vi "WVDIAL_2_OphirPM_v2.2_temp_tune.vi"() -> ()   [LabVIEW 2012]
uses:
  <vilib>/DAQmx/write.llb/DAQmx Write (Digital 1D Bool NChan 1Samp 1Line).vi
  <vilib>/DAQmx/miscellaneous.llb/DAQmx Fill In Error Info.vi
  under_development/AMCS_Data.vi
  <vilib>/Analysis/baseanly.llb/Mean (DBL).vi
  H2O_DIAL/LabVIEW-2012/Scalar_Data.vi
  H2O_DIAL/LabVIEW-2012/Bristol WM V2_31b/CLDevIFace.dll
  <vilib>/Analysis/NI_AALBase.lvlib
panel:
  out "AMCS_Profile":i32=423938
  out "FileHour":i32=21
  out "L_Count":i32=55
  out "sigma_off_total":dbl[](array[numeric])=[4.643764478525789e-25, 4.614054089008885e-25, 4.584505239124867e-25, 4.555117711360031e-25, 4.525891281920628e-25, 4.496825720864026e-25, 4.4679207921346825e-25, 4.43917625363397e-25, 4.410591857279519e-25, 4.382167349086702e-25, 4.353902469221332e-25, 4.325796952070131e-25, 4.297850526319035e-25, 4.270062915003385e-25, 4.2424338355941755e-25, 4.21496300005555e-25, 4.187650114911694e-25, 4.160494881312817e-25, 4.133496995114222e-25, 4.10665614692786e-25, 4.079972022208119e-25, 4.0534443013005885e-25, 4.0270726595130557e-25, 4.0008567671863953e-25, 3.9747962897506563e-25, 3.948890887799126e-25, 3.923140217138123e-25, 3.8975439288624596e-25, 3.872101669423651e-25, 3.8468130806556615e-25, 3.8216777998733165e-25, 3.796695459918264e-25, 3.771865689214647e-25, 3.7471881118146976e-25, 3.7226623474847904e-25, 3.698288011738762e-25, 3.674064715881081e-25, 3.6499920670996217e-25, 3.626069668468178e-25, 3.602297119029483e-25, 3.5786740138468807e-25, 3.555199944025038e-25, 3.531874496780442e-25, 3.508697255483564e-25, 3.4856677996831964e-25, 3.462785705191059e-25, 3.440050544069148e-25, 3.41746188471553e-25, 3.3950192918949573e-25, 3.3727223267433067e-25, 3.350570546849384e-25, 3.3285635062685348e-25, 3.306700755546275e-25, 3.2849818417818464e-25, 3.2634063086181134e-25, 3.2419736963135166e-25, 3.2206835417447437e-25, 3.1995353784347226e-25, 3.178528736595472e-25, 3.1576631431460264e-25, 3.136938121710331e-25, 3.1163531926889047e-25, 3.0959078732359584e-25, 3.0756016773038813e-25, 3.0554341156586187e-25, 3.0354046958827905e-25, 3.0155129224057757e-25, 2.995758296523749e-25, 2.976140316396684e-25, 2.956658477076711e-25, 2.937312270508894e-25, 2.9181011855453255e-25, 2.8990247079637847e-25, 2.8800823204609833e-25, 2.8612735026590936e-25, 2.8425977311370583e-25, 2.824054479409753e-25, 2.8056432179446445e-25, 2.7873634141536925e-25, 2.7692145324124604e-25, 2.751196034045025e-25, 2.733307377340114e-25, 2.7155480175403066e-25, 2.697917406837425e-25, 2.6804149943858566e-25, 2.6630402262774586e-25, 2.6457925455661677e-25, 2.6286713922280107e-25, 2.6116762031845402e-25, 2.594806412296848e-25, 2.5780614503242897e-25, 2.5614407449651105e-25, 2.5449437208048386e-25, 2.5285697993381813e-25, 2.5123183989456577e-25, 2.4961889348824045e-25, 2.4801808192712767e-25, 2.464293461079702e-25, 2.4485262661369243e-25, 2.432878637089962e-25, 2.4173499733996907e-25, 2.401939671334805e-25, 2.3866471239444233e-25, 2.3714717210600145e-25, 2.3564128492636686e-25, 2.3414698918824553e-25, 2.3266422289643866e-25, 2.3119292372725023e-25, 2.2973302902539466e-25, 2.2828447580263785e-25, 2.268472007381932e-25, 2.254211401719836e-25, 2.240062301084126e-25, 2.226024062100116e-25, 2.212096037982056e-25, 2.198277578493862e-25, 2.1845680299420055e-25, 2.170966735142683e-25, 2.1574730334212e-25, 2.1440862605623073e-25, 2.1308057488112046e-25, 2.117630826839664e-25, 2.1045608197172205e-25, 2.0915950489043225e-25, 2.078732832232995e-25, 2.0659734838290317e-25, 2.0533163141598343e-25, 2.0407606299680385e-25, 2.0283057342632226e-25, 2.0159509262467982e-25, 2.0036955013794794e-25, 1.9915387512419972e-25, 1.9794799636048e-25, 1.967518422328947e-25, 1.9556534073675992e-25, 1.9438841947549892e-25, 1.9322100564956178e-25, 1.920630260637019e-25, 1.9091440711521815e-25, 1.8977507479510996e-25, 1.8864495468332108e-25, 1.8752397194377075e-25, 1.8641205132176874e-25, 1.85309117138839e-25, 1.842150932893969e-25, 1.8312990323947193e-25, 1.8205347001558067e-25, 1.809857162063116e-25, 1.7992656395150586e-25, 1.7887593494647524e-25, 1.778337504265391e-25, 1.7679993116519135e-25, 1.7577439747484068e-25, 1.7475706919047535e-25, 1.7374786567250477e-25, 1.7274670579202631e-25, 1.717535079320341e-25, 1.707681899765072e-25, 1.697906693041456e-25, 1.6882086278066873e-25, 1.678586867468332e-25, 1.669040570230428e-25, 1.6595688888336423e-25, 1.650170970602582e-25, 1.6408459573091302e-25, 1.6315929850696558e-25, 1.6224111842310663e-25, 1.6132996793032208e-25, 1.6042575888772121e-25, 1.5952840254274042e-25, 1.5863780952670232e-25, 1.5775388984249963e-25, 1.5687655284818781e-25, 1.5600570725121137e-25, 1.5514126108612298e-25, 1.5428312171529566e-25, 1.534311957966347e-25, 1.5258538929082173e-25, 1.5174560742476717e-25, 1.5091175469739927e-25, 1.5008373485458013e-25, 1.4926145086791297e-25, 1.4844480493302943e-25, 1.4763369844272314e-25, 1.468280319798211e-25, 1.4602770529521724e-25, 1.452326172944243e-25, 1.4444266601595768e-25, 1.4365774862349533e-25, 1.4287776138376983e-25, 1.4210259966100612e-25, 1.4133215788036764e-25, 1.4056632953286864e-25, 1.3980500715375963e-25, 1.3904808229973073e-25, 1.38295445546765e-25, 1.3754698646759526e-25, 1.3680259363191862e-25, 1.36062154573811e-25, 1.3532555580103542e-25, 1.3459268276849692e-25, 1.3386341988195482e-25, 1.3313765048231232e-25, 1.3241525685254664e-25, 1.3169612019618072e-25, 1.3098012064815228e-25, 1.3026713726028247e-25, 1.2955704802645196e-25, 1.2884972986337452e-25, 1.281450586258092e-25, 1.2744290912136427e-25, 1.2674315511209394e-25, 1.2604566934571265e-25, 1.2535032355813504e-25, 1.246569884883568e-25, 1.2396553393298492e-25, 1.2327582875898557e-25, 1.2258774092414679e-25, 1.219011375458982e-25, 1.2121588491226e-25, 1.2053184854101307e-25, 1.1984889325828062e-25, 1.1916688319567769e-25, 1.1848568191243869e-25, 1.178051524299784e-25, 1.1712515731126608e-25, 1.1644555874741191e-25, 1.1576621864375854e-25, 1.1508699868736606e-25, 1.1440776047568059e-25, 1.137283656132748e-25, 1.1304867581494259e-25, 1.1236855301332552e-25, 1.1168785951747307e-25, 1.1100645810052044e-25, 1.1032421216270046e-25, 1.0964098589464416e-25, 1.0895664437392028e-25, 1.0827105377761497e-25, 1.0758408152001282e-25, 1.068955964128544e-25, 1.062054688828481e-25, 1.055135711160854e-25, 1.0481977726805562e-25, 1.0412396366003204e-25, 1.0342600898105731e-25, 1.027257944842442e-25, 1.0202320419826945e-25, 1.0131812517790627e-25, 1.0061044766845727e-25, 9.990006537566844e-26, 9.918687569493606e-26, 9.8470779905946e-26, 9.775168344172793e-26, 9.702949608562794e-26, 9.630413227010019e-26, 9.557551122277968e-26, 9.484355729177786e-26, 9.410820011448697e-26, 9.336937490265801e-26, 9.262702260371961e-26, 9.188109020809214e-26, 9.11315308869798e-26, 9.037830427761936e-26, 8.962137666462638e-26, 8.88607211673616e-26, 8.809631794749932e-26, 8.732815442451108e-26, 8.655622537484813e-26, 8.578053318660534e-26, 8.500108793558888e-26, 8.421790757035365e-26, 8.343101802299517e-26, 8.26404533202396e-26, 8.184625569595185e-26]
  out "sigma_on_total":dbl[](array[numeric])=[1.7075862122244e-23, 1.7004426742837037e-23, 1.693239609744741e-23, 1.6859783954253323e-23, 1.678660410820497e-23, 1.6712870375550727e-23, 1.6638596588086796e-23, 1.656379658679081e-23, 1.6488484214502813e-23, 1.6412673312498138e-23, 1.6336377713340953e-23, 1.625961123487383e-23, 1.6182387675681657e-23, 1.6104720808587064e-23, 1.602662437665621e-23, 1.5948112086218224e-23, 1.586919760240094e-23, 1.5789894545108264e-23, 1.5710216482381445e-23, 1.5630176926607628e-23, 1.5549789329817173e-23, 1.546906707842516e-23, 1.5388023489784623e-23, 1.530667180683284e-23, 1.5225025193879302e-23, 1.5143096734187747e-23, 1.5060899422993675e-23, 1.4978446166673147e-23, 1.4895749777683752e-23, 1.4812822969984015e-23, 1.4729678357888077e-23, 1.464632845041312e-23, 1.4562785649718562e-23, 1.447906224670939e-23, 1.4395170419387456e-23, 1.431112222903883e-23, 1.4226929617854445e-23, 1.4142604406027486e-23, 1.405815829025985e-23, 1.397360284014021e-23, 1.388894949657693e-23, 1.380420957002031e-23, 1.371939423785285e-23, 1.363451454285266e-23, 1.3549581391141818e-23, 1.3464605551189887e-23, 1.3379597651367873e-23, 1.3294568179486758e-23, 1.3209527481194656e-23, 1.312448575787998e-23, 1.3039453067745007e-23, 1.2954439322388221e-23, 1.2869454287169013e-23, 1.2784507581039522e-23, 1.2699608673775678e-23, 1.2614766888406229e-23, 1.252999139774802e-23, 1.2445291225817366e-23, 1.2360675247526299e-23, 1.2276152187304654e-23, 1.2191730619865334e-23, 1.2107418970164145e-23, 1.202322551315382e-23, 1.193915837419463e-23, 1.1855225528683853e-23, 1.177143480262109e-23, 1.1687793873793825e-23, 1.1604310270505038e-23, 1.1520991373461181e-23, 1.1437844415482158e-23, 1.1354876482938843e-23, 1.1272094515594521e-23, 1.1189505307343022e-23, 1.1107115508072479e-23, 1.1024931622616465e-23, 1.094296001379224e-23, 1.0861206901467108e-23, 1.0779678365135314e-23, 1.0698380343367289e-23, 1.06173186361969e-23, 1.0536498905450043e-23, 1.0455926676160623e-23, 1.0375607337759655e-23, 1.0295546145299345e-23, 1.0215748220460876e-23, 1.0136218553593378e-23, 1.0056962003784583e-23, 9.97798330145124e-24, 9.899287048722052e-24, 9.820877721811146e-24, 9.74275967122139e-24, 9.664937124155247e-24, 9.587414185725328e-24, 9.51019484042637e-24, 9.433282953390896e-24, 9.356682271669029e-24, 9.280396426675263e-24, 9.204428935016307e-24, 9.128783200260969e-24, 9.053462513813825e-24, 8.978470057602318e-24, 8.903808904957389e-24, 8.829482022184774e-24, 8.755492270140328e-24, 8.68184240623818e-24, 8.608535085372624e-24, 8.535572861930238e-24, 8.462958191150288e-24, 8.390693430702545e-24, 8.318780842469266e-24, 8.247222593903732e-24, 8.176020759597675e-24, 8.105177323247602e-24, 8.0346941779939e-24, 7.964573129989107e-24, 7.89481589772579e-24, 7.825424115173927e-24, 7.756399332508075e-24, 7.6877430180163e-24, 7.619456559217698e-24, 7.551541264744586e-24, 7.483998365445229e-24, 7.416829016422044e-24, 7.350034297741753e-24, 7.283615216447286e-24, 7.217572707624918e-24, 7.151907636193094e-24, 7.086620797948962e-24, 7.02171292149949e-24, 6.957184668579832e-24, 6.893036636834266e-24, 6.829269359936771e-24, 6.76588330962968e-24, 6.702878896700126e-24, 6.640256472626323e-24, 6.5780163306938516e-24, 6.516158706777594e-24, 6.4546837815950906e-24, 6.3935916809599384e-24, 6.332882477825005e-24, 6.272556192843959e-24, 6.212612795889849e-24, 6.153052207074656e-24, 6.0938742983743955e-24, 6.035078894147427e-24, 5.976665772122362e-24, 5.918634665719597e-24, 5.860985263481029e-24, 5.803717211502671e-24, 5.7468301138902555e-24, 5.6903235336624575e-24, 5.634196994214138e-24, 5.578449979752345e-24, 5.5230819371427534e-24, 5.468092275895874e-24, 5.413480369833808e-24, 5.359245557887875e-24, 5.305387144754368e-24, 5.251904401815032e-24, 5.198796568697882e-24, 5.146062853222409e-24, 5.0937024329285036e-24, 5.041714455530881e-24, 4.9900980398858834e-24, 4.938852277059481e-24, 4.887976230623468e-24, 4.83746893794503e-24, 4.787329410462798e-24, 4.737556635055691e-24, 4.688149574056101e-24, 4.639107166465834e-24, 4.5904283286634496e-24, 4.542111954867825e-24, 4.494156918056621e-24, 4.4465620704066765e-24, 4.399326243957229e-24, 4.352448251589667e-24, 4.305926887428094e-24, 4.259760927133192e-24, 4.213949129056238e-24, 4.168490234607401e-24, 4.12338296883391e-24, 4.07862604077928e-24, 4.034218144353722e-24, 3.990157958768539e-24, 3.946444149064885e-24, 3.9030753664335e-24, 3.860050249023712e-24, 3.817367422335441e-24, 3.7750254995106654e-24, 3.733023082193349e-24, 3.691358760512388e-24, 3.650031114008777e-24, 3.6090387117905654e-24, 3.5683801127861655e-24, 3.528053866803104e-24, 3.488058514122023e-24, 3.4483925866184155e-24, 3.409054607705317e-24, 3.370043092808114e-24, 3.331356549823639e-24, 3.2929934793979014e-24, 3.2549523754474237e-24, 3.217231725253417e-24, 3.179830009805838e-24, 3.1427457044565034e-24, 3.1059772789917302e-24, 3.0695231977134503e-24, 3.033381920449335e-24, 2.99755190191396e-24, 2.962031592850093e-24, 2.9268194397709086e-24, 2.8919138854636326e-24, 2.8573133691808308e-24, 2.8230163268299376e-24, 2.7890211914429353e-24, 2.7553263932755457e-24, 2.7219303599098855e-24, 2.688831516768636e-24, 2.656028287199601e-24, 2.6235190926969376e-24, 2.5913023529850115e-24, 2.5593764866235505e-24, 2.527739910619601e-24, 2.496391041275666e-24, 2.465328293863177e-24, 2.434550083004947e-24, 2.4040548229168003e-24, 2.373840927399175e-24, 2.3439068103705293e-24, 2.314250885433015e-24, 2.284871566748021e-24, 2.2557672684858724e-24, 2.2269364056176892e-24, 2.1983773934884902e-24, 2.170088648470371e-24, 2.1420685877073818e-24, 2.1143156295265137e-24, 2.0868281932439607e-24, 2.059604699720196e-24, 2.0326435711084415e-24, 2.0059432311343632e-24, 1.9795021052597507e-24, 1.9533186205922764e-24, 1.927391206342342e-24, 1.90171829343342e-24, 1.8762983150473395e-24, 1.851129706617593e-24, 1.8262109056432633e-24, 1.8015403521583982e-24, 1.7771164885857278e-24, 1.752937759959652e-24, 1.7290026138301698e-24, 1.705309500565543e-24, 1.6818568732524412e-24, 1.6586431878588544e-24, 1.6356669031809573e-24, 1.6129264812045587e-24, 1.5904203868386669e-24, 1.5681470881088427e-24, 1.5461050562990223e-24, 1.5242927659307277e-24, 1.5027086948226053e-24, 1.481351324147798e-24, 1.4602191385259846e-24, 1.439310626001592e-24, 1.4186242781334644e-24, 1.3981585901500172e-24, 1.3779120607809285e-24, 1.3578831924817317e-24, 1.3380704914055822e-24, 1.3184724673794015e-24, 1.2990876341133162e-24, 1.2799145090715568e-24, 1.2609516136104614e-24]
  out "background start":u32=269
  in  "Tab Control 2":enum32{"WV ND Narrow", "WV ND Wide"}(tab)
  out "Water Vapor Number Density":dbl[][](graph)=[[2.7919549800729766, 2.4721214980617963, 2.1963483034310913, 1.9775481743916468, 2.0259507247493356, 2.096592957954238, 2.09200685333887, 2.201465478284958, 2.172049757701778, 2.066356384667988, 2.1552068146500667, 2.142096979762263, 2.16074094077469, 2.1508543106624907, 2.063657397073414, 2.111120921818043, 1.9736927303840606, 1.9924659617468845, 1.8437447128387863, 1.716666972928834, 1.7329795721179366, 1.6185075270306553, 1.9531692944484582, 1.7270894741211513, 1.3541922429617665, 1.6972365264191616, 1.3780472464601408, 0.6352127824328955, 0.7449848462353037, 0.25739950222857966, 0.02150582751711, 1.2625193726213453, 1.7103366183498547, 1.1760098085538666, 0.952397569112398, 0.9602628838341002, 1.1470709594539148, 2.0260087466607244, 1.717397631037124, 0.45954812101467546, 0.82082018935899, 0.4578051259106563, 0.17693171656260112, 0.2294926614257034, 0.40695379752745414, 0.7260767006490062, 1.6299360111045522, 1.394016861417572, 1.260638353981884, 0.9565154264924587, 0.778518699153623, 1.1018278296017567, 1.9052590216943897, 2.1494434456810643, 3.1852092631635816, 3.50602861686196, 3.114069255143937, 1.9505136425814023, 0.6799674842963526, 1.4884495991309699, -0.13824046213613744, 2.835156534294972, 3.3505695354404685, 2.938366562214755, 6.438557108895117, 0.5183551787975594, 0.3153485302712685, 1.975534410314832, 2.3601361815003115, 5.779543708322931, 5.6862481890886425, -0.320178545767054, -3.752352207701061, -7.1478162896744895, -12.791206630214896, -7.216285577276, -3.118979952580519, 2.676212905498716, -0.09079217678994128, 0.8475995496768057, 7.5565978270016485, 4.031331088945062, 18.746473553929125, 9.019579967521627, 10.111126789878568, 10.911425895546724, 10.881486374798657, -4.867225785195253, 1.3613463436287887, -6.705643508234555, -9.400669767805649, -11.45672530581558, -15.476104692326604, 2.5019067005614284, 22.15558346925288, 12.372906343206774, 9.180179495997407, 10.035886348315783, -2.300504604887407, -6.109257874581613, 1.2443637131026353, 10.72505129453685, 14.876862757116449, -15.670760900032207, -31.77161023736102, -8.91609594784887, -9.583958414687443, -10.704114282385731, 5.617021746201043, 8.71662490415398, 7.943503644326281, 16.20179237317941, -14.236690656943491, 2.957594051298285, 28.71651223843686, -15.16894026062252, -14.342090655059778, -10.145491925129408, -13.950103926886067, -8.362096082265273, -23.276275045469802, -34.21186123581827, -14.624177385211423, 5.1900077381089815, -22.451944969117548, 9.280913616926904, -0.7349242905240464, -1.9056931662673575, -0.3552584964139418, 13.011816088431226, 2.388764514874305, -4.970348772024848, -5.374892740249347, -18.104796179616045, -3.7757407411406834, 0.2572912127569682, -9.101456890736229, -9.940691485699297, -16.220067449273007, -31.360968584433184, -13.22567737321429, 2.9847822496071443, 0.3000737204657703, 14.226487589262792, 6.624487648840693, -27.284491819792123, 24.242667346984188, 19.937023327511973, -6.324539592488602, -2.8041964118578786, 6.740823105858939, 23.587397969477554, -4.2833757162263355, -33.3154285684293, -35.55104995851804, 4.931666571921572, -8.427144388302073, -2.161849941643455, 31.006477690881464, 28.994847381319968, 9.739058874229096, 31.647398824516547, -9.49704103338363, -3.459829626087916, -10.195382957260902, -18.2305351963672, -39.16562759387119, -38.369889060589664, -33.57595009336855, -48.192728659126416, -34.0670225863149, -64.44616828322731, 22.052013009398934, 48.8882374543455, 47.82272047473126, 21.630359864857, 19.619480202360133, 16.248342826014856, 14.55626534124269, 16.14141319559857, 41.72682657704204, 2.358153419284582, -18.450444811942706, -16.453191933989043, -32.77707187251656, 8.079786828047531, -1.1358565341839377, 18.848376232966167, 8.60604014960662, 4.314367560106007, -13.03383243904803, 2.650659064146061, -4.009372086896625, -29.11960106159767, 0.12218354900213305, -39.711017849362754, -42.75783315079344, -30.018182143488808, -9.971368815385215, 31.54378511520024, 37.63564210589476, -76.9833397272995, -131.8510304950383, 39.46780422831733, 23.7601287553926, -35.38738552003143, 32.03435449229545, -19.69485879050221, -3.0917333259606874, -124.46237667041301, -9.002678693930125, 107.01528897422901, 92.48090288243313, -103.79898797554694, -17.675491202491813, 7.874533254057714, 10.524609447658822, 49.75758334212029, 99.07815475479066, 283.5278586000699, 32.971642390852686, -57.450561658578394, 2.4742562020355403, -64.91676229497271, -81.39557989000245, -68.41783168327089, -79.73478237233522, -60.1655084932687, -183.42488156186718, -250.65131530114368, -152.8606608195418, -45.235659006464026, -71.77006522559867, 69.05001410951006, -31.66224852865109, 51.09664282478717, 46.1035128986533, 36.62674413702954, 77.11160259361291, 78.91913357872623, 74.85307061263583, 57.82460870704682, 102.49351870849972, 108.47745264638517, 108.28296843951362, 80.18423693091486, 6.206295215311893, -25.774421868942422, 38.17790600761687, -37.18542234252088, 40.562292077560116, -10.06029995849638, -45.99779659499376, -76.52379698325059, -24.04739599121833, 7.138888554504087, 94.67361862363965, -20.953075063505143, 27.52883005249273, -43.94482761055022, -31.42891116550487, -59.110333442134035, 69.6709781086392, 69.74972907027177, -244.93614676570755, 66.01327113431867, -263.90594662785674, -176.74730262491283, 53.83886185827534, 177.42061263532574, 108.16924852096365, 193.11882731535258, 102.94954292738339, 85.55425867346395, 0.0, 0.0, 0.0, 0.0, 0.0, 0.0]]
  out "Water Vapor Number Density 2":dbl[][](graph)=[[1.9246774090646468, 2.1364801526718655, 2.3563460415698363, 2.437880160037196, 2.4699096457122773, 2.4513779438068592, 2.4212790327062246, 2.4149121010244667, 2.442684765460251, 2.4627579558093378, 2.425720637457262, 2.499208106949827, 2.5487327850901806, 2.416323533000658, 2.503718155028522, 2.6058329726220686, 2.4815743106251458, 2.764613689254371, 2.8761740069495296, 2.9483743931379394, 2.9544743325162677, 3.1794158502671084, 3.1939705775233973, 2.533885225518133, 5.023499890046839, 5.739889326755892, 7.992222757013449, 11.222739860114261, 13.410626739277465, 21.58391327063631, 26.618972753698802, 23.957314589009496, 13.627342397542513, -33.466783552051155, -31.322362431050404, -3.828090312037132, -22.82546710883033, -10.993941851667527, -9.72872074268521, -20.277080950586896, -10.923757163092711, -9.07636230339632, -8.15449746589819, -10.005103572388432, -7.68751749774677, -8.476357917870377, -8.409711355395942, -8.352416737405557, -10.812293275936563, -10.41513555533087, -11.31136062577575, -13.45042937386785, -33.3057348158326, -14.63420336195662, -9.376062674764945, -11.009338696090161, -9.223392851297126, -11.554322192812531, -19.386991636136848, -10.670640131714526, -6.126941067398296, -7.518439774394675, 16.26303016203163, -4.0325693834978615, -2.912247487056353, 2.439455899744925, 1.3136310339215345, 7.53017468726898, 19.354503059461745, 10.874858416208898, 5.884842201842596, 11.658075090740155, 10.63840673688868, 11.819813138077537, 7.821749325303154, 6.142757151705678, 5.990511287239049, 6.091428632318514, 4.133829631016586, 1.910373740863632, 2.812138534703024, 0.13240697681270577, -1.6539863211154304, 1.8124465284545117, -0.10209803300606486, 0.3873834385336532, 3.2825127417538034, -0.38206784826885704, 0.29108793649235654, 1.9734986497673108, 2.709688975560919, 3.937758253159303, 6.073548367509126, 5.57827633674878, 3.7256924825272715, 3.523348344651393, 2.1380698550049098, 0.9819285118748023, 0.7534956053683336, 1.958752445947795, 1.167700425578407, 2.821741044082525, 1.7904903289201626, -0.06699506335081942, 2.0828772273760388, 1.5528809734202558, -1.4814454333788867, -0.7987225616089674, -2.386278740227717, -4.10627162811292, 0.7960841223175821, -0.967223151556819, -2.7068052187970837, -0.8793538769734781, -1.6058994738614338, -1.153786976051838, -0.3772533844763944, -0.8321700075992845, 0.44162594879454903, 1.6775161023774172, 0.6144603786142944, 1.4748523477090723, 2.4261191491083633, -2.1637504157741003, -3.389739107572159, -1.336259563239183, 1.9457781147812288, 7.382876566090144, 7.012454908750662, 3.1710680875691533, -1.4266581436017785, -1.990855306154264, 1.8513905052490254, 6.224985812056048, 6.783669358850058, 2.503269835114906, 2.526890697902952, -0.15272259761902673, 1.166363050044734, 6.816656964463991, 5.817625584065743, 4.99042666662815, 5.578758228379871, 5.316718150893578, 2.2279403560959765, 3.6626378977623295, -2.7379426603799293, -4.168325740386166, -6.125245341748409, -5.986492361721819, -5.554924977572535, -4.33933044932571, -4.5079301433076795, -8.557458906008524, -5.194267813260687, -2.290162360446739, 3.189747404419548, 8.255852252066553, 9.969917789546885, 7.289797314084266, 4.129672688789654, 1.5019653264394026, 4.035196023759196, 3.620172660102847, 19.014751858086527, 6.4140881220414885, 1.6078436888032817, -4.9127663382774704, -13.431807716867139, -4.920859019873842, 0.11545557487235945, -2.418236722549294, -12.138276953308633, -13.944911735185746, -38.40034011695379, -12.768978114170004, -10.98559210913547, -8.071653207468731, 13.296674504094893, -6.570530262352096, 2.05649815926914, 0.27410650933140895, -7.566197720766897, 3.244758690591443, 11.479395171418595, -7.161105508606986, 12.337200345292445, 7.436389297750922, -2.8867984076459487, 26.508322141770208, -8.578118700603605, -4.812022100008427, 3.533689345937024, -8.142214281133004, 2.5937233186038475, 9.186142836001329, -15.684712280988862, -4.636866364119136, -7.5203674360960395, -21.093456852627572, 26.245939225341598, 32.12889135174122, 30.211214706937447, 49.64772783624668, 27.87193220400699, 8.478543192420785, 7.300517871932979, -11.241261216539064, -6.755589509893532, 0.1754162141842197, -40.87967308128872, -30.777993550416333, -25.110900077730392, -40.53025335927562, -16.147889968195557, -5.849042580416056, -42.062440862797764, -40.9461177020024, -48.30500611043761, -32.69072054873273, 4.3684891317049805, 40.5333176218133, 44.48163269384392, 16.266173328134716, -1.4034575775621692, -13.732735958483435, 35.50263552659409, 88.77461883984728, 65.81909954799848, 46.01099724751913, 29.966703800722787, -32.222515144215095, -39.001218416158856, -45.89663062841511, 10.24466871719786, 50.268932259400195, -121.68095976928211, -105.29974840543122, -56.18445992064484, -67.42947981632405, -15.455237158470073, 268.98749589285126, 208.26441201100153, 162.76795471812062, 1.9734940437567248, -218.48392140256198, 105.85362620395831, -64.0037301624681, -2.898047398837785, 21.380458202422382, 52.06570549270102, -248.8417906380732, -392.7522320975338, -215.35790079570805, 86.30117929847647, 159.14973379695226, 49.766972938901, 141.48970735229034, 1.7362457533596822, -0.14859597277129066, -98.66855973524312, 66.47378697642905, 236.04063498719637, 18.599802555423434, -99.43534896876382, 102.65886550601961, 73.36634300545326, -52.794667338550894, 36.1390490700412, 17.94640810403047, 34.13997149679165, -102.74220223926922, -65.7599054547175, 57.26872729966095, 0.0, 0.0, 0.0, 0.0, 0.0, 0.0]] caption="Water Vapor Number Density"
  out "RingBuffer offline near":dbl[][](array[numeric])
  out "RingBuffer aerosol near":dbl[][](array[numeric])
  in  "LOWER DISPLAY TAB":T1(tab)
  out "NRB":dbl[][](graph)=[[-3.800229408179693, -3.06314471671871, -2.586395001932205, -2.231941202363951, -1.9477207314219656, -1.7167397393646742, -1.5262035572526398, -1.364937464827194, -1.229462730809553, -1.118344000034183, -1.0283656358510886, -0.9561701019361557, -0.9025135206001915, -0.8627761462819167, -0.8360063278396849, -0.8198158981197357, -0.8061970293623525, -0.7877547408903874, -0.761226082248506, -0.7318531575391255, -0.7043247843183529, -0.6856829368303268, -0.6774945269892939, -0.6780969120898757, -0.6855795172986112, -0.697357082303388, -0.7090931326438995, -0.719243815964618, -0.7301383219859523, -0.7340834310039841, -0.7411956864780824, -0.7410369821935734, -0.7389788255998272, -0.7411397471378939, -0.7349219768039156, -0.7383642102319196, -0.7346077084773024, -0.7383309135731002, -0.7404822097283869, -0.7400029405093289, -0.7403653644838679, -0.7398416855657998, -0.7495371647323372, -0.7507436529256251, -0.7628558778510316, -0.7744574009887791, -0.772092035038182, -0.7826605939835732, -0.7906350425190564, -0.7911167128231053, -0.8047257605935517, -0.8208185277520433, -0.8319646227700381, -0.8377364399653591, -0.8425989844040539, -0.8513709082209938, -0.8614177662910704, -0.8912920570377314, -0.9248282024330806, -0.9432974574531058, -0.9415412810401951, -0.9310482734359397, -0.9338475158110462, -0.9134126868959206, -0.9283159986479004, -0.9145357579604514, -0.8898714875211668, -0.8875119944449646, -0.8828395041020582, -0.8987158344231726, -0.9189036361912808, -0.9646903803671855, -1.012629192189445, -1.04810081341131, -1.0803705713954739, -1.0793488392821509, -1.0810325197637765, -1.0860051215689395, -1.0919950348359535, -1.0970130303750192, -1.10050408499005, -1.1270957243331732, -1.153978655576542, -1.1759114974466267, -1.1814224007579102, -1.1478719628952656, -1.0881989873342564, -1.0434132693286031, -1.0423709416923355, -1.003167618084612, -1.0073219251996215, -1.0202371044894711, -1.0152974092249483, -1.1107576533946732, -1.1218686377231266, -1.2137096270649306, -1.2667171397873895, -1.1892934301718043, -1.195811506977401, -1.0821539130490045, -1.060475648708257, -1.0960067322895548, -1.1045852070482358, -1.205075147723515, -1.1710054544711102, -1.2279788860580556, -1.2235093993119002, -1.1920092242575382, -1.1837115303455092, -1.172287896788179, -1.246471942306521, -1.163648031500021, -1.084657739777487, -1.0421989912294563, -1.031853699648537, -1.1138724762093004, -1.1962195579732187, -1.2789690855557603, -1.2013419086769594, -1.1984463292291385, -1.2347319589311334, -1.0914307352170172, -1.119133066161212, -1.0951251916722085, -1.0796012629942673, -1.1660709765933723, -1.121190131602695, -1.1021885815228185, -1.1162886426649374, -1.1518589012525402, -1.235429403749575, -1.3843132921113361, -1.4984585580111909, -1.1477154649207388, -1.1408513656392523, -1.0889991084647108, -1.0498968077168733, -1.2217489272096793, -1.147493708380524, -1.1048199722886152, -1.0906745215855211, -1.1616096714779933, -1.231523831555943, -1.2084113515707662, -1.0485969917388265, -1.0028476315868609, -0.908153785166785, -0.9593826358961169, -1.1485410157950036, -1.1805752730290044, -1.4613637167632942, -1.5831274616304676, -1.8524697361245794, -1.902893297328939, -1.787245904046182, -1.9469806297270116, -2.4348078969799545, -1.5452467790031763, -1.5555715396865895, -1.6046204481754156, -1.4808715626314377, -1.3616849023984043, -1.2044986712945338, -1.0728427396250597, -1.1368391398220103, -1.102541352977231, -1.188264259019151, -1.2087675203831756, -1.0898031784234676, -1.0938247007935697, -0.9835556291746889, -0.9904433581700574, -1.0522941045778185, -1.0560752229787496, -1.2348032828788582, -1.334713764526752, -1.1978469831217804, -1.3608491709347206, -1.0667022430489146, -0.9399106674612636, -0.9876858594604188, -0.9662967753493834, -1.0825798056847127, -1.3239312272664043, -1.2163301583978723, -1.3333345454057624, -1.4132217678519643, -1.4325731565341893, -1.326699507831265, -1.1895532512336644, -1.357146633255645, -1.1092647584015825, -1.405175209074444, -2.071325145827588, -1.7178623977929357, -2.519985049968918, -1.8650910351271313, -1.1573432346808377, -0.9007453282372851, -0.8538828666401298, -0.8669195966399774, -1.0140790767546946, -1.4217368261424512, -1.0249565405120962, -0.9192498069458324, -0.842713087225846, -0.9210522507407414, -1.1768630172734111, -1.2843024988594796, -1.9010322059685716, -1.2202092243334877, -1.766166903525135, -2.203531076343693, -3.514732758163316, -1.1658588717362406, -2.8174425613600427, -1.7252934585275521, -1.4158596591803272, -1.0661722234590856, -1.3922611378291887, -1.8065419289783404, -2.012215811399121, -2.9418314791168347, -2.1050247884394424, -1.574790059832753, -2.077194149612097, -2.1648977087631036, -1.5196154156533368, -1.177386185168425, -1.0008246644603354, -1.1775246202068392, -1.1202978755017272, -1.044063384440292, -0.9858486216752352, -0.9637605673447708, -1.2184346489813616, -1.1987451492339647, -1.5260011819424544, -1.2610700135891226, -0.9215963998960293, -1.113154617357813, -1.1475896753447852, -1.1756020903233884, -1.7256144841358523, -1.5689993243779985, -1.4104165618981157, -1.3146217250936891, -1.5819863632077438, -1.0933708340070682, -1.2071394021218131, -1.2102078003428727, -1.184296563243633, -1.2357777799638099, -1.1743147216259175, -1.380206899498629, -1.447625287732161, -1.2721141475668638, -2.6438056872192366, -1.0704576216856974, -1.828565053490517, -1.3540195684640588, -1.211855498018374, -0.965407575543998, -1.5884933767947966, -1.0531141070130239, -0.9156713028909425, -0.8100547333672709, -1.3031843902511135, -1.3165366769540703, -1.4320177541670616, -1.6886772033069095, -1.5758186382249717, -1.1421971851539605, -1.1508373970493577, -1.690035290867579, -inf, -inf, -inf, -inf, -inf]] caption="Water Vapor Number Density"
  out "NRB 2":dbl[][](graph)=[[-3.0395188028357603, -2.3233310980260935, -1.908420723106076, -1.6302908440291224, -1.4282319836990602, -1.2744401657701292, -1.1539937154087423, -1.05853929608012, -0.9834427908474358, -0.9283287518597617, -0.8863581265636199, -0.8577551770624776, -0.8428705414502229, -0.8373210856679418, -0.8447938776035089, -0.8587365448043809, -0.873883515771329, -0.8813689723007432, -0.8774795693013318, -0.8677747815053004, -0.8600600847719546, -0.8595431314342655, -0.8681841305661355, -0.885390456771323, -0.9199774671108429, -0.9523346307996355, -0.9887639986348082, -1.0160536970759566, -1.0377506342413638, -1.0575136619828756, -1.0724721099288403, -1.1081309920793745, -1.114135072852424, -1.1355512982105995, -1.1392677172713934, -1.1467863183669873, -1.1658943701620241, -1.188161442926748, -1.2069892676099805, -1.2074612515550163, -1.2430546003808078, -1.2300970883816922, -1.298830352045476, -1.358703266826767, -1.3248852909188416, -1.3860187725636977, -1.3972398422909322, -1.4554774841562164, -1.5178491030527048, -1.564110781795938, -1.6220897936161092, -1.5208969542258364, -1.454348655100703, -1.4405921579344618, -1.4615070162429147, -1.4951291443274128, -1.7319565361894438, -1.969627795218796, -2.0771765277122363, -2.328544428787139, -1.8601381790747755, -1.8951962653608625, -1.7793115109813733, -2.255357804818516, -2.902967799437367, -2.421844110716655, -1.886647282120273, -2.0371230826274975, -2.1296353890888784, -2.203475639570752, -2.5685712448217277, -2.0033420248153524, -2.6169900639957655, -1.927542690509862, -1.405873961597174, -1.3259638684638195, -1.3539550277695553, -1.4242408794322738, -1.468918201419294, -1.4538280602853981, -1.3954212501136907, -1.305232269627442, -1.3344630238732782, -1.4740737469258944, -1.348804310360201, -1.5001521126592026, -1.389640446498644, -1.2250901251967545, -1.2913755968283593, -1.1235122884102886, -1.1483390918357013, -1.146495387943153, -1.1508242258903185, -1.229521881558638, -1.3304819849086533, -1.4452755544135947, -1.2762251214476263, -1.188234794912964, -1.0272788934356993, -1.0561195464317779, -1.1755054918408905, -1.1901794946288025, -1.331092466379116, -1.3164567545394104, -1.3490261692585808, -1.3440099621319015, -1.2577528142307361, -1.2561268962359338, -1.1410008073837692, -1.0676552929420373, -1.0705065775440905, -0.9949654137895192, -0.9602649895110492, -0.9858900749888218, -1.0894067873465203, -1.00682512703767, -1.0243095421701527, -0.9262744207006681, -1.0124226618520726, -0.9852318793179309, -1.0545828719090762, -1.3309862870720164, -1.0873613373156128, -1.41157121686751, -1.2176731494363078, -1.543541430165227, -1.6266424343497268, -1.4411568122747527, -1.4038460927505363, -0.9525486962136351, -0.9710054049772678, -0.830230618685657, -0.9424523281840133, -0.8645246633140569, -0.8732983037287279, -1.0361607688951742, -0.8809275494921459, -1.0428741462471849, -0.8257052431138743, -0.7570678364375087, -0.8810124231548133, -0.9287378561861365, -0.9616461089243693, -1.0505251112482314, -0.9753015586967972, -0.8760595689715901, -0.9203697595905868, -1.116959300554274, -1.0757393471096224, -1.2481722985000652, -1.6419601507423385, -1.210873281443344, -1.1566809666728644, -1.1235066614230336, -0.9662288978872197, -0.8655480583717805, -1.0243341460745388, -1.0695996474203173, -0.9473647012757251, -1.2272006224470273, -1.5656156624047448, -0.8838816613406753, -0.8131352902229119, -0.5883525803118183, -0.44705190910656667, -0.4873783352928001, -0.697030801218704, -0.8529471636503854, -0.7888217180943793, -0.9796596082035468, -0.6965771991231455, -0.6863397287202919, -0.704343194569718, -0.6983521519003736, -0.75482060215265, -0.8265077372261195, -0.9366095532244315, -1.3096368128120366, -1.55523088529547, -1.051374191523295, -1.0134466624297098, -0.7165252825776682, -0.6877544777857888, -0.7294851994483913, -0.7071201854733108, -0.792240532611032, -0.8216762298728549, -0.8316234970712869, -1.183308004710733, -1.2014672707579863, -1.3930671714776368, -2.558789782326539, -1.0221680070974872, -0.7480559331584905, -0.5974185950939364, -0.4775717144571013, -0.6171381393317891, -0.8313691001778754, -0.9955764722936213, -1.0527813017046717, -0.6033543602819839, -0.5290594479150054, -0.43524397052742386, -0.37679335183244894, -0.5162544646967443, -0.47135181420500616, -0.7167633775590044, -0.7407021630217935, -0.8597964624753381, -1.1734621711320692, -0.7688427227470973, -1.669945647531002, -1.3431548384512018, -2.066624363320553, -1.654336929725225, -0.8971846990069086, -1.013146177970888, -1.5734198083696587, -1.8822121408274337, -2.0694797328117005, -1.1185490231931678, -0.6818046448015959, -0.9037450905151062, -1.9477758044580327, -1.9586300403215469, -1.0289019449660306, -0.5713708094925551, -0.439195873307232, -0.4029292512642405, -0.4611900196568202, -0.9660070139599247, -0.69589168199642, -1.2102712213870142, -1.3891355286097515, -1.214467865809061, -2.1242955574673843, -0.7547284262543583, -0.7392845638966377, -0.780333238537859, -0.6398868140073373, -1.273219658057857, -1.7242941865417751, -1.1638448909447319, -0.6533727995881398, -1.2415473713943328, -1.246609551185947, -1.1510733702051754, -0.5871513490306304, -0.6930188537604239, -0.44586737411491756, -0.4336888079832172, -0.5143941610715134, -0.5453776795196447, -0.6326882983211548, -0.8931884033565821, -0.7723614430752257, -0.9372443197274739, -1.178304247434384, -0.7218840491245596, -0.8616817347228367, -0.7209931344792607, -1.034721576384339, -0.7559150388452325, -0.8138309771345489, -1.0614132301942103, -0.6058575709955408, -0.4737327477542772, -0.8142841054573958, -1.3092373775920507, -1.0968241652288904, -0.8305038352815278, -1.2854410336523954, -0.5782161423596848, -1.3387354637076283, -1.116390408215631, -inf, -inf, -inf, -inf, -inf]] caption="Water Vapor Number Density"
  out "raw counts":dbl[][](graph)=[[64.89999999999998, 127.89999999999998, 149.89999999999998, 225.89999999999998, 299.9, 364.9, 367.9, 511.9, 588.9, 656.9, 762.9, 717.9, 757.9, 722.9, 691.9, 601.9, 558.9, 415.9, 441.9, 443.9, 372.9, 443.9, 423.9, 406.9, 339.9, 291.9, 282.9, 260.9, 225.89999999999998, 210.89999999999998, 169.89999999999998, 117.89999999999998, 138.89999999999998, 158.89999999999998, 165.89999999999998, 140.89999999999998, 132.89999999999998, 119.89999999999998, 84.89999999999998, 105.89999999999998, 103.89999999999998, 96.89999999999998, 96.89999999999998, 90.89999999999998, 119.89999999999998, 68.89999999999998, 98.89999999999998, 58.89999999999998, 41.89999999999998, 59.89999999999998, 34.89999999999998, 55.89999999999998, 28.899999999999977, 64.89999999999998, 18.899999999999977, 62.89999999999998, 44.89999999999998, 52.89999999999998, 58.89999999999998, 29.899999999999977, 63.89999999999998, 2.8999999999999773, 3.8999999999999773, 48.89999999999998, 43.89999999999998, 13.899999999999977, 20.899999999999977, 5.899999999999977, 34.89999999999998, 19.899999999999977, -9.100000000000023, 9.899999999999977, 30.899999999999977, 17.899999999999977, -2.1000000000000227, 29.899999999999977, 4.899999999999977, 34.89999999999998, 11.899999999999977, -1.1000000000000227, -7.100000000000023, -5.100000000000023, -11.100000000000023, 2.8999999999999773, 6.899999999999977, -3.1000000000000227, 19.899999999999977, 13.899999999999977, 13.899999999999977, 12.899999999999977, 12.899999999999977, 24.899999999999977, 38.89999999999998, -26.100000000000023, 0.8999999999999773, 19.899999999999977, 38.89999999999998, 11.899999999999977, 8.899999999999977, 36.89999999999998, 11.899999999999977, -12.100000000000023, -15.100000000000023, -3.1000000000000227, -8.100000000000023, -7.100000000000023, 14.899999999999977, 1.8999999999999773, -9.100000000000023, -21.100000000000023, -6.100000000000023, 12.899999999999977, 5.899999999999977, -9.100000000000023, 34.89999999999998, 16.899999999999977, -7.100000000000023, 30.899999999999977, 8.899999999999977, 24.899999999999977, 33.89999999999998, 15.899999999999977, 3.8999999999999773, 36.89999999999998, -18.100000000000023, 4.899999999999977, -12.100000000000023, 14.899999999999977, 11.899999999999977, -10.100000000000023, -27.100000000000023, 6.899999999999977, 3.8999999999999773, 3.8999999999999773, 11.899999999999977, 2.8999999999999773, 32.89999999999998, -12.100000000000023, 6.899999999999977, 14.899999999999977, -11.100000000000023, 24.899999999999977, 4.899999999999977, -38.10000000000002, 34.89999999999998, -21.100000000000023, -1.1000000000000227, -13.100000000000023, -12.100000000000023, 5.899999999999977, 26.899999999999977, -8.100000000000023, -0.10000000000002274, -16.100000000000023, -22.100000000000023, 12.899999999999977, 11.899999999999977, 28.899999999999977, -13.100000000000023, -9.100000000000023, -3.1000000000000227, -32.10000000000002, 32.89999999999998, 16.899999999999977, 0.8999999999999773, 9.899999999999977, 7.899999999999977, 28.899999999999977, 9.899999999999977, -6.100000000000023, 15.899999999999977, -10.100000000000023, 18.899999999999977, 23.899999999999977, -15.100000000000023, 23.899999999999977, -23.100000000000023, 12.899999999999977, 18.899999999999977, -3.1000000000000227, -11.100000000000023, -30.100000000000023, -25.100000000000023, 5.899999999999977, -0.10000000000002274, -23.100000000000023, 20.899999999999977, 4.899999999999977, 19.899999999999977, 13.899999999999977, 1.8999999999999773, 14.899999999999977, -3.1000000000000227, 57.89999999999998, 13.899999999999977, -1.1000000000000227, -12.100000000000023, -8.100000000000023, 10.899999999999977, -14.100000000000023, -24.100000000000023, -16.100000000000023, -3.1000000000000227, 6.899999999999977, -14.100000000000023, -18.100000000000023, -6.100000000000023, 5.899999999999977, 3.8999999999999773, 0.8999999999999773, 6.899999999999977, -1.1000000000000227, -6.100000000000023, -8.100000000000023, -0.10000000000002274, 9.899999999999977, -20.100000000000023, 9.899999999999977, 4.899999999999977, 29.899999999999977, -15.100000000000023, 2.8999999999999773, -26.100000000000023, -2.1000000000000227, 6.899999999999977, -16.100000000000023, -17.100000000000023, -15.100000000000023, -36.10000000000002, -24.100000000000023, -17.100000000000023, 18.899999999999977, -3.1000000000000227, -22.100000000000023, -12.100000000000023, 5.899999999999977, -20.100000000000023, 31.899999999999977, 3.8999999999999773, -0.10000000000002274, 30.899999999999977, 12.899999999999977, -20.100000000000023, -5.100000000000023, 17.899999999999977, -1.1000000000000227, -10.100000000000023, -30.100000000000023, 4.899999999999977, -3.1000000000000227, 9.899999999999977, 12.899999999999977, -14.100000000000023, -38.10000000000002, 7.899999999999977, -0.10000000000002274, -5.100000000000023, -24.100000000000023, 3.8999999999999773, -5.100000000000023, -11.100000000000023, 5.899999999999977, -1.1000000000000227, -8.100000000000023, -13.100000000000023, -8.100000000000023, -13.100000000000023, 3.8999999999999773, 3.8999999999999773, 29.899999999999977, 1.8999999999999773, -4.100000000000023, -22.100000000000023, 20.899999999999977, 4.899999999999977, -12.100000000000023, 1.8999999999999773, -18.100000000000023, -3.1000000000000227, 0.0]] caption="Water Vapor Number Density"
  out "raw counts near":dbl[][](graph)=[[330.29999999999995, 680.3, 879.3, 1114.3, 1303.3, 1233.3, 1310.3, 1335.3, 1304.3, 1170.3, 1044.3, 1129.3, 817.3, 849.3, 628.3, 550.3, 507.29999999999995, 330.29999999999995, 297.29999999999995, 291.29999999999995, 341.29999999999995, 223.29999999999995, 280.29999999999995, 290.29999999999995, 226.29999999999995, 162.29999999999995, 191.29999999999995, 182.29999999999995, 94.29999999999995, 62.299999999999955, 90.29999999999995, 69.29999999999995, 56.299999999999955, 80.29999999999995, 10.299999999999955, 26.299999999999955, 57.299999999999955, 34.299999999999955, 28.299999999999955, 52.299999999999955, 44.299999999999955, 44.299999999999955, -4.7000000000000455, 58.299999999999955, 36.299999999999955, 7.2999999999999545, 34.299999999999955, 61.299999999999955, 26.299999999999955, 40.299999999999955, 45.299999999999955, -34.700000000000045, 19.299999999999955, -20.700000000000045, -47.700000000000045, 27.299999999999955, 26.299999999999955, 74.29999999999995, 31.299999999999955, 3.2999999999999545, -7.7000000000000455, -0.7000000000000455, -50.700000000000045, -10.700000000000045, -19.700000000000045, 44.299999999999955, 75.29999999999995, -59.700000000000045, -53.700000000000045, -57.700000000000045, 3.2999999999999545, 10.299999999999955, 24.299999999999955, 32.299999999999955, 47.299999999999955, -51.700000000000045, 13.299999999999955, 6.2999999999999545, -65.70000000000005, 13.299999999999955, -13.700000000000045, -1.7000000000000455, -33.700000000000045, -33.700000000000045, -56.700000000000045, -42.700000000000045, 4.2999999999999545, -38.700000000000045, -23.700000000000045, 47.299999999999955, -38.700000000000045, -34.700000000000045, 15.299999999999955, -71.70000000000005, 44.299999999999955, -31.700000000000045, -35.700000000000045, 35.299999999999955, -3.7000000000000455, -31.700000000000045, 36.299999999999955, -41.700000000000045, 27.299999999999955, -20.700000000000045, 16.299999999999955, -75.70000000000005, 12.299999999999955, -83.70000000000005, -4.7000000000000455, 15.299999999999955, 46.299999999999955, -7.7000000000000455, -98.70000000000005, -50.700000000000045, -9.700000000000045, -42.700000000000045, -73.70000000000005, -42.700000000000045, 3.2999999999999545, -27.700000000000045, -28.700000000000045, -13.700000000000045, -37.700000000000045, -4.7000000000000455, -12.700000000000045, -20.700000000000045, -23.700000000000045, -20.700000000000045, 12.299999999999955, -37.700000000000045, 40.299999999999955, -37.700000000000045, -10.700000000000045, -37.700000000000045, 1.2999999999999545, -8.700000000000045, -46.700000000000045, -55.700000000000045, -87.70000000000005, 5.2999999999999545, 28.299999999999955, -63.700000000000045, -41.700000000000045, 18.299999999999955, -25.700000000000045, -27.700000000000045, 69.29999999999995, -48.700000000000045, -29.700000000000045, -2.7000000000000455, -8.700000000000045, -17.700000000000045, -7.7000000000000455, -50.700000000000045, 19.299999999999955, 15.299999999999955, 2.2999999999999545, -74.70000000000005, 4.2999999999999545, 3.2999999999999545, -138.70000000000005, 17.299999999999955, 31.299999999999955, -53.700000000000045, 16.299999999999955, 5.2999999999999545, -17.700000000000045, -9.700000000000045, -99.70000000000005, -140.70000000000005, 56.299999999999955, -68.70000000000005, 31.299999999999955, -27.700000000000045, 7.2999999999999545, 2.2999999999999545, -8.700000000000045, -22.700000000000045, 67.29999999999995, 21.299999999999955, -5.7000000000000455, -4.7000000000000455, -52.700000000000045, 19.299999999999955, -41.700000000000045, -126.70000000000005, 59.299999999999955, -66.70000000000005, -15.700000000000045, -6.7000000000000455, -55.700000000000045, 12.299999999999955, 56.299999999999955, -23.700000000000045, -34.700000000000045, -23.700000000000045, -48.700000000000045, -7.7000000000000455, -34.700000000000045, 21.299999999999955, 22.299999999999955, 18.299999999999955, 13.299999999999955, 15.299999999999955, -49.700000000000045, -47.700000000000045, 25.299999999999955, -97.70000000000005, -27.700000000000045, -20.700000000000045, -18.700000000000045, -35.700000000000045, -32.700000000000045, -4.7000000000000455, -41.700000000000045, -23.700000000000045, -34.700000000000045, -25.700000000000045, -10.700000000000045, 53.299999999999955, -60.700000000000045, 67.29999999999995, -15.700000000000045, 33.299999999999955, -33.700000000000045, 42.299999999999955, -44.700000000000045, -80.70000000000005, 62.299999999999955, 30.299999999999955, 38.299999999999955, -3.7000000000000455, -55.700000000000045, -2.7000000000000455, -9.700000000000045, 20.299999999999955, -3.7000000000000455, 1.2999999999999545, -50.700000000000045, -29.700000000000045, -18.700000000000045, 2.2999999999999545, -27.700000000000045, -15.700000000000045, -1.7000000000000455, 7.2999999999999545, -17.700000000000045, -61.700000000000045, -57.700000000000045, -15.700000000000045, -9.700000000000045, 6.2999999999999545, -39.700000000000045, 21.299999999999955, -33.700000000000045, -38.700000000000045, -17.700000000000045, 10.299999999999955, -25.700000000000045, 1.2999999999999545, -19.700000000000045, -39.700000000000045, 3.2999999999999545, -43.700000000000045, -30.700000000000045, 34.299999999999955, -45.700000000000045, -37.700000000000045, -30.700000000000045, -45.700000000000045, -3.7000000000000455, -32.700000000000045, -11.700000000000045, 27.299999999999955, 14.299999999999955, -3.7000000000000455, -9.700000000000045, -38.700000000000045, 104.29999999999995, 0.0]] caption="Water Vapor Number Density"
  out "Aerosol Smoothed 2":dbl[](array[numeric])=[796.9473684210525, 1034.6151315789473, 1193.9440789473683, 1273.4309210526317, 1297.5822368421054, 1284.1282894736844, 1245.342105263158, 1188.3552631578946, 1116.7927631578946, 1027.694078947368, 936.1578947368419, 840.7894736842103, 741.9440789473682, 648.4210526315788, 555.5986842105262, 473.1842105263157, 404.99342105263145, 355.203947368421, 321.7467105263157, 296.99342105263156, 274.25657894736844, 250.233552631579, 224.4802631578948, 198.19407894736847, 168.71052631578948, 144.8092105263158, 123.49671052631581, 107.85197368421055, 95.65131578947373, 85.41118421052636, 77.28618421052634, 66.81907894736844, 61.97039473684211, 55.57236842105263, 51.99671052631578, 48.30592105263157, 43.763157894736835, 39.41776315789473, 35.835526315789465, 34.02960526315788, 29.842105263157883, 29.299342105263143, 23.861842105263147, 19.855263157894726, 20.519736842105253, 17.059210526315777, 15.924342105263147, 13.351973684210515, 11.098684210526304, 9.582236842105251, 8.059210526315779, 9.786184210526304, 10.980263157894726, 10.917763157894726, 10.029605263157883, 8.95394736842104, 5.009868421052619, 2.799342105263146, 2.1118421052631455, -1.144736842105275, -3.256578947368433, -2.9078947368421173, -3.6776315789473806, -1.1907894736842228, 0.2598684210526195, 0.76315789473683, 2.539473684210514, 1.743421052631567, -1.3684210526315912, -1.1217105263158014, -0.4703947368421173, -1.6809210526315912, 0.39802631578946146, -1.8947368421052753, -6.131578947368434, -7.177631578947381, -6.555921052631591, -5.434210526315802, -4.779605263157907, -4.825657894736855, -5.384868421052644, -6.467105263157907, -5.9013157894736965, -4.177631578947381, -5.444078947368433, -3.7532894736842226, -4.730263157894749, -6.753289473684223, -5.667763157894749, -8.157894736842117, -7.5361842105263275, -7.404605263157906, -7.17434210526317, -5.858552631578959, -4.546052631578959, -3.4177631578947487, -4.940789473684223, -5.92763157894738, -8.414473684210538, -7.717105263157906, -5.746710526315802, -5.447368421052643, -3.86184210526317, -3.9177631578947487, -3.565789473684223, -3.539473684210538, -4.23684210526317, -4.17434210526317, -5.342105263157907, -6.210526315789486, -6.059210526315802, -7.082236842105275, -7.5361842105263275, -6.980263157894749, -5.404605263157907, -6.42434210526317, -6.065789473684223, -7.4736842105263275, -6.0263157894736965, -6.309210526315802, -5.289473684210538, -2.753289473684223, -4.746710526315802, -2.213815789473696, -3.404605263157907, -1.5822368421052755, -1.286184210526328, -1.9407894736842226, -2.0822368421052753, -5.796052631578959, -5.470394736842118, -7.450657894736854, -5.667763157894749, -6.680921052631591, -6.450657894736853, -4.368421052631591, -6.154605263157906, -4.177631578947381, -6.789473684210538, -7.8388157894736965, -5.809210526315801, -5.131578947368433, -4.690789473684223, -3.7697368421052753, -4.421052631578959, -5.480263157894749, -4.881578947368433, -3.0625000000000115, -3.322368421052644, -2.2039473684210646, -0.8782894736842225, -2.338815789473696, -2.6151315789473806, -2.7861842105263275, -3.950657894736854, -4.917763157894749, -3.3684210526315908, -2.996710526315801, -3.9210526315789593, -2.0328947368421173, -0.9210526315789591, -4.371710526315801, -5.082236842105275, -8.42434210526317, -11.523026315789487, -10.375000000000012, -6.325657894736853, -4.365131578947381, -5.0000000000000115, -3.1842105263158014, -6.039473684210538, -6.11184210526317, -5.796052631578959, -5.809210526315801, -5.042763157894749, -4.226973684210538, -3.243421052631591, -1.3585526315789598, -0.7631578947368542, -2.4078947368421173, -2.598684210526328, -5.092105263157907, -5.381578947368434, -4.835526315789486, -5.0361842105263275, -4.095394736842118, -3.786184210526328, -3.661184210526328, -1.6118421052631697, -1.529605263157907, -0.9736842105263278, 0.06578947368419855, -2.2401315789473806, -4.167763157894749, -5.835526315789486, -7.611842105263169, -5.463815789473696, -3.3026315789473806, -2.2401315789473806, -1.9440789473684328, -5.417763157894749, -6.365131578947381, -7.822368421052643, -8.86184210526317, -6.365131578947381, -6.990131578947381, -3.934210526315801, -3.687500000000012, -2.776315789473696, -1.3355263157894857, -3.3585526315789593, 0.41776315789472496, -0.8782894736842225, 0.16447368421051445, -0.42105263157895934, -2.3848684210526434, -1.8092105263158014, -0.493421052631591, -0.24013157894738058, -0.15460526315790668, -1.368421052631591, -3.7072368421052753, -2.2039473684210646, -0.19736842105264363, -0.1907894736842226, -1.6085526315789596, -4.572368421052644, -6.144736842105275, -6.621710526315802, -5.740131578947381, -1.7796052631579067, -3.286184210526328, -0.9967105263158014, 0.6546052631578827, -0.9703947368421174, 0.11842105263156688, -2.750000000000012, -2.825657894736854, -2.54934210526317, -3.4934210526315908, 0.805921052631567, -0.2828947368421173, 1.0197368421052513, 3.2763157894736725, 0.8388157894736723, 0.8223684210526196, -1.0164473684210646, -3.694078947368433, -2.8717105263158014, -5.032894736842117, -5.134868421052643, -4.230263157894749, -3.9078947368421173, -3.1710526315789593, -1.7269736842105383, -2.263157894736854, -1.5361842105263281, -0.875000000000012, -2.4835526315789593, -1.786184210526328, -2.450657894736854, 1.1809210526315668, 2.2269736842105146, 1.9342105263157776, 1.085526315789462, -3.075657894736854, -4.138157894736854, -1.8750000000000118, 0.5953947368420931, 0.9638157894736719, 1.7664473684210398, 0.6151315789473562, -3.11184210526317, -0.5361842105263277, 0.8881578947368303]
  out "Off-Line Smoothed 2":dbl[](array[numeric])=[737.7630026809647, 963.7931635388732, 1122.1765415549585, 1206.0666219839127, 1233.7422252010706, 1227.392359249328, 1198.6537533512046, 1152.8528150134032, 1092.8816353887385, 1022.7844504021434, 942.6061662198382, 853.9419571045571, 761.2046916890079, 667.010321715818, 577.6537533512069, 495.95804289544276, 422.8172922252015, 363.77506702412916, 318.57533512064384, 285.15509383378054, 259.58806970509414, 234.44865951742648, 208.47949061662206, 182.07734584450398, 156.0485254691688, 134.2509383378015, 114.62560321715806, 100.25563002680954, 89.05187667560311, 78.57198391420901, 71.08941018766747, 63.27372654155489, 57.71474530831094, 53.05522788203752, 49.82332439678284, 46.24691689008044, 42.89705093833783, 40.80187667560324, 37.58672922252014, 35.40040214477215, 31.597453083109947, 28.043163538874015, 24.653083109919596, 21.245576407506718, 20.764343163538893, 18.834718498659534, 17.677211796246667, 16.574664879356586, 14.522386058981247, 12.571983914209124, 10.867560321715823, 8.510991957104556, 8.053887399463804, 6.494235924932972, 5.057908847184984, 4.621581769436995, 2.708042895442358, 1.6550938337801595, 0.03579088471849734, -0.9166219839142106, -2.4447721179624677, -1.249061662198393, -1.5084450402144787, -0.722252010723862, 0.13364611260053472, -0.6639410187667575, 0.9111260053619289, 0.47412868632707633, -0.7550938337801623, -0.35630026809651616, -1.0419571045576421, -1.6237265415549613, -1.5560321715817709, -2.6961126005361944, -3.9179624664879373, -3.9333780160857925, -2.7812332439678302, -3.4012064343163564, -4.151206434316356, -3.0024128686327107, -3.879758713136732, -3.9849865951742656, -3.4293565683646143, -4.761796246648796, -4.9856568364611284, -4.0506702412868645, -3.5915549597855243, -3.862332439678286, -3.495710455764076, -4.289946380697053, -3.8884718498659536, -3.5084450402144793, -3.995710455764077, -3.060723860589814, -3.9461126005361944, -3.9628686327077762, -4.309383378016088, -5.083512064343166, -6.360321715817697, -6.3489276139410205, -5.890482573726543, -5.979624664879359, -5.480965147453086, -5.1458445040214515, -4.837533512064346, -5.107640750670244, -4.895844504021451, -5.740348525469171, -6.5252010723860625, -6.5660857908847206, -5.351608579088474, -4.977613941018769, -3.578820375335123, -2.704155495978554, -3.224932975871315, -3.1639410187667574, -4.878418230563005, -5.509785522788206, -5.155898123324399, -5.613002680965151, -4.486327077747992, -4.157238605898126, -4.284584450402147, -3.048659517426275, -3.528552278820377, -3.1525469168900817, -2.9541554959785534, -3.915281501340484, -3.9789544235924943, -3.363002680965149, -2.6197050938337814, -2.987667560321718, -2.9621983914209133, -3.9809651474530856, -4.5017426273458465, -3.759785522788205, -3.273860589812334, -3.7081769436997334, -4.5788203753351215, -5.0707774798927625, -5.055361930294907, -4.609651474530833, -5.275201072386061, -5.353619302949064, -5.5781501340482595, -5.442091152815016, -5.0258713136729245, -4.176005361930296, -5.086863270777483, -5.552010723860593, -4.704825737265418, -5.3080428954423615, -4.27922252010724, -4.06407506702413, -3.9615281501340496, -4.633109919571048, -4.137131367292227, -4.293967828418233, -5.401206434316356, -3.4487935656836486, -2.9568364611260076, -3.0707774798927634, -3.107640750670244, -4.858310991957108, -6.390482573726544, -6.595576407506705, -5.007774798927616, -4.3160857908847206, -4.155898123324399, -3.3824396782841837, -4.1592493297587145, -3.236997319034854, -3.35093833780161, -2.6418230563002694, -2.6880697050938354, -4.415281501340485, -4.03525469168901, -3.8630026809651494, -3.066756032171584, -1.9762734584450417, -1.3764075067024144, -2.580831099195712, -2.148525469168902, -2.125067024128688, -3.66662198391421, -2.63378016085791, -3.867024128686328, -3.8241286863270787, -2.381099195710457, -2.7671581769437013, -2.1364611260053636, -1.7121983914209131, -2.5815013404825753, -1.9534852546916905, -2.427345844504023, -3.374396782841824, -2.1404825737265427, -2.614343163538875, -2.7510723860589827, -1.9957104557640766, -2.8348525469168915, -3.086193029490618, -2.464879356568366, -3.331501340482575, -2.5037533512064356, -2.4367292225201083, -2.3697050938337814, -1.2356568364611276, -1.8442359249329772, -1.516487935656838, -1.8301608579088486, -2.340884718498661, -1.7832439678284198, -1.3663538873994652, -1.413270777479894, -1.3495978552278833, -0.724932975871315, -1.2135388739946393, -1.8697050938337823, -1.2865951742627366, -2.3408847184986614, -2.589544235924935, -0.5902144772117978, -0.5406166219839159, 0.47077747989275986, 0.8789544235924918, -1.1022788203753364, -2.1103217158176957, -2.945442359249331, -2.9615281501340496, -1.9494638069705108, -1.523860589812334, -1.1538873994638084, -1.8254691689008056, -1.863002680965149, -2.604289544235926, -3.2845844504021464, -1.951474530831101, -1.5687667560321734, -0.23297587131367445, 0.7053619302949047, -1.0821715817694384, -0.021849865951743874, -0.2725201072386072, -0.5164879356568378, 0.38163538873994496, -0.9380697050938351, -1.338203753351208, -1.2195710455764088, -0.6994638069705108, -0.7021447721179639, 0.010321715817692895, 0.8407506702412854, 0.08136729222519956, -0.8355227882037548, -1.1029490616621997, -1.447453083109921, -0.4936997319034867, -0.023860589812333965, -0.23900804289544386, -1.2403485254691704, -0.6793565683646127, -0.3482573726541569, -0.3516085790884733, -0.29128686327077896, -1.0453083109919585, -0.4635388739946396, -0.04329758713136875, 0.6349865951742613, -0.34557640750670393, -1.0138069705093848, -1.3924932975871327, -1.3382037533512081, 0.3481233243967814, 0.8126005361930281]
  out "Off-Line Bin Readings 2":dbl[](array[numeric])=[1969.0, 2319.0, 2518.0, 2753.0, 2942.0, 2872.0, 2949.0, 2974.0, 2943.0, 2809.0, 2683.0, 2768.0, 2456.0, 2488.0, 2267.0, 2189.0, 2146.0, 1969.0, 1936.0, 1930.0, 1980.0, 1862.0, 1919.0, 1929.0, 1865.0, 1801.0, 1830.0, 1821.0, 1733.0, 1701.0, 1729.0, 1708.0, 1695.0, 1719.0, 1649.0, 1665.0, 1696.0, 1673.0, 1667.0, 1691.0, 1683.0, 1683.0, 1634.0, 1697.0, 1675.0, 1646.0, 1673.0, 1700.0, 1665.0, 1679.0, 1684.0, 1604.0, 1658.0, 1618.0, 1591.0, 1666.0, 1665.0, 1713.0, 1670.0, 1642.0, 1631.0, 1638.0, 1588.0, 1628.0, 1619.0, 1683.0, 1714.0, 1579.0, 1585.0, 1581.0, 1642.0, 1649.0, 1663.0, 1671.0, 1686.0, 1587.0, 1652.0, 1645.0, 1573.0, 1652.0, 1625.0, 1637.0, 1605.0, 1605.0, 1582.0, 1596.0, 1643.0, 1600.0, 1615.0, 1686.0, 1600.0, 1604.0, 1654.0, 1567.0, 1683.0, 1607.0, 1603.0, 1674.0, 1635.0, 1607.0, 1675.0, 1597.0, 1666.0, 1618.0, 1655.0, 1563.0, 1651.0, 1555.0, 1634.0, 1654.0, 1685.0, 1631.0, 1540.0, 1588.0, 1629.0, 1596.0, 1565.0, 1596.0, 1642.0, 1611.0, 1610.0, 1625.0, 1601.0, 1634.0, 1626.0, 1618.0, 1615.0, 1618.0, 1651.0, 1601.0, 1679.0, 1601.0, 1628.0, 1601.0, 1640.0, 1630.0, 1592.0, 1583.0, 1551.0, 1644.0, 1667.0, 1575.0, 1597.0, 1657.0, 1613.0, 1611.0, 1708.0, 1590.0, 1609.0, 1636.0, 1630.0, 1621.0, 1631.0, 1588.0, 1658.0, 1654.0, 1641.0, 1564.0, 1643.0, 1642.0, 1500.0, 1656.0, 1670.0, 1585.0, 1655.0, 1644.0, 1621.0, 1629.0, 1539.0, 1498.0, 1695.0, 1570.0, 1670.0, 1611.0, 1646.0, 1641.0, 1630.0, 1616.0, 1706.0, 1660.0, 1633.0, 1634.0, 1586.0, 1658.0, 1597.0, 1512.0, 1698.0, 1572.0, 1623.0, 1632.0, 1583.0, 1651.0, 1695.0, 1615.0, 1604.0, 1615.0, 1590.0, 1631.0, 1604.0, 1660.0, 1661.0, 1657.0, 1652.0, 1654.0, 1589.0, 1591.0, 1664.0, 1541.0, 1611.0, 1618.0, 1620.0, 1603.0, 1606.0, 1634.0, 1597.0, 1615.0, 1604.0, 1613.0, 1628.0, 1692.0, 1578.0, 1706.0, 1623.0, 1672.0, 1605.0, 1681.0, 1594.0, 1558.0, 1701.0, 1669.0, 1677.0, 1635.0, 1583.0, 1636.0, 1629.0, 1659.0, 1635.0, 1640.0, 1588.0, 1609.0, 1620.0, 1641.0, 1611.0, 1623.0, 1637.0, 1646.0, 1621.0, 1577.0, 1581.0, 1623.0, 1629.0, 1645.0, 1599.0, 1660.0, 1605.0, 1600.0, 1621.0, 1649.0, 1613.0, 1640.0, 1619.0, 1599.0, 1642.0, 1595.0, 1608.0, 1673.0, 1593.0, 1601.0, 1608.0, 1593.0, 1635.0, 1606.0, 1627.0, 1666.0, 1653.0, 1635.0, 1629.0, 1600.0, 1743.0]
  out "On-Line Smoothed 2":dbl[](array[numeric])=[512.1839142091153, 638.7643431635389, 707.9513404825736, 719.0880697050939, 692.9486595174262, 649.234852546917, 596.6537533512067, 541.2053619302951, 483.76702412868633, 427.3333780160858, 371.05656836461117, 317.15442359249323, 266.9768096514745, 220.0719839142091, 179.66045576407504, 146.09477211796246, 116.9969168900804, 94.93659517426273, 78.5961126005362, 65.53310991957105, 56.1416890080429, 47.11152815013405, 39.43793565683646, 31.704691689008037, 25.579356568364595, 20.878284182305617, 15.040482573726528, 12.100134048257367, 8.232171581769435, 5.809919571045576, 3.6731903485254693, 1.8441018766756028, 0.9513404825737262, -0.5560321715817697, -0.460187667560322, -1.979624664879357, -1.4816353887399467, -2.0453083109919574, -3.3422252010723863, -2.797319034852547, -4.177345844504021, -5.062734584450402, -5.131099195710455, -6.079490616621983, -4.982975871313672, -4.740348525469168, -5.6646112600536185, -5.253753351206434, -6.596246648793565, -7.3053619302949055, -6.565415549597856, -8.006434316353888, -8.55, -9.194101876675603, -9.613672922252011, -8.532573726541553, -7.395844504021447, -6.61970509383378, -7.419973190348525, -8.205495978552278, -8.836193029490616, -9.137131367292225, -9.00710455764075, -8.499731903485253, -8.121715817694371, -8.673994638069704, -7.850268096514746, -7.395174262734585, -8.284584450402145, -6.3697050938337805, -6.635790884718498, -8.204825737265415, -7.834852546916889, -9.23699731903485, -9.070777479892762, -8.547319034852546, -9.115013404825737, -7.740348525469169, -8.001072386058981, -7.570107238605898, -6.9782841823056305, -7.48833780160858, -6.574128686327079, -6.291286863270779, -6.149195710455764, -6.564745308310991, -7.451474530831098, -8.474932975871312, -8.533243967828417, -8.133780160857908, -7.099597855227882, -6.221581769436996, -4.796648793565682, -4.351608579088472, -4.795308310991957, -4.9146112600536185, -6.070107238605898, -6.384450402144772, -6.614343163538874, -5.5875335120643435, -6.395844504021448, -6.490348525469169, -4.972922252010724, -6.332171581769437, -5.304691689008043, -4.898525469168901, -5.830160857908848, -5.006434316353888, -5.434718498659517, -5.889142091152815, -4.484316353887399, -4.444101876675603, -3.8924932975871314, -3.588203753351207, -4.637131367292225, -4.913270777479893, -5.253753351206434, -5.454825737265415, -5.957506702412868, -5.655227882037533, -4.604289544235924, -4.30201072386059, -4.879758713136729, -4.374396782841822, -4.753753351206434, -3.9963806970509372, -2.997721179624665, -3.3636729222520114, -3.5680965147453088, -4.255764075067025, -3.8174262734584454, -3.569436997319035, -2.7865951742627346, -2.705495978552279, -2.995040214477212, -3.4306970509383383, -3.7886058981233246, -3.8904825737265423, -3.4816353887399463, -3.5111260053619304, -3.7798927613941022, -4.252412868632707, -3.907908847184986, -3.751742627345844, -3.411260053619302, -2.700134048257373, -3.3743967828418233, -2.754423592493298, -2.383109919571046, -2.442761394101877, -2.872386058981234, -3.4816353887399467, -3.885790884718499, -3.940750670241287, -3.972922252010724, -3.8033512064343165, -4.316085790884719, -4.010455764075067, -3.7510723860589814, -3.081501340482574, -2.7557640750670243, -2.458176943699732, -2.225603217158177, -2.5486595174262736, -3.052680965147453, -3.1867292225201074, -3.7571045576407505, -3.523860589812332, -2.1793565683646112, -2.289946380697051, -1.0278820375335123, -1.6270777479892764, -2.0975871313672925, -1.9193029490616624, -3.125067024128687, -2.9983914209115285, -2.9528150134048263, -3.5774798927613944, -3.497050938337802, -3.1679624664879356, -3.965549597855228, -2.9983914209115285, -2.7323056300268096, -2.6009383378016087, -1.9675603217158177, -2.745040214477212, -2.6351206434316357, -3.557372654155496, -4.130428954423593, -3.587533512064343, -2.986997319034853, -2.9018766756032175, -1.6793565683646114, -1.5895442359249334, -1.6190348525469174, -0.8971849865951745, -2.3194369973190354, -3.0942359249329763, -3.7483914209115285, -3.721581769436998, -3.3583109919571044, -3.1632707774798927, -3.5017426273458443, -3.442761394101876, -2.477613941018767, -1.98029490616622, -0.7906166219839145, -0.34289544235924957, -0.6310991957104561, -0.2939678284182308, -0.6056300268096517, -1.5540214477211798, -1.6612600536193034, -2.0721179624664883, -1.7162198391420913, -1.0399463806970513, -1.311394101876676, -1.2517426273458447, -1.8609919571045581, -1.403217158176944, -1.6203753351206438, -2.2517426273458447, -2.649865951742628, -3.581501340482574, -3.3449061662198396, -2.395844504021448, -1.727613941018767, -0.5734584450402146, -0.6773458445040217, -1.9199731903485255, -1.529892761394102, -2.19544235924933, -1.4146112600536194, -0.5680965147453085, -1.277211796246649, -1.4320375335120645, -1.8247989276139414, -1.5533512064343167, -1.3227882037533516, -0.5975871313672925, -0.413270777479893, -0.3395442359249332, -0.7993297587131369, -1.8971849865951746, -1.8368632707774804, -1.5225201072386063, -0.9293565683646117, 0.0009383378016083188, -0.004423592493297837, 0.021715817694369755, 0.36420911528150113, 0.7965147453083107, 1.3092493297587129, 1.9057640750670237, 2.500268096514745, 2.047855227882037, 0.39034852546916876, -0.2557640750670242, -1.363672922252011, -1.6411528150134052, -0.12372654155495993, -1.0567024128686329, 0.19329758713136713, 0.29249329758713116, 0.7542895442359248, 1.8621983914209115, 1.1463806970509383, 0.006970509383377843, -0.21152815013404852, -1.247721179624665, -0.9045576407506705, 0.297184986595174, -0.2021447721179627, 0.7435656836461124, 0.9339142091152812]
  out "On-Line Bin Readings 2":dbl[](array[numeric])=[1931.0, 2137.0, 2311.0, 2341.0, 2387.0, 2422.0, 2291.0, 2251.0, 2344.0, 2214.0, 2108.0, 2141.0, 1988.0, 1865.0, 1768.0, 1801.0, 1774.0, 1692.0, 1696.0, 1688.0, 1700.0, 1641.0, 1704.0, 1653.0, 1613.0, 1617.0, 1684.0, 1673.0, 1747.0, 1639.0, 1589.0, 1559.0, 1662.0, 1572.0, 1558.0, 1613.0, 1653.0, 1588.0, 1591.0, 1584.0, 1598.0, 1581.0, 1602.0, 1575.0, 1571.0, 1567.0, 1609.0, 1644.0, 1575.0, 1623.0, 1620.0, 1623.0, 1646.0, 1653.0, 1675.0, 1612.0, 1563.0, 1612.0, 1616.0, 1621.0, 1594.0, 1635.0, 1647.0, 1631.0, 1660.0, 1558.0, 1621.0, 1579.0, 1622.0, 1526.0, 1638.0, 1650.0, 1593.0, 1599.0, 1620.0, 1659.0, 1636.0, 1576.0, 1575.0, 1688.0, 1599.0, 1599.0, 1594.0, 1540.0, 1608.0, 1537.0, 1595.0, 1561.0, 1565.0, 1617.0, 1590.0, 1671.0, 1644.0, 1604.0, 1573.0, 1557.0, 1623.0, 1647.0, 1513.0, 1604.0, 1606.0, 1627.0, 1624.0, 1512.0, 1652.0, 1646.0, 1640.0, 1639.0, 1624.0, 1585.0, 1601.0, 1555.0, 1601.0, 1613.0, 1601.0, 1644.0, 1672.0, 1552.0, 1628.0, 1604.0, 1620.0, 1620.0, 1592.0, 1618.0, 1615.0, 1652.0, 1617.0, 1607.0, 1619.0, 1543.0, 1700.0, 1544.0, 1561.0, 1591.0, 1592.0, 1655.0, 1590.0, 1610.0, 1618.0, 1611.0, 1621.0, 1555.0, 1583.0, 1564.0, 1515.0, 1688.0, 1607.0, 1622.0, 1573.0, 1594.0, 1597.0, 1683.0, 1623.0, 1607.0, 1544.0, 1641.0, 1622.0, 1634.0, 1677.0, 1599.0, 1635.0, 1600.0, 1585.0, 1604.0, 1635.0, 1677.0, 1633.0, 1683.0, 1620.0, 1629.0, 1563.0, 1540.0, 1611.0, 1612.0, 1604.0, 1595.0, 1661.0, 1564.0, 1608.0, 1616.0, 1571.0, 1557.0, 1593.0, 1592.0, 1618.0, 1565.0, 1580.0, 1570.0, 1614.0, 1646.0, 1561.0, 1634.0, 1586.0, 1588.0, 1639.0, 1576.0, 1629.0, 1600.0, 1589.0, 1519.0, 1586.0, 1617.0, 1607.0, 1607.0, 1553.0, 1545.0, 1571.0, 1642.0, 1605.0, 1607.0, 1573.0, 1583.0, 1591.0, 1612.0, 1599.0, 1594.0, 1541.0, 1670.0, 1611.0, 1590.0, 1592.0, 1586.0, 1606.0, 1614.0, 1604.0, 1540.0, 1586.0, 1632.0, 1539.0, 1617.0, 1659.0, 1640.0, 1624.0, 1712.0, 1599.0, 1611.0, 1677.0, 1573.0, 1631.0, 1593.0, 1615.0, 1647.0, 1632.0, 1627.0, 1595.0, 1575.0, 1520.0, 1633.0, 1583.0, 1590.0, 1689.0, 1630.0, 1637.0, 1660.0, 1578.0, 1618.0, 1605.0, 1612.0, 1653.0, 1662.0, 1519.0, 1539.0, 1537.0, 1588.0, 1647.0, 1653.0, 1674.0, 1654.0, 1685.0, 1604.0, 1615.0, 1628.0, 1617.0, 1618.0, 1631.0, 1615.0, 1526.0, 1576.0, 1669.0]
  in  "stop":bool
  in  "Reset Average":bool=TRUE
  in  "Save Data?":bool=TRUE
  in  "Collect Data?":bool=TRUE
  in  "Tab Control":T2(tab)=enum."g/m^3"
  out "Water Vapor Number Density  2":cluster{"Y":dbl[], "Y":dbl[]}[](graph)
  out "Absolute Humidity":cluster{"Y":dbl[], "Y":dbl[]}[](graph)
  out "NRB plot":cluster{"Y":dbl[], "Y":dbl[]}[](graph)
  in  "background length":i32=10
  out "Correction":cluster{"Y":dbl[], "Y":dbl[]}[](graph)
  in  "dead time":dbl=3.7e-08
  out "Optical Depth":cluster{"Y":dbl[], "Y":dbl[]}[](graph) caption="XY Graph"
  out "RingBuffer offline far":dbl[][](array[numeric])
  out "RingBuffer aerosol far":dbl[][](array[numeric])
  in  "Weather":T3(tab)=enum."Pulse Energy (Micro Joule)"
  out "Temperature (C)":dbl(graph)=28.233974358974365
  out "Pressure (mb)":dbl(graph)=842.3763736263736
  out "Relative Humdity (%)":dbl(graph)=31.846764346764346
  out "Pulse Energy (Micro Joule)":cluster{dbl}(graph)={3.7142857142857144}
  in  "PRF (kHz)":dbl=7.0
  out "?":cluster{"mean":dbl, "mean":dbl}(graph)={"mean"=55220.00000000001, "mean"=327740.0}
  out "Index":i32=56
  out "Aerosol Smoothed":dbl[](array[numeric])=[140.37105263157895, 191.4861842105263, 254.97631578947363, 324.2296052631578, 399.0355263157894, 471.4072368421052, 536.8184210526315, 595.5519736842105, 642.5947368421052, 672.1177631578948, 683.2855263157895, 678.0125, 653.8052631578947, 617.920394736842, 572.6934210526315, 522.6572368421052, 477.88421052631577, 444.8611842105263, 424.47960526315785, 409.94342105263155, 396.20328947368415, 376.89078947368415, 351.45986842105253, 322.4039473684209, 292.1177631578946, 262.9105263157894, 237.34144736842103, 215.62763157894736, 196.0618421052631, 181.57171052631577, 167.3019736842105, 157.0782894736842, 148.4138157894737, 139.1276315789474, 133.1901315789474, 124.90723684210528, 119.27894736842109, 112.12434210526318, 105.92697368421055, 100.81184210526318, 95.87763157894739, 91.47960526315794, 85.35131578947372, 81.29210526315792, 75.58486842105266, 70.43026315789476, 67.83486842105265, 63.476315789473695, 59.805263157894736, 57.37434210526315, 53.44671052631579, 49.54210526315789, 46.4828947368421, 44.18684210526315, 42.121052631578934, 39.81842105263157, 37.555263157894736, 33.86118421052632, 30.292105263157893, 28.07171052631579, 27.26907894736842, 27.042105263157893, 26.02236842105263, 26.430263157894732, 24.759210526315783, 24.788815789473684, 25.459868421052633, 24.851315789473684, 24.39736842105263, 22.854605263157893, 21.206578947368417, 18.558552631578948, 16.167105263157897, 14.49934210526316, 13.1046052631579, 12.7921052631579, 12.413815789473688, 11.959868421052636, 11.499342105263162, 11.084868421052636, 10.72631578947369, 9.844736842105268, 9.032236842105268, 8.384210526315796, 8.084868421052636, 8.532236842105268, 9.565131578947373, 10.36447368421053, 10.157236842105267, 10.871052631578952, 10.532236842105268, 10.002631578947373, 9.900657894736847, 7.778947368421055, 7.423684210526318, 5.884210526315792, 5.101315789473687, 5.973026315789477, 5.7657894736842135, 7.341447368421056, 7.565131578947372, 6.834868421052634, 6.571710526315791, 5.114473684210528, 5.426973684210528, 4.670394736842107, 4.63092105263158, 4.887500000000001, 4.890789473684212, 4.930263157894738, 4.081578947368422, 4.851315789473686, 5.716447368421056, 6.193421052631582, 6.232894736842107, 5.0717105263157904, 4.124342105263159, 3.3513157894736856, 3.9401315789473697, 3.9006578947368435, 3.5289473684210533, 4.828289473684211, 4.456578947368422, 4.6342105263157904, 4.726315789473686, 3.8118421052631595, 4.1605263157894745, 4.278947368421054, 4.078289473684212, 3.7000000000000015, 3.0059210526315803, 2.101315789473685, 1.5914473684210542, 3.515789473684213, 3.5190789473684236, 3.9072368421052657, 4.213157894736844, 2.7953947368421064, 3.2690789473684223, 3.555263157894738, 3.621052631578949, 3.0322368421052643, 2.545394736842107, 2.647368421052633, 3.772368421052634, 4.134210526315792, 5.071710526315791, 4.446710526315791, 2.8381578947368435, 2.6013157894736856, 1.3447368421052643, 1.0026315789473697, 0.5322368421052643, -0.46776315789473555, -0.6026315789473671, -0.4118421052631566, -0.13223684210526185, 1.0125000000000013, 0.9763157894736856, 0.8611842105263171, 1.1309210526315803, 1.4697368421052643, 2.084868421052633, 2.7888157894736856, 2.37763157894737, 2.5421052631578958, 2.061842105263159, 1.9434210526315803, 2.5256578947368435, 2.473026315789475, 3.1506578947368435, 3.06513157894737, 2.62763157894737, 2.5750000000000015, 1.6868421052631595, 1.3250000000000015, 1.7953947368421068, 1.2197368421052643, 2.3743421052631595, 3.1440789473684223, 2.785526315789475, 2.8940789473684223, 2.1901315789473697, 1.2427631578947382, 1.575000000000001, 1.1901315789473697, 0.979605263157896, 0.9269736842105275, 1.1703947368421066, 1.5881578947368433, 1.0684210526315803, 1.8710526315789489, 0.9368421052631591, 0.2000000000000013, 0.4467105263157908, -0.06973684210526182, 0.31184210526315925, 1.5750000000000015, 2.81513157894737, 3.104605263157896, 2.982894736842107, 2.104605263157896, 0.8151315789473698, 2.0125000000000015, 2.542105263157896, 3.0026315789473697, 2.4828947368421064, 1.3644736842105276, 1.0552631578947382, 0.25263157894736976, 1.2000000000000013, 0.33815789473684343, -0.12236842105263024, 0.0059210526315803, -1.3098684210526301, 0.028947368421054054, 0.3546052631578962, 0.7164473684210542, 1.5881578947368433, 0.7427631578947382, -0.28355263157894606, -0.1749999999999987, -0.020394736842103994, -0.1388157894736829, 0.466447368421054, -0.1453947368421039, 0.11776315789473824, 0.5157894736842119, 1.1243421052631593, 1.673684210526317, 1.1046052631578962, 1.2493421052631595, 1.4763157894736856, 1.6736842105263172, 1.7460526315789489, 0.9631578947368432, 0.9993421052631591, 0.46644736842105394, 0.8513157894736856, 1.8447368421052643, 1.1769736842105276, 1.078289473684212, 1.0026315789473697, -0.28026315789473544, -0.3986842105263144, -0.5697368421052618, -0.7046052631578934, 0.3776315789473697, 1.153947368421054, 0.8809210526315803, 0.8677631578947382, 0.9138157894736856, 0.8052631578947382, 0.9203947368421068, 0.5684210526315805, 0.4828947368421066, -0.7177631578947355, -0.03026315789473555, 1.124342105263159, -0.19473684210526188, -0.576315789473683, -0.7934210526315777, -1.388815789473683, 0.3282894736842118, 1.117763157894738, 1.522368421052633, 1.9269736842105276, 0.6144736842105276, 0.5914473684210539, 0.45000000000000134, -0.2473684210526302, 0.3184210526315803, 0.8578947368421066, 0.8348684210526329, 0.23947368421052762]
  out "Off-Line  Bin Readings":dbl[](array[numeric])=[341.0, 404.0, 426.0, 502.0, 576.0, 641.0, 644.0, 788.0, 865.0, 933.0, 1039.0, 994.0, 1034.0, 999.0, 968.0, 878.0, 835.0, 692.0, 718.0, 720.0, 649.0, 720.0, 700.0, 683.0, 616.0, 568.0, 559.0, 537.0, 502.0, 487.0, 446.0, 394.0, 415.0, 435.0, 442.0, 417.0, 409.0, 396.0, 361.0, 382.0, 380.0, 373.0, 373.0, 367.0, 396.0, 345.0, 375.0, 335.0, 318.0, 336.0, 311.0, 332.0, 305.0, 341.0, 295.0, 339.0, 321.0, 329.0, 335.0, 306.0, 340.0, 279.0, 280.0, 325.0, 320.0, 290.0, 297.0, 282.0, 311.0, 296.0, 267.0, 286.0, 307.0, 294.0, 274.0, 306.0, 281.0, 311.0, 288.0, 275.0, 269.0, 271.0, 265.0, 279.0, 283.0, 273.0, 296.0, 290.0, 290.0, 289.0, 289.0, 301.0, 315.0, 250.0, 277.0, 296.0, 315.0, 288.0, 285.0, 313.0, 288.0, 264.0, 261.0, 273.0, 268.0, 269.0, 291.0, 278.0, 267.0, 255.0, 270.0, 289.0, 282.0, 267.0, 311.0, 293.0, 269.0, 307.0, 285.0, 301.0, 310.0, 292.0, 280.0, 313.0, 258.0, 281.0, 264.0, 291.0, 288.0, 266.0, 249.0, 283.0, 280.0, 280.0, 288.0, 279.0, 309.0, 264.0, 283.0, 291.0, 265.0, 301.0, 281.0, 238.0, 311.0, 255.0, 275.0, 263.0, 264.0, 282.0, 303.0, 268.0, 276.0, 260.0, 254.0, 289.0, 288.0, 305.0, 263.0, 267.0, 273.0, 244.0, 309.0, 293.0, 277.0, 286.0, 284.0, 305.0, 286.0, 270.0, 292.0, 266.0, 295.0, 300.0, 261.0, 300.0, 253.0, 289.0, 295.0, 273.0, 265.0, 246.0, 251.0, 282.0, 276.0, 253.0, 297.0, 281.0, 296.0, 290.0, 278.0, 291.0, 273.0, 334.0, 290.0, 275.0, 264.0, 268.0, 287.0, 262.0, 252.0, 260.0, 273.0, 283.0, 262.0, 258.0, 270.0, 282.0, 280.0, 277.0, 283.0, 275.0, 270.0, 268.0, 276.0, 286.0, 256.0, 286.0, 281.0, 306.0, 261.0, 279.0, 250.0, 274.0, 283.0, 260.0, 259.0, 261.0, 240.0, 252.0, 259.0, 295.0, 273.0, 254.0, 264.0, 282.0, 256.0, 308.0, 280.0, 276.0, 307.0, 289.0, 256.0, 271.0, 294.0, 275.0, 266.0, 246.0, 281.0, 273.0, 286.0, 289.0, 262.0, 238.0, 284.0, 276.0, 271.0, 252.0, 280.0, 271.0, 265.0, 282.0, 275.0, 268.0, 263.0, 268.0, 263.0, 280.0, 280.0, 306.0, 278.0, 272.0, 254.0, 297.0, 281.0, 264.0, 278.0, 258.0, 273.0]
  out "Off-Line Smoothed":dbl[](array[numeric])=[127.77426273458451, 172.54235924932982, 227.732707774799, 289.64959785522797, 354.35335120643435, 419.08525469168904, 481.18176943699734, 536.7601876675602, 584.6268096514743, 622.284986595174, 642.3573726541553, 646.1261394101875, 633.4719839142089, 605.5014745308309, 570.7166219839141, 527.8305630026808, 482.8037533512064, 443.6603217158178, 411.3821715817695, 388.9833780160859, 371.84061662198405, 352.78632707774807, 328.95455764075075, 301.4290884718499, 273.13619302949064, 245.35000000000008, 220.8955764075068, 200.36407506702426, 182.35938337801622, 168.23538873994647, 155.8654155495979, 146.39222520107242, 138.71461126005363, 131.58860589812335, 126.45857908847185, 120.63887399463806, 115.62278820375334, 110.16166219839138, 104.41836461126002, 99.68780160857908, 94.41367292225199, 89.60603217158175, 84.59463806970507, 79.55509383378015, 74.53565683646111, 69.32922252010722, 65.1563002680965, 60.84731903485254, 56.555093833780134, 52.8037533512064, 48.49410187667557, 44.28029490616619, 40.62680965147452, 37.98806970509382, 35.37949061662198, 33.49745308310992, 31.606032171581766, 29.33525469168901, 27.985388739946384, 26.544369973190353, 25.264879356568372, 24.046380697050946, 22.511528150134055, 20.89959785522789, 19.872117962466497, 19.20254691689009, 18.80978552278821, 18.112734584450408, 17.195844504021455, 16.5745308310992, 16.060455764075073, 15.16836461126006, 14.343967828418238, 13.205898123324408, 12.327882037533525, 12.067828418230576, 11.781635388739957, 11.52225201072387, 10.843967828418236, 10.449195710455768, 10.24879356568365, 9.49477211796247, 8.901608579088471, 8.667024128686327, 8.21729222520107, 8.605361930294906, 8.965951742627349, 8.80241286863271, 8.51152815013405, 8.114075067024126, 7.471313672922248, 7.09664879356568, 7.347989276139406, 6.719302949061658, 6.643565683646109, 5.983378016085788, 5.019571045576405, 4.935120643431633, 5.292359249329756, 5.625469168900802, 5.4967828418230535, 5.356032171581767, 5.181769436997316, 5.091957104557637, 5.212600536193026, 5.139544235924929, 4.67640750670241, 3.9237265415549585, 4.170375335120641, 3.6402144772117944, 3.4532171581769413, 3.834584450402142, 3.620107238605896, 4.108042895442356, 4.064477211796244, 3.78900804289544, 4.092627345844502, 3.7869973190348514, 3.605361930294904, 3.6449061662198377, 2.8841823056300253, 2.8386058981233226, 3.059785522788203, 2.892895442359248, 3.045710455764074, 2.888873994638069, 2.260187667560321, 2.2983914209115275, 2.3305630026809636, 2.5396782841823042, 2.650938337801607, 2.6395442359249324, 2.1234584450402143, 2.3882037533512053, 2.33592493297587, 2.4264075067024122, 2.6428954423592486, 2.106032171581769, 2.376139410187667, 1.9404825737265408, 2.1375335120643424, 1.833243967828417, 1.8426273458445028, 1.9237265415549585, 1.8017426273458437, 2.1402144772117953, 1.8754691689008034, 1.8138069705093827, 1.223324396782841, 1.3097855227882027, 0.9558981233243957, 0.5604557640750658, 0.5946380697050926, -0.05951742627345917, 0.17104557640750595, 0.8654155495978544, 1.0383378016085782, 1.0336461126005354, 0.9371313672922243, 0.5872654155495971, 0.7126005361930288, 1.0497319034852541, 1.284316353887399, 1.4371313672922246, 1.6938337801608572, 1.8419571045576397, 1.6221179624664872, 1.1824396782841813, 0.5832439678284175, 0.46461126005361864, 0.5148793565683639, 0.5450402144772111, 0.6750670241286856, 0.5624664879356561, 0.6308310991957096, 0.5195710455764067, 0.476005361930294, 0.4961126005361922, 0.5088471849865945, 0.9156836461125999, 0.9894101876675596, 0.7092493297587125, 0.4116621983914201, 0.2742627345844496, 0.33056300268096434, 0.517560321715817, 0.631501340482573, 0.3654155495978545, 0.5798927613941012, 0.4760053619302942, 0.3627345844504014, 0.9056300268096507, 0.7856568364611252, 0.6891420911528142, 0.9170241286863263, 0.4840482573726533, 0.20321715817694294, 0.6663538873994631, 0.7119302949061657, 0.601340482573726, 0.7816353887399459, 0.26621983914209046, 0.20790884718498556, 0.6201072386058971, 0.28163538873994537, 0.866756032171581, 0.3855227882037528, -0.01327077747989329, 0.0028150134048251785, -0.5199731903485263, -0.28605898123324464, 0.019571045576406765, -0.18820375335120695, -0.07158176943699784, -0.1506702412868638, -0.0025469168900810746, 0.4572386058981224, 0.3687667560321707, 0.047050938337800774, 0.016219839142090464, -0.2706434316353894, 0.04235924932975804, 0.5879356568364604, 0.5463806970509376, 0.9666219839142084, 0.8392761394101869, 0.5752010723860582, 0.43243967828418156, 0.267560321715817, 0.016219839142090464, 0.17774798927613872, -0.04008042895442428, 0.09597855227881966, 0.1891420911528143, 0.08458445040214407, 0.1616621983914202, 0.1449061662198384, 0.12345844504021372, 0.04034852546916817, 0.09396782841822983, 0.028284182305629305, 0.14691689008042824, 0.024932975871312935, -0.11447721179624736, -0.5146112600536201, -0.5957104557640759, -0.6620643431635396, -0.5400804289544243, -0.2378016085790892, -0.7686327077747996, -0.7538873994638078, -0.9985254691689016, -0.8323056300268104, -0.38726541554959865, -0.13726541554959854, -0.2706434316353894, -0.7036193029490623, -0.3912868632707781, -0.25187667560321775, -0.2699731903485261, -0.3604557640750677, -0.7833780160857915, -1.0058981233243973, -0.13123324396782898, -0.1995978552278826, 0.10536193029490565, 0.3218498659517421, -0.08565683646112665, 0.4344504021447714, 0.37680965147453016, 0.0008042895442351705, -0.15737265415549673, 0.012198391420910781, 0.002144772117961699, -0.13525469168900855]
  out "On-Line  Smoothed":dbl[](array[numeric])=[77.79235924932973, 97.45455764075061, 120.67238605898115, 144.74477211796236, 168.4880697050937, 190.04436997319024, 207.21662198391414, 219.78833780160852, 227.4887399463807, 229.13217158176946, 225.18646112600538, 215.52962466487935, 200.42439678284177, 182.48739946380687, 163.08257372654143, 143.80643431635377, 125.28833780160848, 109.58056300268089, 97.44182305630021, 87.66233243967825, 80.9445040214477, 73.52761394101876, 66.19986595174262, 58.40428954423593, 50.3593833780161, 44.01152815013407, 38.35335120643435, 33.34932975871317, 29.80241286863273, 27.2353887399464, 24.663002680965164, 23.435120643431645, 21.9304289544236, 19.96193029490617, 18.592627345844512, 17.414343163538877, 16.333914209115285, 15.277613941018767, 14.066487935656836, 12.718632707774798, 11.853351206434315, 11.21997319034852, 11.156300268096512, 10.152949061662193, 9.488069705093826, 8.835254691689, 7.795040214477203, 7.6804289544235855, 7.335924932975866, 6.442493297587128, 5.6328418230562995, 4.827882037533514, 3.9190348525469214, 3.714611260053624, 3.5383378016085847, 3.5483914209115333, 3.260857908847189, 2.9994638069705126, 2.5363270777479916, 2.173726541554961, 1.6408847184986606, 1.3902144772117975, 1.2441018766756047, 1.435120643431637, 1.739410187667562, 1.5416890080428967, 1.9491957104557656, 1.1201072386058992, 0.8707774798927623, 0.8184986595174272, 0.3560321715817701, 0.805764075067025, 0.7554959785522796, 0.6489276139410194, 0.7132707774798934, 0.37144772117962527, 0.46662198391420995, 0.7327077747989286, 0.9833780160857921, 1.573860589812334, 1.7615281501340496, 1.556434316353889, 0.7742627345844515, 0.29369973190348614, -0.491152815013404, -0.24919571045576328, 0.12144772117962543, -0.31018766756032107, -0.048793565683645596, -0.3034852546916885, -0.26997319034852496, -0.21903485254691626, 0.12680965147453147, -0.44021447721179535, -0.30951742627345735, 0.4337801608579103, 0.2608579088471865, 0.8184986595174274, 0.28230563002681075, -0.15402144772117898, 0.010857908847185627, 0.03297587131367357, 0.02828418230563065, -0.08498659517426209, -0.307506702412868, -0.7378016085790876, -0.19624664879356468, 0.14691689008043013, 0.032975871313674104, 0.6563002680965156, 0.39289544235925017, 0.07922252010723926, 0.07252010723860655, -0.2619302949061656, -0.12184986595174199, 0.17908847184986657, 0.0684986595174269, 0.02225201072386121, -0.15938337801608515, -0.4107238605898117, 0.012198391420912169, 0.31581769436997387, 0.30241286863270844, 0.5235924932975877, 0.41568364611260117, -0.3302949061662188, -0.48042895442359146, -0.5869973190348515, -0.4971849865951733, 0.16769436997319098, 0.14423592493297654, -0.1171581769436991, -0.22908847184986533, -0.5018766756032165, -0.3262734584450396, 0.07922252010723932, 0.41970509383378113, 0.7943699731903495, 0.7903485254691699, 0.7260053619302957, 0.1790884718498666, -0.08833780160857843, -0.46367292225200984, -0.9563002680965139, -1.0782841823056293, -1.2927613941018754, -0.9844504021447713, -0.5172922252010714, -0.39128686327077644, -0.14396782841822992, 0.051072386058981886, -0.29946380697050873, 0.02091152815013468, 0.005495978552279457, 0.15361930294906234, 0.5926273458445047, 0.29571045576407573, 0.045710455764075675, -0.39329758713136664, -0.8584450402144767, -0.6426273458445035, -0.3684986595174257, -0.10375335120643375, -0.17546916890080366, -0.14597855227881973, 0.14356568364611333, -0.224396782841822, -0.006568364611259009, -0.4274798927613928, -0.6922252010723848, -0.7847184986595163, -0.6097855227882026, -0.8101876675603206, -0.9288203753351195, -0.5575067024128678, -1.0749329758713126, -0.6707774798927605, -0.2639410187667551, -0.09906166219839055, 0.0644772117962473, 0.07587131367292292, 0.19986595174262806, -0.1392761394101869, -0.15067024128686252, -0.11447721179624588, -0.3504021447721173, 0.07050938337801677, 0.1569705093833787, 0.32319034852546985, -0.09571045576407416, -0.19155495978552195, -0.16943699731903403, -0.28270777479892684, 0.13351206434316412, 0.20053619302949124, 0.24008042895442422, -0.04879356568364546, -0.24182305630026743, -0.453619302949061, -0.5300268096514739, -0.3939678284182299, -0.3597855227882031, -0.5809651474530825, -0.550134048257372, 0.11005361930294999, -0.10509383378015993, -0.018632707774797988, 0.15428954423592586, -0.6064343163538868, -0.08565683646112526, 0.05643431635388815, -0.11447721179624593, 0.12345844504021518, -0.14530831099195649, -0.07493297587131302, 0.06112600536193094, -0.0481233243967822, -0.050804289544235284, 0.15093833780160942, -0.17546916890080344, -0.129892761394101, -0.1553619302949053, -0.2833780160857902, 0.1697050938337808, -0.01461126005361868, -0.0005361930294899477, 0.020911528150134667, -0.4623324396782835, -0.5843163538873988, -1.0126005361930284, -1.2431635388739934, -1.0916890080428943, -0.6352546916890071, -0.45361930294906105, -0.7130026809651469, -0.696246648793565, -1.0534852546916884, -0.6540214477211789, -0.88793565683646, -0.5970509383378005, -0.5045576407506692, -0.788739946380696, -0.04477211796246586, -0.11045576407506635, 0.48471849865951805, 0.2970509383378022, 0.5819034852546924, 0.5664879356568372, 0.2675603217158184, 0.2508042895442369, -0.6077747989276127, -0.5735924932975858, -1.1546916890080414, -0.6841823056300256, -0.05080428954423516, -0.3457104557640743, -0.23780160857908755, -0.49651474530830997, -0.7699731903485245, -0.5595174262734575, -0.5126005361930288, -0.4207774798927608, -0.17680965147453026, -0.3289544235924927, 0.047050938337802245, 0.31514745308311054, 0.2367292225201079, 0.34329758713136793, 0.29571045576407573, 0.18310991957104622, -0.11447721179624572, -0.02801608579088378, 0.37278820375335214, -0.13190348525469048, -0.017292225201071484]
  out "On-Line Bin Readings":dbl[](array[numeric])=[316.0, 329.0, 379.0, 368.0, 414.0, 467.0, 469.0, 506.0, 517.0, 525.0, 536.0, 508.0, 542.0, 509.0, 472.0, 451.0, 396.0, 374.0, 370.0, 366.0, 357.0, 353.0, 343.0, 344.0, 338.0, 328.0, 323.0, 310.0, 327.0, 329.0, 320.0, 260.0, 295.0, 277.0, 297.0, 291.0, 295.0, 289.0, 302.0, 308.0, 266.0, 308.0, 285.0, 289.0, 294.0, 286.0, 295.0, 280.0, 280.0, 270.0, 277.0, 272.0, 274.0, 261.0, 250.0, 254.0, 250.0, 289.0, 269.0, 286.0, 278.0, 274.0, 302.0, 250.0, 253.0, 276.0, 252.0, 306.0, 292.0, 250.0, 240.0, 258.0, 238.0, 255.0, 271.0, 286.0, 251.0, 257.0, 273.0, 255.0, 271.0, 280.0, 286.0, 264.0, 297.0, 283.0, 311.0, 281.0, 262.0, 276.0, 301.0, 262.0, 280.0, 267.0, 258.0, 281.0, 297.0, 291.0, 256.0, 279.0, 275.0, 263.0, 232.0, 292.0, 308.0, 264.0, 294.0, 286.0, 255.0, 275.0, 276.0, 254.0, 280.0, 253.0, 263.0, 294.0, 293.0, 264.0, 265.0, 228.0, 265.0, 267.0, 268.0, 308.0, 243.0, 267.0, 264.0, 296.0, 276.0, 262.0, 278.0, 286.0, 255.0, 317.0, 272.0, 268.0, 273.0, 249.0, 295.0, 273.0, 253.0, 266.0, 265.0, 260.0, 272.0, 276.0, 292.0, 260.0, 265.0, 279.0, 264.0, 283.0, 252.0, 262.0, 274.0, 268.0, 270.0, 291.0, 269.0, 259.0, 246.0, 276.0, 261.0, 257.0, 266.0, 282.0, 270.0, 248.0, 248.0, 273.0, 274.0, 255.0, 311.0, 264.0, 285.0, 266.0, 295.0, 240.0, 284.0, 263.0, 275.0, 259.0, 267.0, 269.0, 278.0, 281.0, 256.0, 302.0, 286.0, 254.0, 293.0, 266.0, 279.0, 285.0, 282.0, 260.0, 267.0, 252.0, 282.0, 274.0, 273.0, 258.0, 255.0, 275.0, 283.0, 281.0, 283.0, 285.0, 258.0, 235.0, 279.0, 297.0, 268.0, 296.0, 237.0, 278.0, 288.0, 253.0, 239.0, 233.0, 302.0, 286.0, 241.0, 244.0, 251.0, 261.0, 254.0, 272.0, 281.0, 269.0, 277.0, 258.0, 278.0, 260.0, 285.0, 276.0, 284.0, 261.0, 275.0, 262.0, 273.0, 258.0, 257.0, 275.0, 267.0, 249.0, 275.0, 260.0, 282.0, 261.0, 278.0, 282.0, 252.0, 281.0, 267.0, 279.0, 287.0, 281.0, 277.0, 267.0, 259.0, 274.0, 242.0, 279.0, 289.0, 266.0, 283.0, 259.0, 270.0, 245.0, 302.0, 291.0, 258.0, 284.0, 292.0, 287.0, 275.0, 249.0, 280.0]
  out "Range Corrected Altitude Array":dbl[](array[numeric])=[5625.0, 22500.0, 50625.0, 90000.0, 140625.0, 202500.0, 275625.0, 360000.0, 455625.0, 562500.0, 680625.0, 810000.0, 950625.0, 1102500.0, 1265625.0, 1440000.0, 1625625.0, 1822500.0, 2030625.0, 2250000.0, 2480625.0, 2722500.0, 2975625.0, 3240000.0, 3515625.0, 3802500.0, 4100625.0, 4410000.0, 4730625.0, 5062500.0, 5405625.0, 5760000.0, 6125625.0, 6502500.0, 6890625.0, 7290000.0, 7700625.0, 8122500.0, 8555625.0, 9000000.0, 9455625.0, 9922500.0, 10400625.0, 10890000.0, 11390625.0, 11902500.0, 12425625.0, 12960000.0, 13505625.0, 14062500.0, 14630625.0, 15210000.0, 15800625.0, 16402500.0, 17015625.0, 17640000.0, 18275625.0, 18922500.0, 19580625.0, 20250000.0, 20930625.0, 21622500.0, 22325625.0, 23040000.0, 23765625.0, 24502500.0, 25250625.0, 26010000.0, 26780625.0, 27562500.0, 28355625.0, 29160000.0, 29975625.0, 30802500.0, 31640625.0, 32490000.0, 33350625.0, 34222500.0, 35105625.0, 36000000.0, 36905625.0, 37822500.0, 38750625.0, 39690000.0, 40640625.0, 41602500.0, 42575625.0, 43560000.0, 44555625.0, 45562500.0, 46580625.0, 47610000.0, 48650625.0, 49702500.0, 50765625.0, 51840000.0, 52925625.0, 54022500.0, 55130625.0, 56250000.0, 57380625.0, 58522500.0, 59675625.0, 60840000.0, 62015625.0, 63202500.0, 64400625.0, 65610000.0, 66830625.0, 68062500.0, 69305625.0, 70560000.0, 71825625.0, 73102500.0, 74390625.0, 75690000.0, 77000625.0, 78322500.0, 79655625.0, 81000000.0, 82355625.0, 83722500.0, 85100625.0, 86490000.0, 87890625.0, 89302500.0, 90725625.0, 92160000.0, 93605625.0, 95062500.0, 96530625.0, 98010000.0, 99500625.0, 101002500.0, 102515625.0, 104040000.0, 105575625.0, 107122500.0, 108680625.0, 110250000.0, 111830625.0, 113422500.0, 115025625.0, 116640000.0, 118265625.0, 119902500.0, 121550625.0, 123210000.0, 124880625.0, 126562500.0, 128255625.0, 129960000.0, 131675625.0, 133402500.0, 135140625.0, 136890000.0, 138650625.0, 140422500.0, 142205625.0, 144000000.0, 145805625.0, 147622500.0, 149450625.0, 151290000.0, 153140625.0, 155002500.0, 156875625.0, 158760000.0, 160655625.0, 162562500.0, 164480625.0, 166410000.0, 168350625.0, 170302500.0, 172265625.0, 174240000.0, 176225625.0, 178222500.0, 180230625.0, 182250000.0, 184280625.0, 186322500.0, 188375625.0, 190440000.0, 192515625.0, 194602500.0, 196700625.0, 198810000.0, 200930625.0, 203062500.0, 205205625.0, 207360000.0, 209525625.0, 211702500.0, 213890625.0, 216090000.0, 218300625.0, 220522500.0, 222755625.0, 225000000.0, 227255625.0, 229522500.0, 231800625.0, 234090000.0, 236390625.0, 238702500.0, 241025625.0, 243360000.0, 245705625.0, 248062500.0, 250430625.0, 252810000.0, 255200625.0, 257602500.0, 260015625.0, 262440000.0, 264875625.0, 267322500.0, 269780625.0, 272250000.0, 274730625.0, 277222500.0, 279725625.0, 282240000.0, 284765625.0, 287302500.0, 289850625.0, 292410000.0, 294980625.0, 297562500.0, 300155625.0, 302760000.0, 305375625.0, 308002500.0, 310640625.0, 313290000.0, 315950625.0, 318622500.0, 321305625.0, 324000000.0, 326705625.0, 329422500.0, 332150625.0, 334890000.0, 337640625.0, 340402500.0, 343175625.0, 345960000.0, 348755625.0, 351562500.0, 354380625.0, 357210000.0, 360050625.0, 362902500.0, 365765625.0, 368640000.0, 371525625.0, 374422500.0, 377330625.0, 380250000.0, 383180625.0, 386122500.0, 389075625.0, 392040000.0, 395015625.0, 398002500.0, 401000625.0, 404010000.0, 407030625.0, 410062500.0, 413105625.0, 416160000.0, 419225625.0, 422302500.0, 425390625.0, 428490000.0, 431600625.0, 434722500.0, 437855625.0, 441000000.0]
  out "Altitude Array (km)":dbl[](array[numeric])=[0.075, 0.15, 0.22499999999999998, 0.3, 0.375, 0.45, 0.5249999999999999, 0.6, 0.6749999999999999, 0.7499999999999999, 0.825, 0.8999999999999999, 0.9749999999999999, 1.05, 1.125, 1.2, 1.275, 1.3499999999999999, 1.4249999999999998, 1.5, 1.575, 1.65, 1.7249999999999999, 1.7999999999999998, 1.8749999999999998, 1.95, 2.025, 2.1, 2.1750000000000003, 2.25, 2.325, 2.4, 2.475, 2.5500000000000003, 2.625, 2.7, 2.775, 2.85, 2.9250000000000003, 3.0, 3.075, 3.15, 3.225, 3.3000000000000003, 3.375, 3.45, 3.525, 3.6, 3.675, 3.75, 3.825, 3.9, 3.975, 4.05, 4.125, 4.2, 4.275, 4.35, 4.425, 4.5, 4.575, 4.65, 4.725, 4.8, 4.875, 4.95, 5.025, 5.1, 5.175, 5.25, 5.325, 5.4, 5.475, 5.55, 5.625, 5.7, 5.775, 5.85, 5.925, 6.0, 6.075, 6.15, 6.225, 6.3, 6.375, 6.45, 6.525, 6.6, 6.675, 6.75, 6.825, 6.9, 6.975, 7.05, 7.125, 7.2, 7.2749999999999995, 7.35, 7.425, 7.5, 7.575, 7.6499999999999995, 7.725, 7.8, 7.875, 7.95, 8.024999999999999, 8.1, 8.174999999999999, 8.249999999999998, 8.325, 8.399999999999999, 8.475, 8.549999999999999, 8.624999999999998, 8.7, 8.774999999999999, 8.85, 8.924999999999999, 8.999999999999998, 9.075, 9.149999999999999, 9.225, 9.299999999999999, 9.374999999999998, 9.45, 9.524999999999999, 9.6, 9.674999999999999, 9.749999999999998, 9.825, 9.899999999999999, 9.975, 10.049999999999999, 10.124999999999998, 10.2, 10.274999999999999, 10.35, 10.424999999999999, 10.499999999999998, 10.575, 10.649999999999999, 10.725, 10.799999999999999, 10.874999999999998, 10.95, 11.024999999999999, 11.1, 11.174999999999999, 11.249999999999998, 11.325, 11.399999999999999, 11.475, 11.549999999999999, 11.624999999999998, 11.7, 11.774999999999999, 11.85, 11.924999999999999, 11.999999999999998, 12.075, 12.149999999999999, 12.225, 12.299999999999999, 12.374999999999998, 12.45, 12.524999999999999, 12.6, 12.674999999999999, 12.749999999999998, 12.825, 12.899999999999999, 12.975, 13.049999999999999, 13.124999999999998, 13.2, 13.274999999999999, 13.35, 13.424999999999999, 13.499999999999998, 13.575, 13.649999999999999, 13.725, 13.799999999999999, 13.874999999999998, 13.95, 14.024999999999999, 14.1, 14.174999999999999, 14.249999999999998, 14.325, 14.399999999999999, 14.474999999999998, 14.549999999999999, 14.624999999999998, 14.7, 14.774999999999999, 14.849999999999998, 14.924999999999999, 14.999999999999998, 15.075, 15.149999999999999, 15.224999999999998, 15.299999999999999, 15.374999999999998, 15.45, 15.524999999999999, 15.599999999999998, 15.674999999999999, 15.749999999999998, 15.825, 15.899999999999999, 15.974999999999998, 16.05, 16.125, 16.2, 16.275, 16.349999999999998, 16.424999999999997, 16.5, 16.575, 16.65, 16.724999999999998, 16.799999999999997, 16.875, 16.95, 17.025, 17.099999999999998, 17.174999999999997, 17.25, 17.325, 17.4, 17.474999999999998, 17.549999999999997, 17.625, 17.7, 17.775, 17.849999999999998, 17.924999999999997, 18.0, 18.075, 18.15, 18.224999999999998, 18.299999999999997, 18.375, 18.45, 18.525, 18.599999999999998, 18.674999999999997, 18.75, 18.825, 18.9, 18.974999999999998, 19.049999999999997, 19.125, 19.2, 19.275, 19.349999999999998, 19.424999999999997, 19.5, 19.575, 19.65, 19.724999999999998, 19.799999999999997, 19.875, 19.95, 20.025, 20.099999999999998, 20.174999999999997, 20.25, 20.325, 20.4, 20.474999999999998, 20.549999999999997, 20.625, 20.7, 20.775, 20.849999999999998, 20.924999999999997, 21.0]
  in  "Instrument Control":T4(tab)=enum."Wavemeter"
  out "Readings":T5={"OnLineTEC"=19.5154362, "OnLineLD"=0.155058607, "OffLineTEC"=18.6247501, "OffLineLD"=0.150023445, "EtalonTEC"=26.3773537, "TSOA-TEC"=18.9968204, "Pro8000"=TRUE, "OnLine TEC"=TRUE, "OnLine LD"=TRUE, "OffLine TEC"=TRUE, "OffLine LD"=TRUE, "Etalon TEC"=TRUE, "TSOA TEC"=TRUE} {"OffLineLD" format="%.4g"; "OnLineLD" format="%.4g"; "TSOA-TEC" format="%.3g"; "EtalonTEC" format="%.3g"; "OffLineTEC" format="%.3g"; "OnLineTEC" format="%.3g"}
  in  "Settings":T6={"Module"=enum."On Line TEC", "OnLineTEC"=19.51161500000004, "OnLineLD"=0.155, "OffLineTEC"=18.623800000000333, "OffLineLD"=0.15, "EtalonTEC"=26.4, "TSOA-TEC"=18.0} {"OffLineLD" min=0.0 max=0.175 step=0.001 format="%.3p"; "OnLineLD" min=0.0 max=0.175 step=0.001 format="%.3p"; "TSOA-TEC" format="%.2g"; "EtalonTEC" format="%.2g"; "OffLineTEC" min=0.0 max=30.0 step=0.1 format="%.3g"; "OnLineTEC" min=0.0 max=30.0 step=0.1 format="%.3g"}
  in  "Pulse B Polarity":enum32{"Low", "High"}(ring)=enum."High"
  in  "Pulse A Delay(ns)":u32=1040 min=80 max=327600
  in  "Pulse B Delay(ns)":u32=170000 min=80 max=327600 step=1
  in  "Accumulation Delay(ns)":u32=10 min=10 max=1270 step=1
  in  "Sync Pulse Polarity":enum32{"Low", "High"}(ring)=enum."High"
  in  "Pulse A Polarity":enum32{"Low", "High"}(ring)=enum."High"
  in  "Number of Bins":u32=280 min=2 max=4095 step=1
  in  "Number of Accumulates":u32=10000 min=1 max=32767 step=1
  in  "Time Resolution Per Bin(ns)":u32=500 min=5 max=1063 step=1
  out "WM Switch":bool
  in  "Cancel online":bool
  in  "Cancel Offline":bool
  in  "Lambda On Set (nm)":dbl=828.197 format="%.5f"
  out "Lambda On Read (nm)":dbl=828.196974966175 format="%.5f"
  out "Lambda Off Read (nm)":dbl=828.2964768450829 format="%.5f"
  in  "Lambda Off Set (nm)":dbl=828.2965 format="%#.5f"
  in  "Bristol In":i32=5
  out "Bristol Out":i32=8
  in  "Online_Tol":dbl=5e-05 format="%#_15g"
  in  "Offline_Tol":dbl=5e-05 format="%#_15g"
  out "Wavelength Lock Online":bool=TRUE
  out "Wavelength Lock Offline":bool=TRUE
  out "WL Difference":dbl=-2.5033824954334705e-05 format="%_7g"
  out "WL Difference off":dbl=-2.3154917130341346e-05 format="%_7g"
  in  "calculate absorption cross sections":bool
  in  "Smoothing Range":dbl=300.0
  in  "Total DIAL Integration Time (Minutes)":i32=5
  in  "Data Reads (number of loops)":i32=1
  in  "Total Aerosol Integration Time (Minutes)":dbl=0.5
  in  "Scalar Wait Time (disabled)":u32=1300
  out "Smoothed Bins":dbl=4.0
  in  "Ophir PM On/Off":bool=TRUE
  out "OphirPM":T7={"Ophir-Ref"=refnum, "Ophir-Device"=1000, "Ophir-Channel"=0}
  out "Average Diode Power":dbl(knob)=0.0013 scale=0.0..0.002 scale format="%.1p"
  out "Ophir Samples":i32=22
  in  "Switch Comm Port":refnum<visa-resource-name>="COM3"
  out "FF_On_Ref":refnum<file>
  out "FF_On_Ptr":i64=3839264 format="%.2p"
  out "FF_Off_Ref":refnum<file>
  out "FF_Off_Ptr":i64=3839264 format="%.2p"
  out "NF_On_Ref":refnum<file>
  out "NF_On_Ptr":i64=3839264 format="%.2p"
  out "NF_Off_Ref":refnum<file>
  out "NF_Off_Ptr":i64=3839264 format="%.2p"
  out "DataOpen":bool=TRUE
  out "File Path_Far Field (out)":string="D:\\Micropulse_DIAL_data\\160714FF\\21"
  out "File Path_Near Field (out)":string="D:\\Micropulse_DIAL_data\\160714NF\\21"
  in  "Data File DIR (in)":string="D:\\Micropulse_DIAL_data\\"
  in  "WS_On/Off":bool=TRUE
  in  "WS visa":refnum<visa-resource-name>="Weather"
  out "TRHP":T8={"Temp C"=28.233974358974365, "RelH %"=31.846764346764346, "Press hPa"=842.3763736263736, "AbH g/m^3"=8.562271062271064}
  in  "ADAM6018 IP":string="192.168.0.165"
  out "T_bench":sgl=26.03952
  in  "Port":u16=502
  in  "IP Address":string="192.168.0.165"
  out "ID_out":refnum<k5>
  in  "bins":u32=280 min=2 max=4095 step=1
  out "y offset":u32=10
  in  "ns scale":u32=500
  # "ADAM6018"
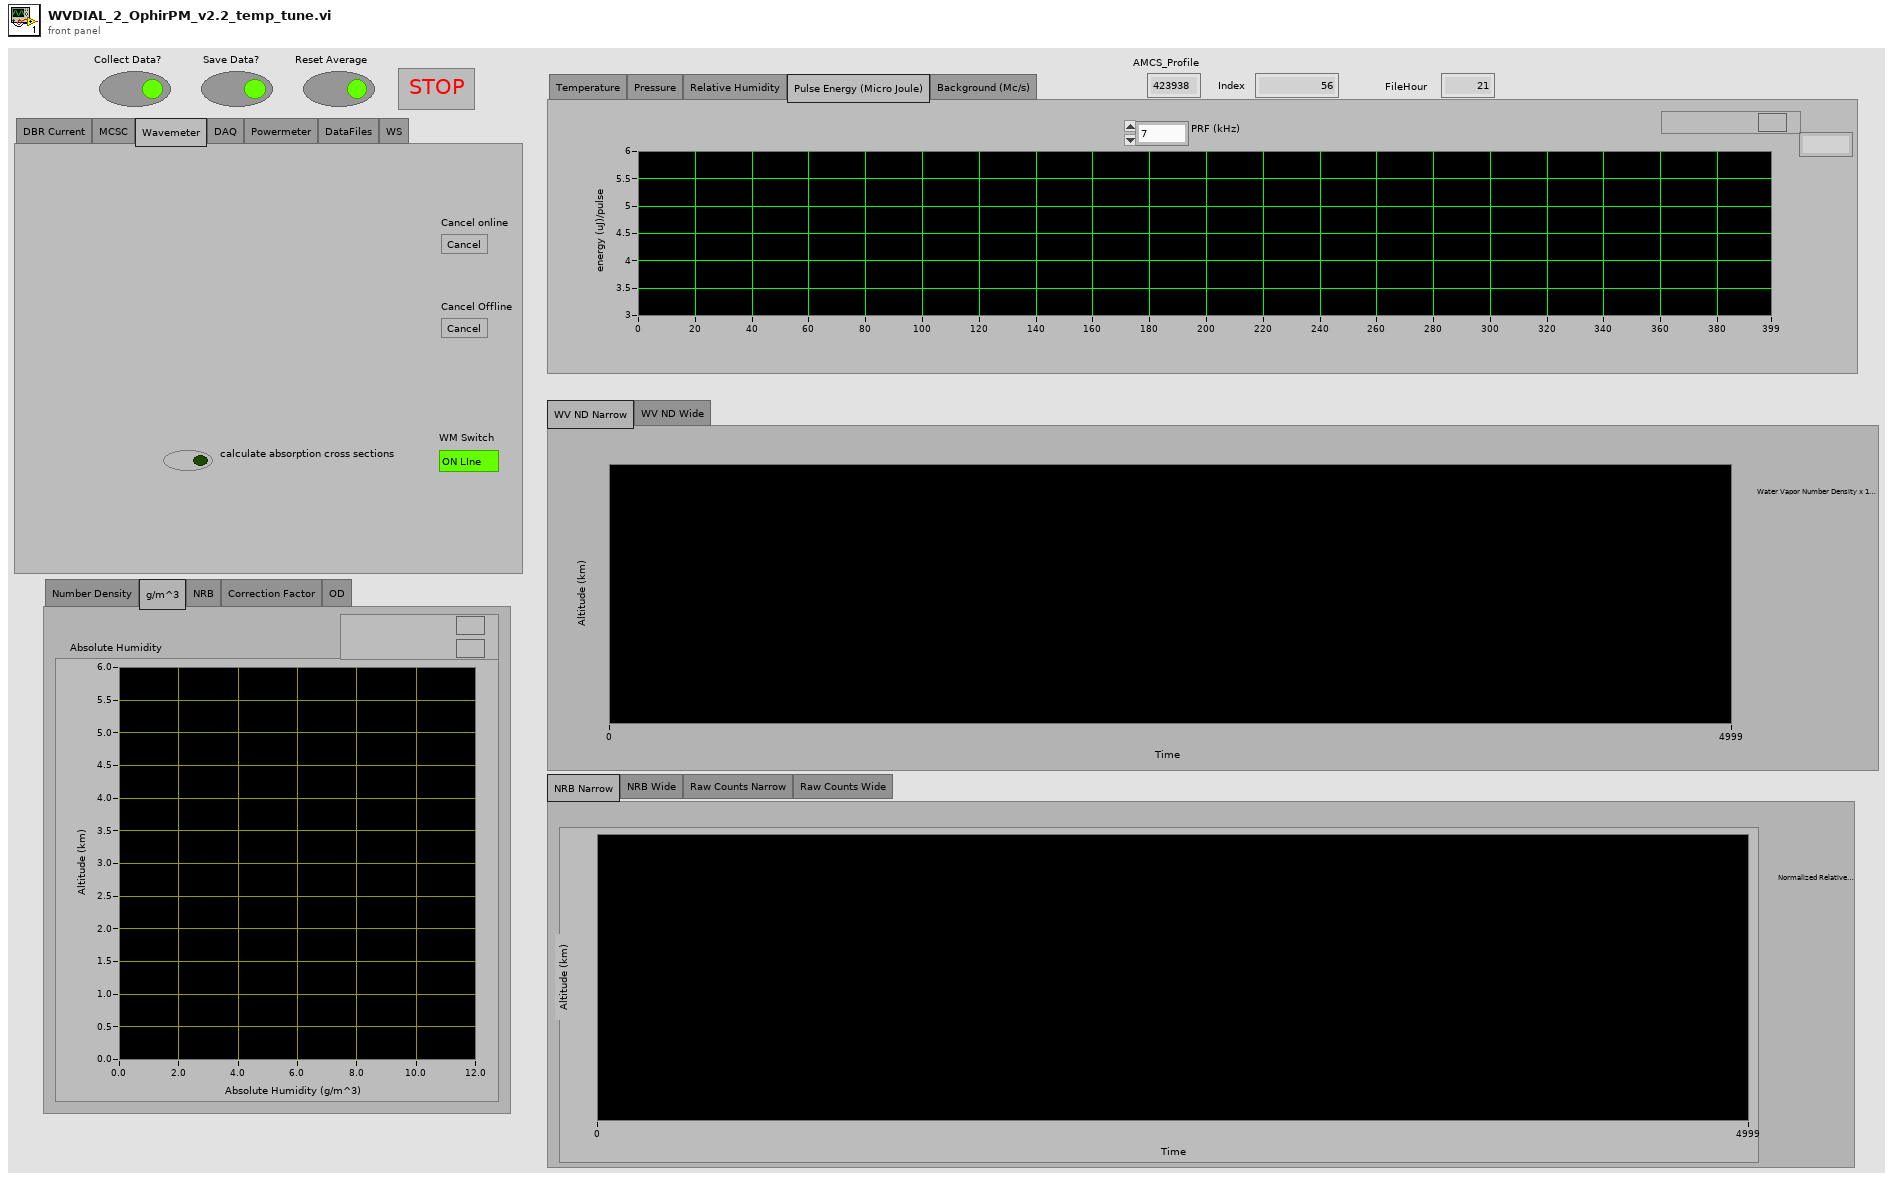
[diagram p1: front panel]
types:
  T1 = enum32{"NRB Narrow", "NRB Wide", "Raw Counts Narrow", "Raw Counts Wide"}
  T2 = enum32{"Number Density", "g/m^3", "NRB", "Correction Factor", "OD"}
  T3 = enum32{"Temperature", "Pressure", "Relative Humidity", "Pulse Energy (Micro Joule)", "Background (Mc/s)"}
  T4 = enum32{"DBR Current", "MCSC", "Wavemeter", "DAQ", "Powermeter", "DataFiles", "WS"}
  T5 = cluster{"OnLineTEC":dbl, "OnLineLD":dbl, "OffLineTEC":dbl, "OffLineLD":dbl, "EtalonTEC":dbl, "TSOA-TEC":dbl, "Pro8000":bool, "OnLine TEC":bool, "OnLine LD":bool, "OffLine TEC":bool, "OffLine LD":bool, "Etalon TEC":bool, "TSOA TEC":bool}
  T6 = cluster{"Module":enum16{"On Line TEC", "On Line LD", "Off Line TEC", "Off Line LD", "Etalon TEC", "TSOA TEC"}, "OnLineTEC":dbl, "OnLineLD":dbl, "OffLineTEC":dbl, "OffLineLD":dbl, "EtalonTEC":dbl, "TSOA-TEC":dbl}
  T7 = cluster{"Ophir-Ref":refnum<k7>, "Ophir-Device":i32, "Ophir-Channel":i32}
  T8 = cluster{"Temp C":dbl, "RelH %":dbl, "Press hPa":dbl, "AbH g/m^3":dbl}
  T9 = enum16{"Open_TL", "Close_TL", "Verify_ID", "TEC_Sensor", "SET", "READ", "ON", "OFF", "Set_Limits", "Read_Limits", "Enable_Status", "Read_Status"}
  T10 = enum16{"open", "replace", "create", "open or create", "replace or create", "replace or create with confirmation"}
  T11 = enum16{"On Line TEC", "On Line LD", "Off Line TEC", "Off Line LD", "Etalon TEC", "TSOA TEC"}
  T12 = cluster{"Temp":dbl, "RelH":dbl, "Press":dbl, "AbH":dbl}
  T13 = typedef "LVDateTimeRec.ctl" = cluster{"fractional second":dbl, "second":i32, "minute":i32, "hour":i32, "day of month":i32, "month":i32, "year":i32, "day of week":i32, "day of year":i32, "DST":i32}
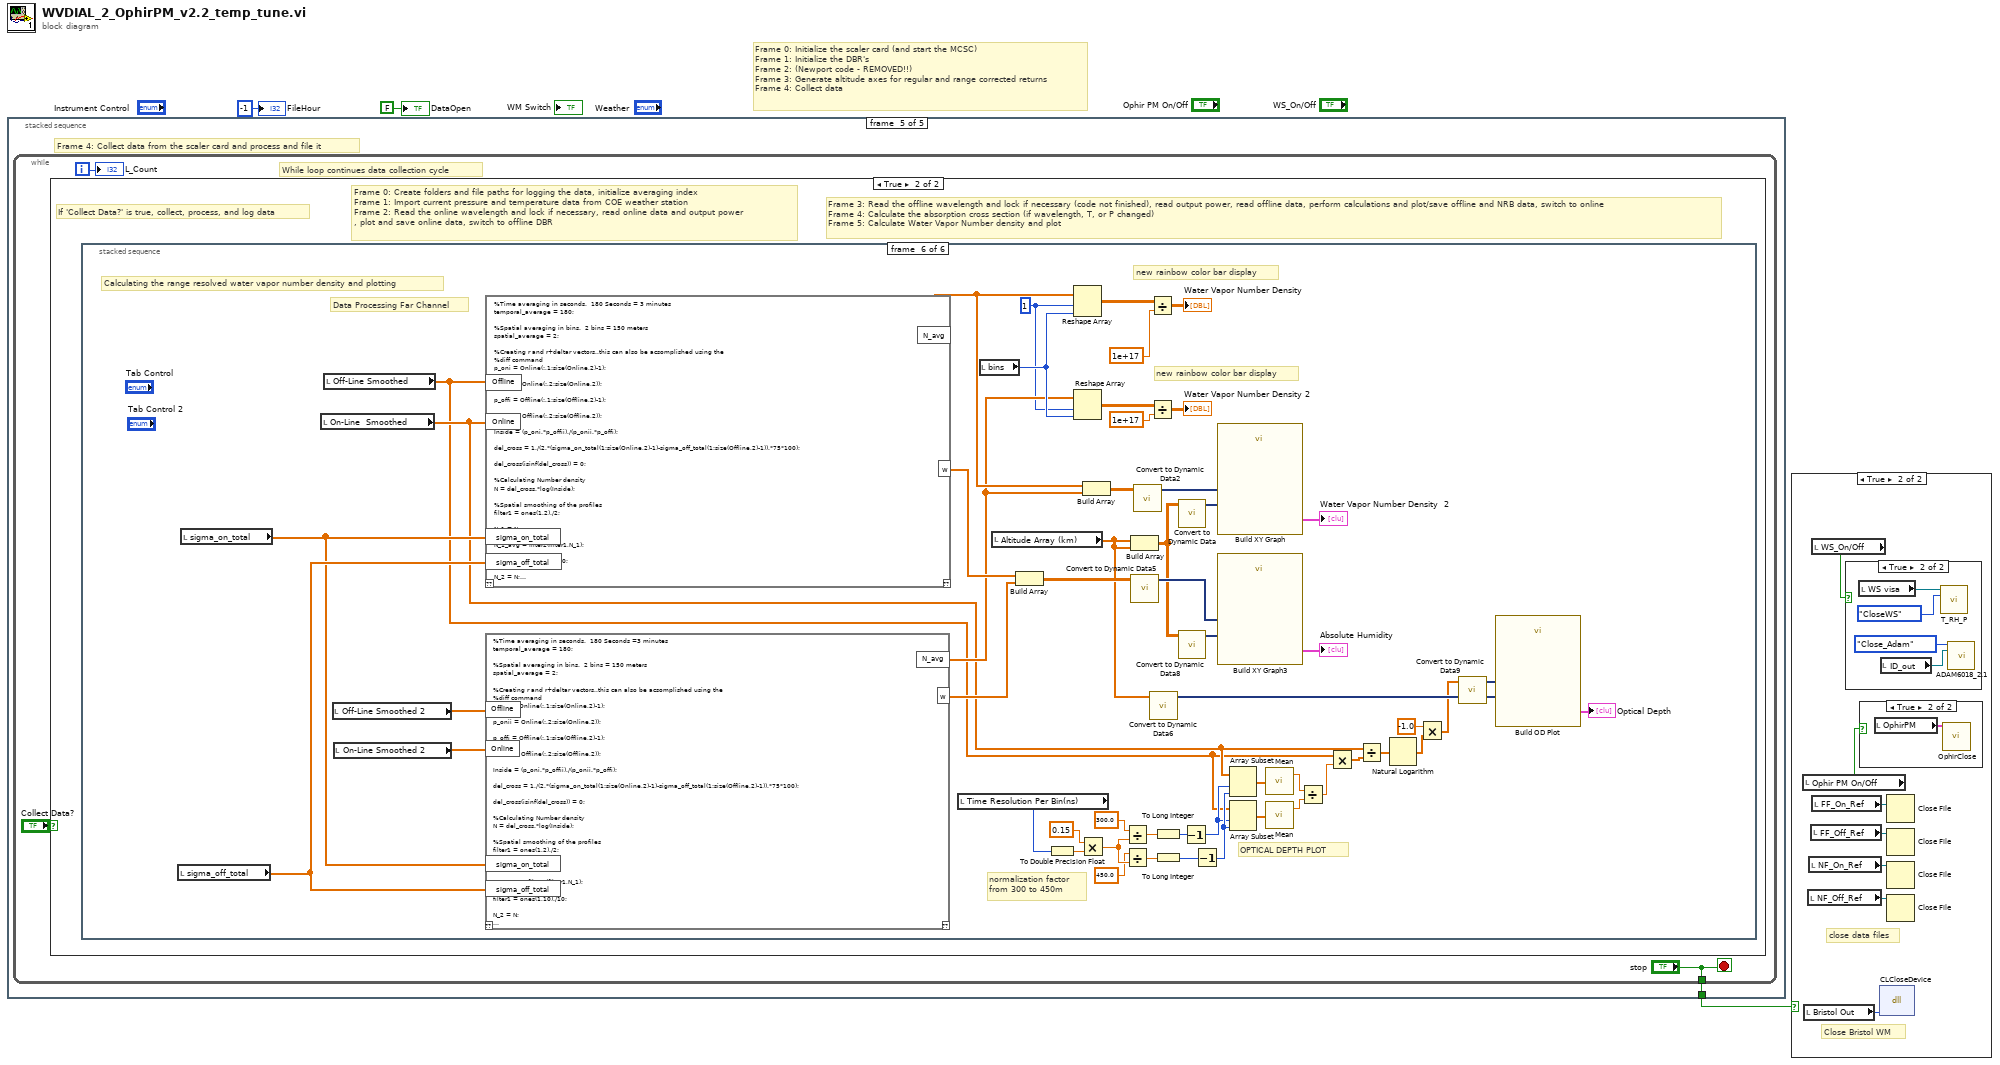
[diagram p0: block diagram]
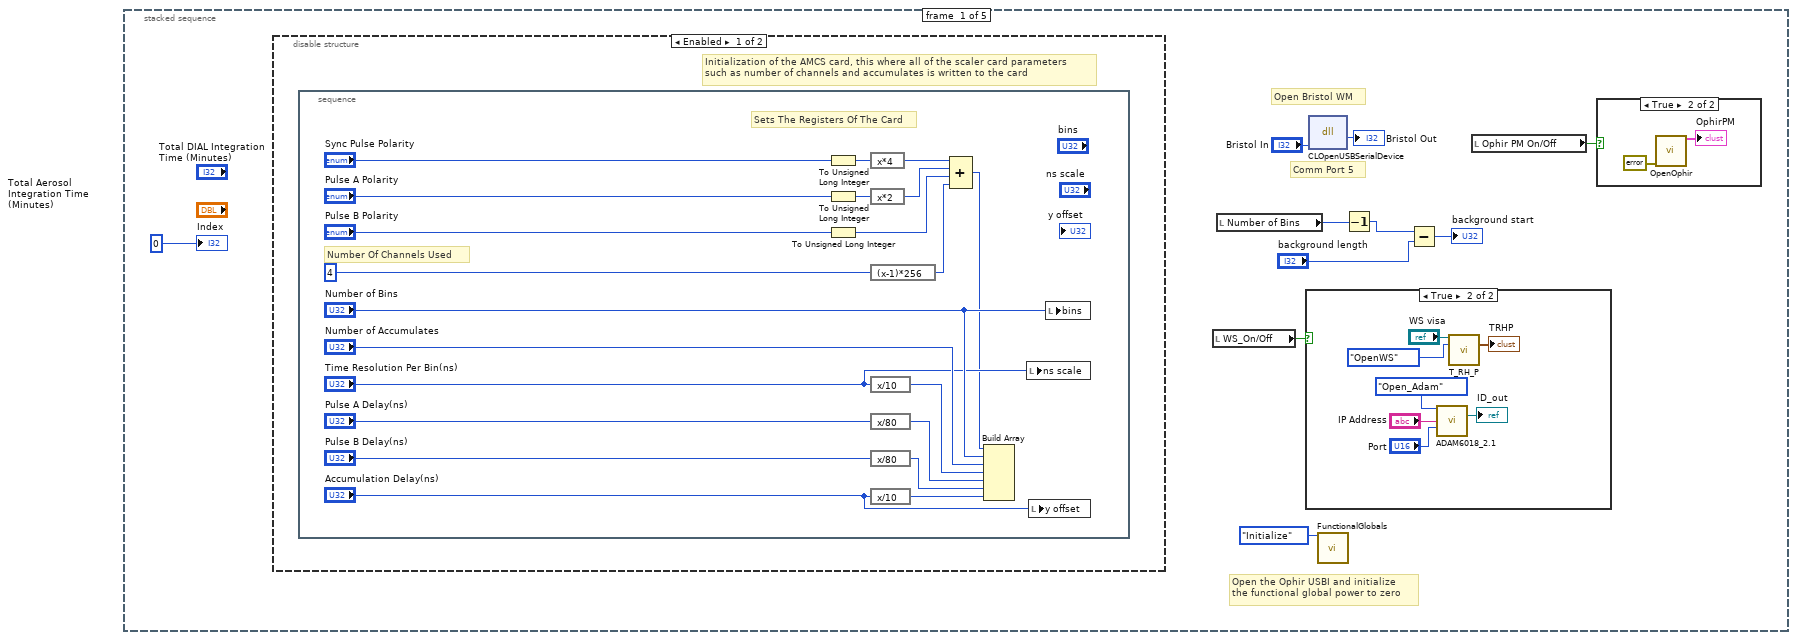
[diagram p5: hidden frame]
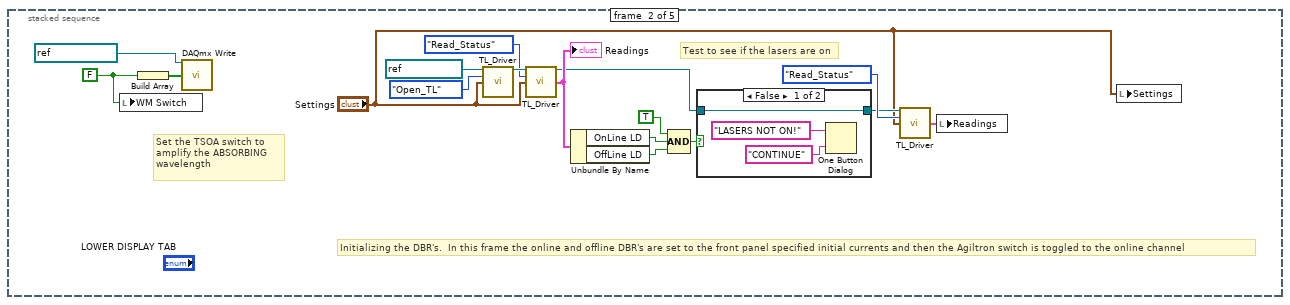
[diagram p9: hidden frame]
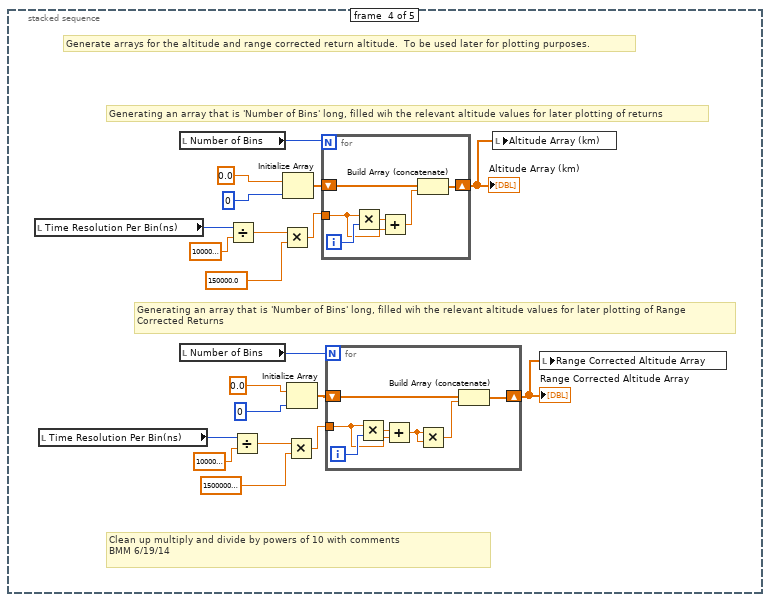
[diagram p12: hidden frame]
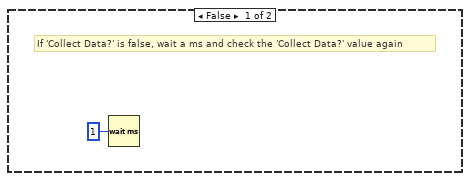
[diagram p13: hidden frame]
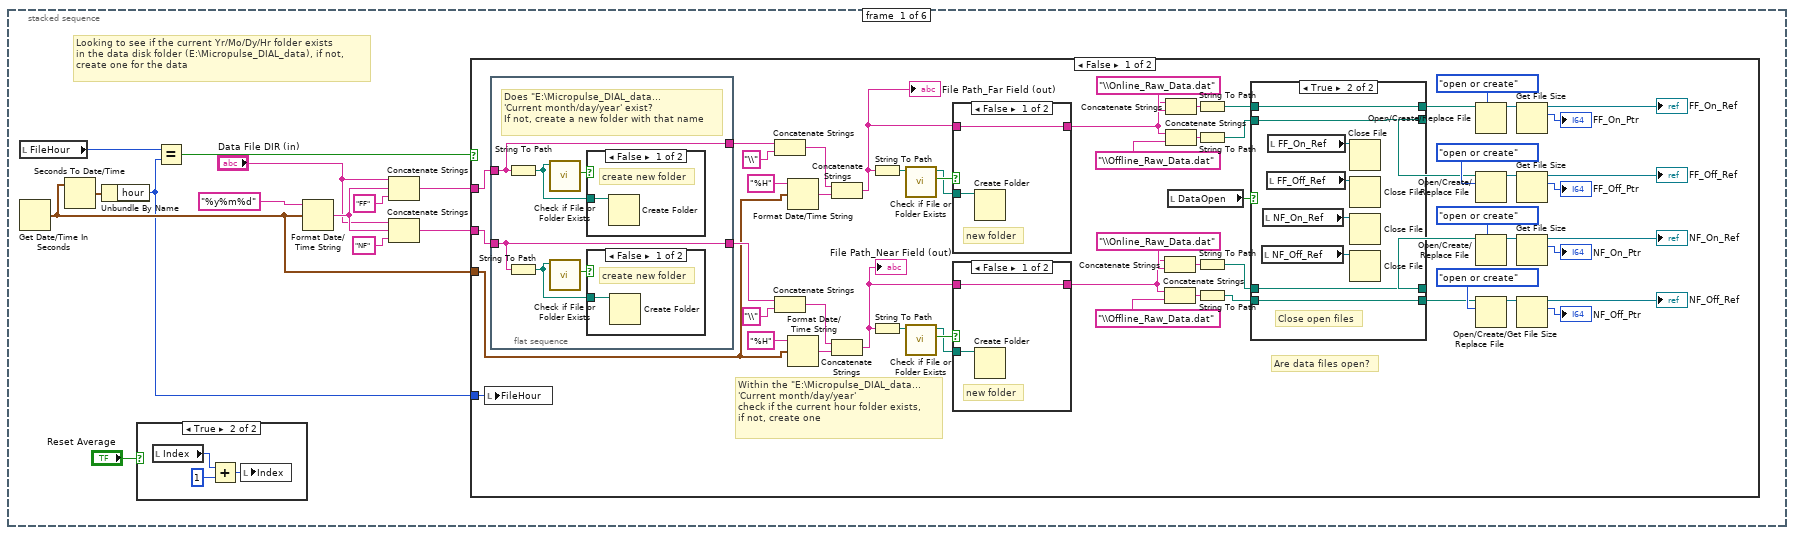
[diagram p14: hidden frame]
diagram:
  # "Frame 0: Initialize the scaler card (and start the MCSC)\nFrame 1: Initialize the DBR's\nFrame 2: (Newport code - REMOVED!!)\nFrame 3: Generate altitude axes for regular and range corrected returns\nFrame 4: Collect data"
  n1 = stacked-sequence {
    tunnel: [_ _ _ _ w98] -> w3
    frame #0 {
      # "Open the Ophir USBI and initialize\nthe functional global power to zero"
      # "Comm Port 5"
      # "Open Bristol WM"
      n2 = disable-structure shown="Enabled" {
        frame Enabled {
          # "Initialization of the AMCS card, this where all of the scaler card parameters\nsuch as number of channels and accumulates is written to the card"
          n3 = stacked-sequence {
            frame #0 {
              # "Sets The Registers Of The Card"
              # "Number Of Channels Used"
              n4 = To Unsigned Long Integer(number="Sync Pulse Polarity") -> (unsigned 32bit integer=w23:u32)
              n5 = To Unsigned Long Integer(number="Pulse A Polarity") -> (unsigned 32bit integer=w27:u32)
              n6 = To Unsigned Long Integer(number="Pulse B Polarity") -> (unsigned 32bit integer=w25:u32)
              n7 = expression code="x*4"(w23) -> (w32:u32)
              n8 = expression code="x*2"(w27) -> (w31:u32)
              n9 = expression code="(x-1)*256"(u32 4 ("Number of Channels Used")) -> (w30:u32)
              n10 = expression code="x/10"("Time Resolution Per Bin(ns)") -> (w34:u32)
              n11 = expression code="x/80"("Pulse A Delay(ns)") -> (w41:u32)
              n12 = expression code="x/80"("Pulse B Delay(ns)") -> (w43:u32)
              n13 = expression code="x/10"("Accumulation Delay(ns)") -> (w42:u32)
              n14 = Compound Arithmetic op=ADD(w32, w31, w25, w30) -> (w29:u32)
              n15 = Build Array(w29, "Number of Bins", "Number of Accumulates", w34, w41, w43, w42) -> ()  [unwired: 1 out]
              n16 = local write "ns scale"("Time Resolution Per Bin(ns)") -> ()
              n17 = local write "y offset"("Accumulation Delay(ns)") -> ()
              n18 = local write "bins"("Number of Bins") -> ()
            }
          }
        }
        frame Disabled {
        }
      }
      n19 = local read "WS_On/Off"() -> (w5:bool)
      n20 = local read "Number of Bins"() -> (w10:u32)
      n21 = case shown="True" w5 {
        frame False {
        }
        frame True {
          n22 = call "ADAM6018_2.1.vi"("ADAM6018_Command"=enum16{"Open_Adam", "Read_Adam", "Close_Adam"}."Open_Adam", "IP Address"="IP Address", "Port"="Port") -> ("ADAM_ID"=→"ID_out":refnum<k5>)  [unwired: 10 in, 2 out]
          n23 = call "T_RH_P.vi"("VISA in"="WS visa", "WS_Commands"=enum16{"OpenWS", "ReadTRHP", "CloseWS"}."OpenWS") -> ("TRHP"=→"TRHP":T12)  [unwired: 11 in, 2 out]
        }
      }
      n24 = dll-call lib="C:/H2O_DIAL/LabVIEW-2012/Bristol WM V2_31b/CLDevIface.dll" fn="CLOpenUSBSerialDevice"("commPort"="Bristol In") -> ("return type"=→"Bristol Out":i32)  [unwired: 4 in, 2 out]
      n25 = call "FunctionalGlobals.vi"("FG_Control"=enum16{"Initialize", "PowerRead", "PowerWrite"}."Initialize") -> ()  [unwired: 14 in, 1 out]
      n26 = Decrement(x=w10) -> (x-1=w9:u32)
      n27 = Subtract(x=w9, y="background length") -> (x-y=→"background start":u32)
      n28 = local read "Ophir PM On/Off"() -> (w4:bool)
      n29 = case shown="True" w4 {
        frame False {
        }
        frame True {
          n30 = call "OpenOphir.vi"("error in (no error)"=errorcluster {"status"=FALSE, "code"=0, "source"=""}) -> ("OphirPM"=→"OphirPM":T7)  [unwired: 13 in, 1 out]
        }
      }
      "Index" <- 0 ("Index")
    }
    frame #1 {
      w44 = FALSE ("Boolean")
      # "Test to see if the lasers are on"
      # "Set the TSOA switch to\namplify the ABSORBING\nwavelength"
      # "Initializing the DBR's.  In this frame the online and offline DBR's are set to the front panel specified initial currents and then the Agiltron switch is toggled to the online channel"
      n31 = local write "WM Switch"(w44) -> ()
      n32 = Build Array(w44) -> (w46:bool[])
      n33 = call-poly <vilib>:"DAQmx Write.vi"("task/channels in"=refnum<k21> "BristolWM", "data"=w46) -> ()  [unwired: 11 in, 3 out]
      n34 = call "TL_Driver.vi"("Device In"=refnum<visa-resource-name> "ThorLabs", "Commands"=T9."Open_TL", "Settings"="Settings") -> ("Device Out"=w58:refnum<visa-resource-name>)  [unwired: 9 in, 3 out]
      n35 = call "TL_Driver.vi"("Device In"=w58, "Commands"=T9."Read_Status", "Settings"="Settings") -> ("Device Out"=w55:refnum<visa-resource-name>, "Readings"=w56:T5)  [unwired: 9 in, 2 out]
      "Readings" <- w56
      n36 = Unbundle By Name(w56) -> ("OnLine LD"=w50:bool, "OffLine LD"=w51:bool)
      n37 = Compound Arithmetic op=AND(TRUE, w50, w51) -> (w49:bool)
      n38 = case shown="False" w49 {
        tunnel: w55 -> [w61 w64]
        tunnel: [w61 w64] -> w53
        frame False {
          n39 = One Button Dialog(message="LASERS NOT ON!", button name ("OK")="CONTINUE") -> ()  [unwired: 1 out]
        }
        frame True {
        }
      }
      n40 = call "TL_Driver.vi"("Device In"=w53, "Commands"=T9."Read_Status", "Settings"="Settings") -> ("Readings"=w45:T5)  [unwired: 9 in, 3 out]
      n41 = local write "Readings"(w45) -> ()
      n42 = local write "Settings"("Settings") -> ()
    }
    frame #2 {
      # "NEWPORT CODE REMOVED!!!!"
    }
    frame #3 {
      # "Clean up multiply and divide by powers of 10 with comments\nBMM 6/19/14"
      # "Generating an array that is 'Number of Bins' long, filled wih the relevant altitude values for later plotting of Range \nCorrected Returns"
      # "Generating an array that is 'Number of Bins' long, filled wih the relevant altitude values for later plotting of returns"
      # "Generate arrays for the altitude and range corrected return altitude.  To be used later for plotting purposes."
      n43 = local read "Time Resolution Per Bin(ns)"() -> (w77:u32)
      n44 = local read "Time Resolution Per Bin(ns)"() -> (w67:u32)
      n45 = local read "Number of Bins"() -> (w80:u32)
      n46 = local read "Number of Bins"() -> (w70:u32)
      n47 = Divide(x=w77, y=1000000000.0) -> (x/y=w75:dbl)
      n48 = Divide(x=w67, y=1000000000.0) -> (x/y=w65:dbl)
      n49 = Multiply(x=w75, y=150000.0) -> (x*y=w78:dbl)
      n50 = Initialize Array(0.0, 0) -> (w83:dbl[])
      n51 = Multiply(x=w65, y=150000000.0) -> (x*y=w68:dbl)
      n52 = Initialize Array(0.0, 0) -> (w73:dbl[])
      n53 = for {
        N: w80 -> [_]
        shift-right: [w96] -> w81
        shift-left: w83 -> [w97]
        tunnel: w78 -> [w93]
        i -> [w95]
        n54 = Multiply(x=w93, y=w95) -> (x*y=w94:dbl)
        n55 = Add(x=w94, y=w93) -> (x+y=w92:dbl)
        n56 = Build Array (concatenate)(w97, w92) -> (w96:dbl[])
      }
      "Altitude Array (km)" <- w81
      n57 = for {
        N: w70 -> [_]
        shift-right: [w90] -> w71
        shift-left: w73 -> [w91]
        tunnel: w68 -> [w86]
        i -> [w89]
        n58 = Multiply(x=w86, y=w89) -> (x*y=w87:dbl)
        n59 = Add(x=w87, y=w86) -> (x+y=w85:dbl)
        n60 = Multiply(x=w85, y=w85) -> (x*y=w88:dbl)
        n61 = Build Array (concatenate)(w91, w88) -> (w90:dbl[])
      }
      "Range Corrected Altitude Array" <- w71
      n62 = local write "Altitude Array (km)"(w81) -> ()
      n63 = local write "Range Corrected Altitude Array"(w71) -> ()
    }
    frame #4 {
      # "Frame 4: Collect data from the scaler card and process and file it"
      n64 = while {
        tunnel: ["stop"] -> w98
        i -> [w99]
        stop <- "stop" stop-if-true
        # "While loop continues data collection cycle"
        n65 = case shown="True" "Collect Data?" {
          frame False {
            # "If 'Collect Data?' is false, wait a ms and check the 'Collect Data?' value again"
            n66 = Wait (ms)(milliseconds to wait=u32 1) -> ()  [unwired: 1 out]
          }
          frame True {
            # "Frame 3: Read the offline wavelength and lock if necessary (code not finished), read output power, read offline data, perform calculations and plot/save offline and NRB data, switch to online\nFrame 4: Calculate the absorption cross section (if wavelength, T, or P changed)\nFrame 5: Calculate Water Vapor Number density and plot"
            # "Frame 0: Create folders and file paths for logging the data, initialize averaging index\nFrame 1: Import current pressure and temperature data from COE weather station\nFrame 2: Read the online wavelength and lock if necessary, read online data and output power\n, plot and save online data, switch to offline DBR"
            # "If 'Collect Data?' is true, collect, process, and log data"
            n67 = stacked-sequence {
              frame #0 {
                # "Looking to see if the current Yr/Mo/Dy/Hr folder exists\nin the data disk folder (E:\\Micropulse_DIAL_data), if not,\ncreate one for the data"
                n68 = local read "FileHour"() -> (w112:i32)
                n69 = Get Date/Time In Seconds() -> (seconds since 1Jan1904=w104:timestamp)
                n70 = Seconds To Date/Time(time stamp (now)=w104) -> (date time rec=w114:T13)  [unwired: 1 in]
                n71 = Unbundle By Name(w114) -> ("hour"=w103:i32)
                n72 = case shown="True" "Reset Average" {
                  frame False {
                    n73 = local write "Index"(0 ("Index")) -> ()
                  }
                  frame True {
                    n74 = local read "Index"() -> (w202:i32)
                    n75 = Add(x=w202, y=1) -> (x+y=w201:i32)
                    n76 = local write "Index"(w201) -> ()
                  }
                }
                n77 = Equal?(x=w112, y=w103) -> (x = y?=w113:bool)
                n78 = Format Date/Time String(time format string (%c)="%y%m%d", seconds (now)=w104) -> (date/time string=w108:string)  [unwired: 1 in]
                n79 = Concatenate Strings("Data File DIR (in)", w108, "FF" ("string")) -> (w110:string)
                n80 = Concatenate Strings("Data File DIR (in)", w108, "NF" ("string")) -> (w105:string)
                n81 = case shown="False" w113 {
                  tunnel: w110 -> [w172 _]
                  tunnel: w105 -> [w171 _]
                  tunnel: w104 -> [w158 _]
                  tunnel: w103 -> [w134 _]
                  frame False {
                    # "Are data files open?"
                    # "Within the \"E:\\Micropulse_DIAL_data...\n'Current month/day/year' \ncheck if the current hour folder exists,\nif not, create one"
                    n82 = local write "FileHour"(w134) -> ()
                    n83 = flat-sequence {
                      tunnel: [w192] -> w159
                      tunnel: w172 -> [w191]
                      tunnel: w171 -> [w192]
                      tunnel: [w191] -> w160
                      frame #0 {
                        # "Does \"E:\\Micropulse_DIAL_data...\n'Current month/day/year' exist?\nIf not, create a new folder with that name"
                        n84 = String To Path(string=w191) -> (path=w196:path)
                        n85 = String To Path(string=w192) -> (path=w194:path)
                        n86 = call <vilib>:"Check if File or Folder Exists.vi"("path"=w196) -> ("file or folder exists?"=w195:bool)  [unwired: 8 in, 2 out]
                        n87 = call <vilib>:"Check if File or Folder Exists.vi"("path"=w194) -> ("file or folder exists?"=w193:bool)  [unwired: 8 in, 2 out]
                        n88 = case shown="False" w195 {
                          tunnel: w196 -> [w198 _]
                          frame False {
                            # "create new folder"
                            n89 = Create Folder(path (use dialog)=w198) -> ()  [unwired: 2 in, 3 out]
                          }
                          frame True {
                            # "Folder exists\ndo nothing"
                          }
                        }
                        n90 = case shown="False" w193 {
                          tunnel: w194 -> [w197 _]
                          frame False {
                            # "create new folder"
                            n91 = Create Folder(path (use dialog)=w197) -> ()  [unwired: 2 in, 3 out]
                          }
                          frame True {
                            # "Folder exists\ndo nothing"
                          }
                        }
                      }
                    }
                    n92 = Concatenate Strings(w160, "\\" ("string")) -> (w167:string)
                    n93 = Concatenate Strings(w159, "\\" ("string")) -> (w162:string)
                    n94 = Format Date/Time String(time format string (%c)="%H", seconds (now)=w158) -> (date/time string=w170:string)  [unwired: 1 in]
                    n95 = Format Date/Time String(time format string (%c)="%H", seconds (now)=w158) -> (date/time string=w165:string)  [unwired: 1 in]
                    n96 = Concatenate Strings(w167, w170) -> (w130:string)
                    "File Path_Far Field (out)" <- w130
                    n97 = Concatenate Strings(w162, w165) -> (w131:string)
                    "File Path_Near Field (out)" <- w131
                    n98 = String To Path(string=w130) -> (path=w168:path)
                    n99 = String To Path(string=w131) -> (path=w163:path)
                    n100 = call <vilib>:"Check if File or Folder Exists.vi"("path"=w168) -> ("file or folder exists?"=w157:bool, "dup path"=w155:path)  [unwired: 8 in, 1 out]
                    n101 = call <vilib>:"Check if File or Folder Exists.vi"("path"=w163) -> ("file or folder exists?"=w156:bool, "dup path"=w154:path)  [unwired: 8 in, 1 out]
                    n102 = case shown="False" w157 {
                      tunnel: w155 -> [w189 _]
                      tunnel: w130 -> [w188 w190]
                      tunnel: [w188 w190] -> w128
                      frame False {
                        # "new folder"
                        n103 = Create Folder(path (use dialog)=w189) -> ()  [unwired: 2 in, 3 out]
                      }
                      frame True {
                        # "Folder exists\ndo nothing"
                      }
                    }
                    n104 = case shown="False" w156 {
                      tunnel: w154 -> [w186 _]
                      tunnel: w131 -> [w185 w187]
                      tunnel: [w185 w187] -> w129
                      frame False {
                        # "new folder"
                        n105 = Create Folder(path (use dialog)=w186) -> ()  [unwired: 2 in, 3 out]
                      }
                      frame True {
                        # "Folder exists\ndo nothing"
                      }
                    }
                    n106 = Concatenate Strings(w129, "\\Online_Raw_Data.dat" ("string")) -> (w148:string)
                    n107 = Concatenate Strings(w129, "\\Offline_Raw_Data.dat" ("string")) -> (w147:string)
                    n108 = Concatenate Strings(w128, "\\Online_Raw_Data.dat" ("string")) -> (w153:string)
                    n109 = Concatenate Strings(w128, "\\Offline_Raw_Data.dat" ("string")) -> (w152:string)
                    n110 = local read "DataOpen"() -> (w145:bool)
                    n111 = String To Path(string=w153) -> (path=w144:path)
                    n112 = String To Path(string=w152) -> (path=w143:path)
                    n113 = String To Path(string=w148) -> (path=w142:path)
                    n114 = String To Path(string=w147) -> (path=w141:path)
                    n115 = case shown="True" w145 {
                      tunnel: w144 -> [w176 w180]
                      tunnel: [w176 w180] -> w138
                      tunnel: w143 -> [w175 w179]
                      tunnel: [w175 w179] -> w137
                      tunnel: w142 -> [w174 w178]
                      tunnel: [w174 w178] -> w136
                      tunnel: [w173 w177] -> w135
                      tunnel: w141 -> [w173 w177]
                      frame False {
                        # "No files open\ndo nothing"
                      }
                      frame True {
                        # "Close open files"
                        n116 = local read "NF_Off_Ref"() -> (w182:refnum<file>)
                        n117 = local read "NF_On_Ref"() -> (w181:refnum<file>)
                        n118 = local read "FF_Off_Ref"() -> (w184:refnum<file>)
                        n119 = local read "FF_On_Ref"() -> (w183:refnum<file>)
                        n120 = Close File(refnum=w183) -> ()  [unwired: 1 in, 2 out]
                        n121 = Close File(refnum=w184) -> ()  [unwired: 1 in, 2 out]
                        n122 = Close File(refnum=w181) -> ()  [unwired: 1 in, 2 out]
                        n123 = Close File(refnum=w182) -> ()  [unwired: 1 in, 2 out]
                      }
                    }
                    n124 = Open/Create/Replace File(file path (use dialog)=w138, operation (0:open)=T10."open or create") -> (refnum out=w124:refnum<file>)  [unwired: 4 in, 2 out]
                    n125 = Open/Create/Replace File(file path (use dialog)=w137, operation (0:open)=T10."open or create") -> (refnum out=w125:refnum<file>)  [unwired: 4 in, 2 out]
                    n126 = Open/Create/Replace File(file path (use dialog)=w136, operation (0:open)=T10."open or create") -> (refnum out=w126:refnum<file>)  [unwired: 4 in, 2 out]
                    n127 = Open/Create/Replace File(file path (use dialog)=w135, operation (0:open)=T10."open or create") -> (refnum out=w127:refnum<file>)  [unwired: 4 in, 2 out]
                    n128 = Get File Size(file=w124) -> (refnum out=→"FF_On_Ref":refnum<file>, size (in bytes)=→"FF_On_Ptr":i64)  [unwired: 1 in, 1 out]
                    n129 = Get File Size(file=w125) -> (refnum out=→"FF_Off_Ref":refnum<file>, size (in bytes)=→"FF_Off_Ptr":i64)  [unwired: 1 in, 1 out]
                    n130 = Get File Size(file=w126) -> (refnum out=→"NF_On_Ref":refnum<file>, size (in bytes)=→"NF_On_Ptr":i64)  [unwired: 1 in, 1 out]
                    n131 = Get File Size(file=w127) -> (refnum out=→"NF_Off_Ref":refnum<file>, size (in bytes)=→"NF_Off_Ptr":i64)  [unwired: 1 in, 1 out]
                  }
                  frame True {
                    # "Don't need to do anything!"
                  }
                }
              }
              frame #1 {
                # "Writing and plotting retrieved\nweather parameters"
                # "Matlab script goes online and retrieves most recent press, temp, and relative humidity data \nfrom the weather station on the roof of Cobleigh"
                # "Importing the current weather conditions from the COE weather station"
                n132 = disable-structure shown="Disabled" {
                  frame Disabled {
                    n133 = script code="%try\n%s=urlread('http://www.coe.montana.edu/ee/weather/mostCurrentCSV.php');\n%amin=textscan(s,'%s %s %s %s %s %s %s %s %s %s %s %s %s');\n%data=amin{1}{2};\n%[test remain]=strtok(data,',');\n%remain=str2num(remain);\n%press=remain(3)./1000;\n%temp=remain(5);\n%RH=remain(7);\n%catch\npress=.850;\ntemp=20;\nRH=40;\n%end"() -> ()  [unwired: 1 in, 4 out]
                  }
                  frame Enabled {
                  }
                }
                n134 = local read "WS_On/Off"() -> (w203:bool)
                n135 = case shown="True" w203 {
                  frame False {
                  }
                  frame True {
                    n136 = disable-structure shown="Disabled" {
                      frame Disabled {
                        n137 = call "ADAM6018.vi"("Remote IP Address 2"="ADAM6018 IP") -> ()  [unwired: 10 in, 1 out]
                      }
                      frame Enabled {
                      }
                    }
                    n138 = local read "WS visa"() -> (w213:refnum<visa-resource-name>)
                    n139 = call "T_RH_P.vi"("VISA in"=w213, "WS_Commands"=enum16{"OpenWS", "ReadTRHP", "CloseWS"}."ReadTRHP") -> ("TRHP"=w208:T12)  [unwired: 11 in, 2 out]
                    n140 = local read "ID_out"() -> (w206:refnum<k5>)
                    n141 = Unbundle By Name(w208) -> ("Temp"=→"Temperature (C)":dbl, "RelH"=→"Relative Humdity (%)":dbl, "Press"=→"Pressure (mb)":dbl)
                    n142 = call "ADAM6018_2.1.vi"("ADAM6018_Command"=enum16{"Open_Adam", "Read_Adam", "Close_Adam"}."Read_Adam", "ID_in"=w206) -> ("Temps"=w207:sgl[])  [unwired: 11 in, 2 out]
                    n143 = local write "TRHP"(w208) -> ()
                    n144 = Index Array(array=w207) -> (element #3=→"T_bench":sgl)  [unwired: 8 in, 7 out]
                  }
                }
              }
              frame #2 {
                # "Frame 3: Read, process, and plot online data\nFrame 4: Switch to the offline DBR seed\nFrame 5: Write the data to the folders from Frame 0 of outter sequence"
                # "Frame 0: Read the online wavelength and adjust to locking tolerance if out of range\nFrame 1: Read the output power from the Newport meter, calculate and plot the output pulse energy\nFrame 2: Wait 'Scalar Wait Time' for buffer to clear other wavelength data"
                # "Online"
                n145 = stacked-sequence {
                  frame #0 {
                    # "Read the online wavelength and continue adjusting the online DBR if outside the wavelength tolerance\nuntil it is within tolerance"
                    n146 = while {
                      i -> [w218]
                      stop <- w216 stop-if-true
                      # "Frame 2: Decrement DBR current if above tolerance\nFrame 3: Increment DBR current if below tolerance"
                      # "Frame 0: Read the current wavelength from the wavemeter\nFrame 1: Calculate the difference between desired and actual wavelength"
                      # "Continue reading and adjusting online DBR current until within locking tolerance"
                      n147 = stacked-sequence {
                        tunnel: w218 -> [w220 _ _ _ _]
                        tunnel: [_ _ w227 _ _] -> w217
                        frame #0 {
                          n148 = Equal To 0?(x=w220) -> (x = 0?=w219:bool)
                          n149 = case shown="True" w219 {
                            frame False {
                            }
                            frame True {
                              w221 = FALSE ("Boolean")
                              # "SWITCH to ABSORBING"
                              n150 = Build Array(w221) -> (w222:bool[])
                              n151 = local write "WM Switch"(w221) -> ()
                              n152 = call-poly <vilib>:"DAQmx Write.vi"("task/channels in"=refnum<k21> "BristolWM", "data"=w222) -> ()  [unwired: 11 in, 3 out]
                            }
                          }
                        }
                        frame #1 {
                          # "Read Bristol WM"
                          n153 = local read "Bristol Out"() -> (w224:i32)
                          n154 = dll-call lib="C:/H2O_DIAL/LabVIEW-2012/Bristol WM V2_31b/CLDevIface.dll" fn="CLGetLambdaReading"("devHandle"=w224) -> ("return type"=→"Lambda On Read (nm)":dbl)  [unwired: 4 in, 2 out]
                        }
                        frame #2 {
                          # "If WL difference is within tolerance, stop looping, and illuminate 'Wavelength Lock Online' indicator"
                          # "Calculating the difference between the actual and desired online wavelength"
                          n155 = local read "Lambda On Read (nm)"() -> (w234:dbl)
                          n156 = local read "Online_Tol"() -> (w231:dbl)
                          n157 = Subtract(x=w234, y="Lambda On Set (nm)") -> (x-y=w226:dbl)
                          "WL Difference" <- w226
                          n158 = Multiply(x=-1.0, y=w231) -> (x*y=w232:dbl)
                          n159 = Greater?(x=w226, y=w232) -> (0:w228:bool)
                          n160 = Less?(x=w226, y=w231) -> (x < y?=w229:bool)
                          n161 = And(x=w228, y=w229) -> (x .and. y?=w227:bool)
                          "Wavelength Lock Online" <- w227
                        }
                        frame #3 {
                          # "If the wavelength difference is greater that 0.0002 nm, decrement the \nDBR current by 0.01 mA"
                          n162 = local read "WL Difference"() -> (w237:dbl)
                          n163 = Greater Or Equal?(x=w237, y="Online_Tol") -> (x >= y?=w235:bool)
                          n164 = case shown="True" w235 {
                            frame False {
                              # "Wavelength difference is not greater than 0.0002 nm, do nothing"
                            }
                            frame True {
                              # "Generating a command string\nto decrement the current"
                              # "WL difference is greater than 0.0002 nm,\ndecrement the DBR current by 0.01 mA"
                              n165 = local read "Settings"() -> (w242:T6)
                              n166 = Unbundle By Name(w242) -> ("OnLineTEC"=w244:dbl)
                              n167 = Subtract(x=w244, y=0.00012) -> (x-y=w245:dbl)
                              n168 = Bundle By Name(cluster=w242, "OnLineTEC"=w245, "Module"=T11."On Line TEC") -> (w240:T6)
                              n169 = call "TL_Driver.vi"("Device In"=refnum<visa-resource-name> "ThorLabs", "Commands"=T9."SET", "Settings"=w240) -> ("Readings"=w238:T5)  [unwired: 9 in, 3 out]
                              n170 = local write "Settings"(w240) -> ()
                              n171 = local write "Readings"(w238) -> ()
                            }
                          }
                        }
                        frame #4 {
                          # "If the wavelength difference is less that 0.0002 nm, increment the \nDBR current by 0.01 mA"
                          n172 = local read "WL Difference"() -> (w251:dbl)
                          n173 = local read "Online_Tol"() -> (w249:dbl)
                          n174 = Multiply(x=-1.0, y=w249) -> (x*y=w247:dbl)
                          n175 = Less Or Equal?(x=w251, y=w247) -> (x <= y?=w250:bool)
                          n176 = case shown="True" w250 {
                            frame False {
                              # "WL difference is no <= to -0.0002 nm, do nothing"
                            }
                            frame True {
                              # "WL difference is < -0.0002,\nincrement the DBR current by 0.01 mA"
                              # "Generating a command string\nto decrement the current"
                              n177 = local read "Settings"() -> (w256:T6)
                              n178 = Unbundle By Name(w256) -> ("OnLineTEC"=w258:dbl)
                              n179 = Add(x=w258, y=0.00012) -> (x+y=w259:dbl)
                              n180 = Bundle By Name(cluster=w256, "OnLineTEC"=w259, "Module"=T11."On Line TEC") -> (w253:T6)
                              n181 = call "TL_Driver.vi"("Device In"=refnum<visa-resource-name> "ThorLabs", "Commands"=T9."SET", "Settings"=w253) -> ("Readings"=w252:T5)  [unwired: 9 in, 3 out]
                              n182 = local write "Settings"(w253) -> ()
                              n183 = local write "Readings"(w252) -> ()
                            }
                          }
                        }
                      }
                      n184 = Or(x=w217, y="Cancel online") -> (x .or. y?=w216:bool)
                    }
                  }
                  frame #1 {
                    # "Reading the output power of the laser transmitter from the Ophir power meter, once read, convert to corresponding pulse energy and plot"
                    n185 = local read "Ophir PM On/Off"() -> (w261:bool)
                    n186 = case shown="True" w261 {
                      frame False {
                      }
                      frame True {
                        # "Plotting the online and offling pulse energies"
                        # "Converting to pulse energy, assumes 5 percent pickoff"
                        n187 = local read "OphirPM"() -> (w266:T7)
                        n188 = call "OphirRead.vi"("OphirPM"=w266) -> ("Power (W)"=w262:dbl, "Ophir Samples"=→"Ophir Samples":i32)  [unwired: 12 in, 1 out]
                        "Average Diode Power" <- w262
                        n189 = Multiply(x=w262, y=1000.0) -> (x*y=w270:dbl)
                        n190 = Divide(x=w270, y=0.05) -> (x/y=w268:dbl)
                        n191 = Divide(x=w268, y="PRF (kHz)") -> (x/y=w263:dbl)
                        n192 = Bundle(w263) -> (→"Pulse Energy (Micro Joule)":cluster{dbl})  [unwired: 1 in]
                      }
                    }
                  }
                  frame #2 {
                    # "Wait 'Scalar Wait Time' for the next available batch of scalar card data"
                    n193 = local read "AMCS_Profile"() -> (w272:i32)
                    n194 = disable-structure shown="Disabled" {
                      frame Disabled {
                        # "Waiting 'Scalar Wait Time'"
                        n195 = Wait (ms)(milliseconds to wait="Scalar Wait Time (disabled)") -> ()  [unwired: 1 out]
                      }
                      frame Enabled {
                      }
                    }
                    n196 = while {
                      tunnel: [w279] -> w273
                      tunnel: [w275] -> _
                      tunnel: w272 -> [w275]
                      stop <- w277 stop-if-true
                      n197 = global read "AMCS_Data.vi" "AMCS_Profile"() -> (w279:i32)
                      n198 = Wait (ms)(milliseconds to wait=u32 10) -> ()  [unwired: 1 out]
                      n199 = Equal?(x=w279, y=w275) -> (x = y?=w278:bool)
                      n200 = case shown="False" w278 {
                        tunnel: [TRUE FALSE] -> w277
                        frame False {
                        }
                        frame True {
                        }
                      }
                    }
                    "AMCS_Profile" <- w273
                  }
                  frame #3 {
                    # "convert time per range bin to meters\nand calculate smoothed bins using\nsmoothing range"
                    # "Plotting online cross section and smoothed online data"
                    # "Calculate the bin by bin mean of the data"
                    # "Collect 'Integration Period (Seconds)' number\nof scalar data"
                    # "Reading, processing, and plotting the online data"
                    n201 = local read "Data Reads (number of loops)"() -> (w307:i32)
                    n202 = for {
                      N: w307 -> [_]
                      tunnel: [w327] -> w319 mode=indexing
                      tunnel: [w328] -> w299 mode=indexing
                      # "Scalar Data is retrieved from Global \nVariable that scaler.vi is writing to,"
                      n203 = disable-structure shown="Disabled" {
                        frame Disabled {
                          n204 = global read "Scalar_Data.vi" "Scalar Data  3"() -> ()  [unwired: 1 out]
                          n205 = global read "Scalar_Data.vi" "Scalar Data"() -> ()  [unwired: 1 out]
                        }
                        frame Enabled {
                        }
                      }
                      n206 = global read "AMCS_Data.vi" "AMCS_Data"() -> (w331:u16[][])
                      n207 = Index Array(array=w331, index (row) #1=0 ("index (row)"), index (row) #2=2 ("index (row)")) -> (element #1=w327:u16[], element #2=w328:u16[])  [unwired: 2 in]
                    }
                    n208 = Transpose 2D Array(2D array=w319) -> (transposed array=w323:u16[][])
                    n209 = Transpose 2D Array(2D array=w299) -> (transposed array=w305:u16[][])
                    n210 = for {
                      tunnel: w323 -> [w333] mode=indexing
                      tunnel: [w332] -> w324 mode=indexing
                      n211 = call-poly <vilib>:"Mean.vi"("X"=w333) -> ("mean"=w332:dbl)  [unwired: 1 out]
                    }
                    n212 = for {
                      tunnel: w305 -> [w326] mode=indexing
                      tunnel: [w325] -> w306 mode=indexing
                      n213 = call-poly <vilib>:"Mean.vi"("X"=w326) -> ("mean"=w325:dbl)  [unwired: 1 out]
                    }
                    n214 = local read "bins"() -> (w298:u32)
                    n215 = Array Subset(array=w324, index=1 ("dimension size"), length=w298) -> (w311:dbl[])
                    n216 = Array Subset(array=w306, index=1 ("dimension size"), length=w298) -> (w303:dbl[])
                    n217 = local read "background length"() -> (w288:i32)
                    n218 = local read "background start"() -> (w289:u32)
                    n219 = Array Size(array=w311) -> (size(s)=w308:i32)
                    n220 = Array Size(array=w303) -> (size(s)=w300:i32)
                    n221 = Initialize Array(1.0 ("element"), w308) -> (w310:dbl[])
                    n222 = Initialize Array(1.0 ("element"), w300) -> (w302:dbl[])
                    n223 = Multiply(x=w311, y=w310) -> (x*y=w312:dbl[])
                    "On-Line Bin Readings" <- w312
                    n224 = Multiply(x=w303, y=w302) -> (x*y=w292:dbl[])
                    "On-Line Bin Readings 2" <- w292
                    n225 = local read "Total DIAL Integration Time (Minutes)"() -> (w315:i32)
                    n226 = local read "Time Resolution Per Bin(ns)"() -> (w284:u32)
                    n227 = Array Subset(array=w312, index=w289, length=w288) -> (w321:dbl[])
                    n228 = Array Subset(array=w292, index=w289, length=w288) -> (w294:dbl[])
                    n229 = call-poly <vilib>:"Mean.vi"("X"=w321) -> ("mean"=w320:dbl)  [unwired: 1 out]
                    n230 = call-poly <vilib>:"Mean.vi"("X"=w294) -> ("mean"=w295:dbl)  [unwired: 1 out]
                    n231 = Divide(x=w315, y=w307) -> (x/y=w313:dbl)
                    n232 = local read "Index"() -> (w293:i32)
                    n233 = Subtract(x=w312, y=w320) -> (x-y=w317:dbl[])
                    n234 = Subtract(x=w292, y=w295) -> (x-y=w296:dbl[])
                    n235 = To Double Precision Float(number=w284) -> (double precision float=w285:dbl)
                    n236 = Multiply(x=w313, y=60.0) -> (x*y=w290:dbl)
                    n237 = Multiply(x=w285, y=0.15) -> (x*y=w287:dbl)
                    n238 = call "Ring Buffer Online Far.vi"("Index"=w293, "Profiles to Average"=w290, "Input Array"=w317) -> ("AvgArray"=w316:dbl[])  [unwired: 7 in, 1 out]
                    n239 = call "Ring Buffer Online Near.vi"("Index"=w293, "Profiles to Average"=w290, "Input Array"=w296) -> ("AvgArray"=w297:dbl[])  [unwired: 7 in, 1 out]
                    n240 = Divide(x="Smoothing Range", y=w287) -> (x/y=w282:dbl)
                    "Smoothed Bins" <- w282
                    n241 = call "Smooth Arrray.vi"("smooth size"=w282, "Raw Array"=w316) -> ("Smoothed Array"=→"On-Line  Smoothed":dbl[])  [unwired: 9 in]
                    n242 = call "Smooth Arrray.vi"("smooth size"=w282, "Raw Array"=w297) -> ("Smoothed Array"=→"On-Line Smoothed 2":dbl[])  [unwired: 9 in]
                    n243 = disable-structure shown="Disabled" {
                      frame Disabled {
                        n244 = script code="format long;\ncounts=sum(Online);\nif counts >=0.5e6\ntime=time;\nelse\ntime=time\nend"() -> ()  [unwired: 3 in, 2 out]
                      }
                      frame Enabled {
                      }
                    }
                  }
                  frame #4 {
                    # "CODE REMOVED!!"
                    # "Toggling the Agiltron switch to the offline DBR seed laser"
                  }
                  frame #5 {
                    # "Save the recently collected online data if 'Save Data?' is true"
                    n245 = case shown="True" "Save Data?" {
                      frame False {
                        # "'Save Data?' is false, do nothing"
                      }
                      frame True {
                        # "'Save Data?' is true, save onfline data to the Data Disk"
                        # "Write only one copy of data at this time"
                        # "Retrieve Julian Date"
                        n246 = local read "Readings"() -> (w342:T5)
                        n247 = local read "Time Resolution Per Bin(ns)"() -> (w340:u32)
                        n248 = local read "Number of Accumulates"() -> (w338:u32)
                        n249 = local read "Number of Bins"() -> (w339:u32)
                        n250 = local write "DataOpen"(TRUE ("DataOpen")) -> ()
                        n251 = local read "Lambda On Read (nm)"() -> (w364:dbl)
                        n252 = local read "On-Line Bin Readings 2"() -> (w362:dbl[])
                        n253 = local read "On-Line Bin Readings"() -> (w366:dbl[])
                        n254 = local read "Average Diode Power"() -> (w363:dbl)
                        n255 = Unbundle By Name(w342) -> ("OnLineLD"=w341:dbl)
                        n256 = To Double Precision Float(number=w340) -> (double precision float=w337:dbl)
                        n257 = To Double Precision Float(number=w339) -> (double precision float=w336:dbl)
                        n258 = To Double Precision Float(number=w338) -> (double precision float=w335:dbl)
                        n259 = call "Julian_Date_2.vi"() -> ("Julian Date"=w365:dbl)  [unwired: 11 in]
                        n260 = Build Array (concatenate)(w365, w364, w341, w363, w337, w336, w335, w366) -> (w357:dbl[])
                        n261 = Build Array (concatenate)(w365, w364, w341, w363, w337, w336, w335, w362) -> (w347:dbl[])
                        n262 = local read "NF_On_Ref"() -> (w345:refnum<file>)
                        n263 = local read "FF_On_Ref"() -> (w361:refnum<file>)
                        n264 = local read "NF_On_Ptr"() -> (w346:i64)
                        n265 = local read "FF_On_Ptr"() -> (w360:i64)
                        n266 = Set File Position(offset (in bytes) (0)=w360, refnum=w361) -> (refnum out=w358:refnum<file>, error out=w355:errorcluster)  [unwired: 2 in]
                        n267 = Set File Position(offset (in bytes) (0)=w346, refnum=w345) -> (refnum out=w351:refnum<file>, error out=w349:errorcluster)  [unwired: 2 in]
                        n268 = Write to Binary File(file (use dialog)=w351, data=w347, error in=w349, 5:FALSE ("prepend array or string size? (T)")) -> (refnum out=w350:refnum<file>, error out=w348:errorcluster)  [unwired: 2 in, 1 out]
                        n269 = Write to Binary File(file (use dialog)=w358, data=w357, error in=w355, 5:FALSE ("prepend array or string size? (T)")) -> (refnum out=w356:refnum<file>, error out=w354:errorcluster)  [unwired: 2 in, 1 out]
                        n270 = Get File Position(4:w348, 7:w350) -> (2:w344:i64)  [unwired: 2 out]
                        n271 = Get File Position(4:w354, 7:w356) -> (2:w353:i64)  [unwired: 2 out]
                        n272 = local write "NF_On_Ptr"(w344) -> ()
                        n273 = local write "FF_On_Ptr"(w353) -> ()
                      }
                    }
                  }
                }
              }
              frame #3 {
                # "Frame 3: Read offline data, calculate aerosol data, and plot offline and normalized relative backscatter\nFrame 4: Swich to online DBR\nFrame 5: Save the offline data and related information"
                # "Frame 0: Read the offline wavelength and lock if necessary, though code is not finished to do so\nFrame 1: Read the output power from the Newport power meter\nFrame 2: Wait 'Scalar Wait Time' for buffers to clear of online contiminated data"
                # "offline"
                n274 = stacked-sequence {
                  frame #0 {
                    # "Every 60 data collection cycles, read the offline DBR wavelength, and if outside of wavelength tolerance, adjust DBR current until within tolerance"
                    n275 = local read "L_Count"() -> (w368:i32)
                    n276 = Quotient & Remainder(x=w368, y=60.0) -> (x-y*floor(x/y)=w369:dbl)  [unwired: 1 out]
                    n277 = Equal To 0?(x=w369) -> (x = 0?=w367:bool)
                    n278 = case shown="True" w367 {
                      frame False {
                      }
                      frame True {
                        n279 = while {
                          i -> [w374]
                          stop <- w372 stop-if-true
                          # "Frame 5 Increment ofline DBR current if below tolerance\nFrame 6: update ILX settings to front pannel"
                          # "Frame 3: Calculating the wavelength difference\nFrame 4:Decrement offline DBR current if above tolerance"
                          # "Frame 0: Read the offline laser wavelength (settle if t=0)"
                          n280 = stacked-sequence {
                            tunnel: w374 -> [w376 _ _ _ _]
                            tunnel: [_ _ w386 _ _] -> w373
                            frame #0 {
                              n281 = Equal To 0?(x=w376) -> (x = 0?=w375:bool)
                              n282 = case shown="True" w375 {
                                frame False {
                                }
                                frame True {
                                w377 = TRUE ("Boolean")
                                # "SWITCH to NON-ABSORBING and wait to settle"
                                n283 = Build Array(w377) -> (w382:bool[])
                                n284 = local write "WM Switch"(w377) -> ()
                                n285 = call-poly <vilib>:"DAQmx Write.vi"("task/channels in"=refnum<k21> "BristolWM", "data"=w382) -> ()  [unwired: 11 in, 3 out]
                                n286 = call "TL_Driver.vi"("Device In"=refnum<visa-resource-name> "ThorLabs", "Commands"=T9."Read_Status") -> ("Readings"=w380:T5)  [unwired: 10 in, 3 out]
                                n287 = local write "Readings"(w380) -> ()
                                n288 = Wait (ms)(milliseconds to wait=u32 3200) -> ()  [unwired: 1 out]
                                }
                              }
                            }
                            frame #1 {
                              # "Read Bristol WM"
                              n289 = local read "Bristol Out"() -> (w384:i32)
                              n290 = dll-call lib="C:/H2O_DIAL/LabVIEW-2012/Bristol WM V2_31b/CLDevIface.dll" fn="CLGetLambdaReading"("devHandle"=w384) -> ("return type"=→"Lambda Off Read (nm)":dbl)  [unwired: 4 in, 2 out]
                            }
                            frame #2 {
                              # "Once locked, stop looping and illuminate 'Wavelength Lock Offline'"
                              # "While loop continues locking process until the wavelength is within tolerance"
                              # "Calculating the difference between the actual and desired \noffline wavelength"
                              n291 = local read "Lambda Off Read (nm)"() -> (w394:dbl)
                              n292 = Subtract(x=w394, y="Lambda Off Set (nm)") -> (x-y=w387:dbl)
                              "WL Difference off" <- w387
                              n293 = local read "Offline_Tol"() -> (w391:dbl)
                              n294 = Multiply(x=-1.0, y=w391) -> (x*y=w392:dbl)
                              n295 = Greater?(x=w387, y=w392) -> (0:w388:bool)
                              n296 = Less?(x=w387, y=w391) -> (x < y?=w389:bool)
                              n297 = And(x=w388, y=w389) -> (x .and. y?=w386:bool)
                              "Wavelength Lock Offline" <- w386
                              n298 = case shown="True" w386 {
                                frame False {
                                }
                                frame True {
                                w395 = FALSE ("Boolean")
                                # "SWITCH back to ABSORBING and wait to settle"
                                n299 = Build Array(w395) -> (w397:bool[])
                                n300 = local write "WM Switch"(w395) -> ()
                                n301 = call-poly <vilib>:"DAQmx Write.vi"("task/channels in"=refnum<k21> "BristolWM", "data"=w397) -> ()  [unwired: 11 in, 3 out]
                                n302 = Wait (ms)(milliseconds to wait=u32 3200) -> ()  [unwired: 1 out]
                                }
                              }
                            }
                            frame #3 {
                              # "Would adjust the offline wavelength if code was finished"
                              n303 = local read "WL Difference off"() -> (w401:dbl)
                              n304 = Greater Or Equal?(x=w401, y="Offline_Tol") -> (x >= y?=w399:bool)
                              n305 = case shown="True" w399 {
                                frame False {
                                # "WL difference is not out of range, do nothing"
                                }
                                frame True {
                                # "Generating a command string\nto decrement the current"
                                # "WL difference is greater than 0.0002 nm,\ndecrement the DBR current by 0.01 mA"
                                # "WL difference is out of range, this is where you would decrement\nthe laser current"
                                n306 = local read "Settings"() -> (w406:T6)
                                n307 = Unbundle By Name(w406) -> ("OffLineTEC"=w407:dbl)
                                n308 = Subtract(x=w407, y=0.00012) -> (x-y=w408:dbl)
                                n309 = Bundle By Name(cluster=w406, "OffLineTEC"=w408, "Module"=T11."Off Line TEC") -> (w405:T6)
                                n310 = call "TL_Driver.vi"("Device In"=refnum<visa-resource-name> "ThorLabs", "Commands"=T9."SET", "Settings"=w405) -> ("Readings"=w402:T5)  [unwired: 9 in, 3 out]
                                n311 = local write "Settings"(w405) -> ()
                                n312 = local write "Readings"(w402) -> ()
                                }
                              }
                            }
                            frame #4 {
                              # "This is where you would increment the offline current if below tolerance"
                              n313 = local read "Offline_Tol"() -> (w412:dbl)
                              n314 = local read "WL Difference off"() -> (w415:dbl)
                              n315 = Multiply(x=-1.0, y=w412) -> (x*y=w411:dbl)
                              n316 = Less Or Equal?(x=w415, y=w411) -> (x <= y?=w414:bool)
                              n317 = case shown="True" w414 {
                                frame False {
                                # "WL difference is not outisde tolerance, do nothing"
                                }
                                frame True {
                                # "Generating a command string\nto decrement the current"
                                # "WL difference is less than 0.0002 nm,\nincrement the DBR current by 0.01 mA"
                                # "Incrementing the current if below tolerance"
                                n318 = local read "Settings"() -> (w419:T6)
                                n319 = Unbundle By Name(w419) -> ("OffLineTEC"=w421:dbl)
                                n320 = Add(x=w421, y=0.00012) -> (x+y=w422:dbl)
                                n321 = Bundle By Name(cluster=w419, "OffLineTEC"=w422, "Module"=T11."Off Line TEC") -> (w420:T6)
                                n322 = call "TL_Driver.vi"("Device In"=refnum<visa-resource-name> "ThorLabs", "Commands"=T9."SET", "Settings"=w420) -> ("Readings"=w416:T5)  [unwired: 9 in, 3 out]
                                n323 = local write "Settings"(w420) -> ()
                                n324 = local write "Readings"(w416) -> ()
                                }
                              }
                            }
                          }
                          n325 = Or(x=w373, y="Cancel Offline") -> (x .or. y?=w372:bool)
                        }
                      }
                    }
                  }
                  frame #1 {
                    # "CODE REMOVED!!!"
                    # "Reading the output power of the laser transmitter from the Ophir power meter, once read, convert to corresponding pulse energy and plot"
                  }
                  frame #2 {
                    # "Added in the ability to interactively control the ThorLab  setting (just etalon temp for now)"
                    # "CODE REMOVED!!!"
                    # "Wait 'Scalar Wait Time' for buffers to clear of online contiminated offline data"
                    n326 = event shown="[3] \"Settings.OffLineLD\": Value Change" {
                      selector: _ -> [_ _ _ _]
                      dyn-events: _ -> [_ _ _ _]
                      timeout: 1 -> [_ _ _ _]
                      event Timeout {
                        n327 = event-data() -> ()  [unwired: 1 in, 2 out]
                      }
                      event "Settings.EtalonTEC": Value Change {
                        # "Generating a command string\nto update the etalon"
                        n328 = event-data() -> ()  [unwired: 1 in, 5 out]
                        n329 = local read "Settings"() -> (w430:T6)
                        n330 = Unbundle By Name(w430) -> ("EtalonTEC"=w429:dbl)
                        n331 = Bundle By Name(cluster=w430, "EtalonTEC"=w429, "Module"=T11."Etalon TEC") -> (w432:T6)
                        n332 = call "TL_Driver.vi"("Device In"=refnum<visa-resource-name> "ThorLabs", "Commands"=T9."SET", "Settings"=w432) -> ("Readings"=w431:T5)  [unwired: 9 in, 3 out]
                        n333 = local write "Settings"(w432) -> ()
                        n334 = local write "Readings"(w431) -> ()
                      }
                      event "Settings.OnLineLD": Value Change {
                        # "Generating a command string\nto update the Online LD"
                        n335 = event-data() -> ()  [unwired: 1 in, 5 out]
                        n336 = local read "Settings"() -> (w437:T6)
                        n337 = Unbundle By Name(w437) -> ("OnLineLD"=w436:dbl)
                        n338 = Bundle By Name(cluster=w437, "OnLineLD"=w436, "Module"=T11."On Line LD") -> (w439:T6)
                        n339 = call "TL_Driver.vi"("Device In"=refnum<visa-resource-name> "ThorLabs", "Commands"=T9."SET", "Settings"=w439) -> ("Readings"=w438:T5)  [unwired: 9 in, 3 out]
                        n340 = local write "Settings"(w439) -> ()
                        n341 = local write "Readings"(w438) -> ()
                      }
                      event "Settings.OffLineLD": Value Change {
                        # "Generating a command string\nto update the Offline LD"
                        n342 = event-data() -> ()  [unwired: 1 in, 5 out]
                        n343 = local read "Settings"() -> (w444:T6)
                        n344 = Unbundle By Name(w444) -> ("OffLineLD"=w443:dbl)
                        n345 = Bundle By Name(cluster=w444, "OffLineLD"=w443, "Module"=T11."Off Line LD") -> (w446:T6)
                        n346 = call "TL_Driver.vi"("Device In"=refnum<visa-resource-name> "ThorLabs", "Commands"=T9."SET", "Settings"=w446) -> ("Readings"=w445:T5)  [unwired: 9 in, 3 out]
                        n347 = local write "Settings"(w446) -> ()
                        n348 = local write "Readings"(w445) -> ()
                      }
                    }
                  }
                  frame #3 {
                    w480 = 1 ("dimension size")
                    w483 = 1
                    # "Plotting the normalized relative \nbackscatter"
                    # "Calculating the normalized relative backscatter"
                    # "Calculating/Plotting smoothed data,\ncross sections etc."
                    # "Pick off data with\nout header"
                    # "Calculate mean bin by bin mean"
                    # "Reading in 'Integration Period (Seconds)' of data"
                    # "Read the offline data from the scalar card, perform smoothing, calculate normalized relative backscatter, and plot"
                    # "File path in MATLAB script is of old dial is:\nF:\\Micropulse DIAL\\Micropulse DIAL Matlab\\\nFinal Overlap Function.mat')];"
                    # "Collects Data From Card,\nSends It To The Chart,\nAnd Saves A Copy As A\nFile If Option Selected On\nFront Panel"
                    n349 = for {
                      N: "Data Reads (number of loops)" -> [_]
                      tunnel: [w516] -> w513 mode=indexing
                      tunnel: [w515] -> w495 mode=indexing
                      # "Read in latest scalar card data from \n'Scalar Data' global variable that \nscaler.vi is writing to, then wait 1 sec\nfor next batch of data"
                      n350 = global read "AMCS_Data.vi" "AMCS_Data"() -> (w517:u16[][])
                      n351 = disable-structure shown="Disabled" {
                        frame Disabled {
                          n352 = global read "Scalar_Data.vi" "Scalar Data  2"() -> ()  [unwired: 1 out]
                          n353 = global read "Scalar_Data.vi" "Scalar Data  4"() -> ()  [unwired: 1 out]
                        }
                        frame Enabled {
                        }
                      }
                      n354 = Index Array(array=w517, index (row) #1=1 ("index (row)"), index (row) #2=3 ("index (row)")) -> (element #1=w516:u16[], element #2=w515:u16[])  [unwired: 2 in]
                    }
                    n355 = local read "Total DIAL Integration Time (Minutes)"() -> (w504:i32)
                    n356 = Divide(x=w504, y="Data Reads (number of loops)") -> (x/y=w502:dbl)
                    n357 = local read "Total Aerosol Integration Time (Minutes)"() -> (w506:dbl)
                    n358 = Multiply(x=w502, y=60.0) -> (x*y=w488:dbl)
                    n359 = local read "background length"() -> (w452:i32)
                    n360 = local read "background start"() -> (w453:u32)
                    n361 = Transpose 2D Array(2D array=w513) -> (transposed array=w512:u16[][])
                    n362 = Transpose 2D Array(2D array=w495) -> (transposed array=w494:u16[][])
                    n363 = Divide(x=w506, y="Data Reads (number of loops)") -> (x/y=w507:dbl)
                    n364 = for {
                      tunnel: w512 -> [w523] mode=indexing
                      tunnel: [w522] -> w514 mode=indexing
                      tunnel: w494 -> [w521] mode=indexing
                      tunnel: [w520] -> _ mode=indexing
                      tunnel: [w520] -> w491 mode=indexing
                      n365 = call-poly <vilib>:"Mean.vi"("X"=w523) -> ("mean"=w522:dbl)  [unwired: 1 out]
                      n366 = call-poly <vilib>:"Mean.vi"("X"=w521) -> ("mean"=w520:dbl)  [unwired: 1 out]
                    }
                    n367 = local read "bins"() -> (w481:u32)
                    n368 = Multiply(x=w507, y=60.0) -> (x*y=w471:dbl)
                    n369 = Array Subset(array=w491, index=w480, length=w481) -> (w492:dbl[])
                    "Off-Line Bin Readings 2" <- w492
                    n370 = Array Subset(array=w514, index=w480, length=w481) -> (w490:dbl[])
                    "Off-Line  Bin Readings" <- w490
                    n371 = Array Subset(array=w492, index=w453, length=w452) -> (w493:dbl[])
                    n372 = Array Subset(array=w490, index=w453, length=w452) -> (w511:dbl[])
                    n373 = local read "Smoothed Bins"() -> (w449:dbl)
                    n374 = call-poly <vilib>:"Mean.vi"("X"=w493) -> ("mean"=w459:dbl)  [unwired: 1 out]
                    n375 = call-poly <vilib>:"Mean.vi"("X"=w511) -> ("mean"=w460:dbl)  [unwired: 1 out]
                    n376 = local read "Index"() -> (w470:i32)
                    n377 = Subtract(x=w492, y=w459) -> (x-y=w472:dbl[])
                    n378 = Subtract(x=w490, y=w460) -> (x-y=w486:dbl[])
                    n379 = call "Ring Buffer Offline Far.vi"("Index"=w470, "Profiles to Average"=w488, "Input Array"=w486) -> ("AvgArray"=w509:dbl[], "RingBufferOut"=→"RingBuffer offline far":dbl[][])  [unwired: 7 in]
                    n380 = call "Ring Buffer Aerosol Far.vi"("Index"=w470, "Profiles to Average"=w471, "Input Array"=w486) -> ("AvgArray"=w505:dbl[], "RingBufferOut"=→"RingBuffer aerosol far":dbl[][])  [unwired: 7 in]
                    n381 = call "Ring Buffer Offline Near.vi"("Index"=w470, "Profiles to Average"=w488, "Input Array"=w472) -> ("AvgArray"=w489:dbl[], "RingBufferOut"=→"RingBuffer offline near":dbl[][])  [unwired: 7 in]
                    n382 = call "Ring Buffer Aerosol Near.vi"("Index"=w470, "Profiles to Average"=w471, "Input Array"=w472) -> ("AvgArray"=w468:dbl[], "RingBufferOut"=→"RingBuffer aerosol near":dbl[][])  [unwired: 7 in]
                    n383 = Reshape Array(w486, w480, w481) -> (→"raw counts":dbl[][])
                    n384 = Reshape Array(w472, w480, w481) -> (→"raw counts near":dbl[][])
                    n385 = call "Smooth Arrray.vi"("smooth size"=w449, "Raw Array"=w509) -> ("Smoothed Array"=→"Off-Line Smoothed":dbl[])  [unwired: 9 in]
                    n386 = call "Smooth Arrray.vi"("smooth size"=w449, "Raw Array"=w505) -> ("Smoothed Array"=w479:dbl[])  [unwired: 9 in]
                    "Aerosol Smoothed" <- w479
                    n387 = call "Smooth Arrray.vi"("smooth size"=w449, "Raw Array"=w489) -> ("Smoothed Array"=→"Off-Line Smoothed 2":dbl[])  [unwired: 9 in]
                    n388 = call "Smooth Arrray.vi"("smooth size"=w449, "Raw Array"=w468) -> ("Smoothed Array"=w451:dbl[])  [unwired: 9 in]
                    "Aerosol Smoothed 2" <- w451
                    n389 = local read "Number of Accumulates"() -> (w455:u32)
                    n390 = local read "Temperature (C)"() -> (w501:dbl)
                    n391 = local read "Pressure (mb)"() -> (w500:dbl)
                    n392 = script code="%accum_num=10000;     % scaler card setting number of accumulations\nt_bin = 500e-9                 % scaler card setting time per bin\n%t_d = 37.3e-9;                % APD dead time from spec sheet\n\n% conversion from accumulated counts to count rate  (c/s)\nc_convert = 1./t_bin./accum_num;\nCR_far = p_raw_far.*c_convert;\nCR_near = p_raw_near.*c_convert;\nCR_total_far = (p_raw_far+b_far).*c_convert;\nCR_total_near = (p_raw_near+b_near).*c_convert;\nb_CR_far =b_far.*c_convert;\nb_CR_near =b_near.*c_convert;\n\n% create a range array\nsize_p =  size(p_raw_far,2);\nr = (75:75:size_p*75)./1e3; \n    \n%APD correction factor\n D_far = 1./(1-(t_d*CR_total_far));\n D_near = 1./(1-(t_d*CR_total_near));\n\n %Calculating normalize relative backscatter profile\n nrb_far = CR_far.*D_far.*r.^2.*1e-6;\n nrb_near = CR_near.*D_near.*r.^2.*1e-6;"("E"=6.0 ("Real"), "temp"=w501, "press"=w500, "p_raw_far"=w479, "b_far"=w460, "b_near"=w459, "p_raw_near"=w451, "accum_num"=w455, "t_d"="dead time") -> ("nrb_far"=w474:cdb[], "D_far"=w465:dbl[], "nrb_near"=w473:cdb[], "D_near"=w464:dbl[], "b_CR_far"=w457:dbl, "b_CR_near"=w456:dbl)  [unwired: 1 in, 1 out]
                    n393 = local read "bins"() -> (w482:u32)
                    n394 = local read "Altitude Array (km)"() -> (w476:dbl[])
                    n395 = Bundle(w457, w456) -> (→"?":cluster{dbl, dbl})  [unwired: 1 in]
                    n396 = Build Array(w474, w473) -> (w478:cdb[][])
                    n397 = Build Array(w465, w464) -> (w463:dbl[][])
                    n398 = Reshape Array(w473, w483, w482) -> (→"NRB 2":cdb[][])
                    n399 = Reshape Array(w474, w483, w482) -> (→"NRB":cdb[][])
                    n400 = Build Array(w476, w476) -> (w475:dbl[][])
                    n401 = call "Convert to Dynamic Data7"("2D Array"=w463) -> ("Dynamic Data Type"=w462:dynamicdata)  [unwired: 3 in]
                    n402 = call "Convert to Dynamic Data3"("2D Array"=w478) -> ("Dynamic Data Type"=w477:dynamicdata)  [unwired: 3 in]
                    n403 = call "Convert to Dynamic Data4"("2D Array"=w475) -> ("Dynamic Data Type"=w466:dynamicdata)  [unwired: 3 in]
                    n404 = call "Build XY Graph2"("Y Input"=w466, "X Input"=w477) -> ("XY Graph"=→"NRB plot":cluster{"Y":dbl[], "Y":dbl[]}[])  [unwired: 3 in, 6 out]
                    n405 = call "Build XY Graph4"("Y Input"=w466, "X Input"=w462) -> ("XY Graph"=→"Correction":cluster{"Y":dbl[], "Y":dbl[]}[])  [unwired: 3 in, 6 out]
                  }
                  frame #4 {
                    # "CODE REMOVED!!!"
                    # "Toggle Agiltron switch to online DBR"
                  }
                  frame #5 {
                    # "If 'Save Data?' is true, save all relavant offline info"
                    n406 = local read "Save Data?"() -> (w524:bool)
                    n407 = case shown="True" w524 {
                      frame False {
                        # "'Save Data?' is false, do nothing"
                      }
                      frame True {
                        # "Write only one data file at this time"
                        # "Retrive Julian Date"
                        # "'Save Data?' is true, save offline data to the Data Disk"
                        n408 = local read "Readings"() -> (w526:T5)
                        n409 = local read "Off-Line Bin Readings 2"() -> (w545:dbl[])
                        n410 = local read "Lambda Off Read (nm)"() -> (w547:dbl)
                        n411 = local read "Off-Line  Bin Readings"() -> (w552:dbl[])
                        n412 = local read "Relative Humdity (%)"() -> (w551:dbl)
                        n413 = local read "Temperature (C)"() -> (w549:dbl)
                        n414 = Unbundle By Name(w526) -> ("OffLineLD"=w525:dbl)
                        n415 = local read "T_bench"() -> (w548:sgl)
                        n416 = local read "Pressure (mb)"() -> (w550:dbl)
                        n417 = call "Julian_Date_2.vi"() -> ("Julian Date"=w546:dbl)  [unwired: 11 in]
                        n418 = Build Array (concatenate)(w546, w547, w525, w548, w549, w550, w551, w552) -> (w531:dbl[])
                        n419 = Build Array (concatenate)(w546, w547, w525, w548, w549, w550, w551, w545) -> (w528:dbl[])
                        n420 = local read "FF_Off_Ref"() -> (w533:refnum<file>)
                        n421 = local read "NF_Off_Ref"() -> (w530:refnum<file>)
                        n422 = local read "FF_Off_Ptr"() -> (w532:i64)
                        n423 = local read "NF_Off_Ptr"() -> (w529:i64)
                        n424 = Set File Position(offset (in bytes) (0)=w532, refnum=w533) -> (refnum out=w544:refnum<file>, error out=w542:errorcluster)  [unwired: 2 in]
                        n425 = Set File Position(offset (in bytes) (0)=w529, refnum=w530) -> (refnum out=w540:refnum<file>, error out=w538:errorcluster)  [unwired: 2 in]
                        n426 = Write to Binary File(file (use dialog)=w544, data=w531, error in=w542, 5:FALSE ("prepend array or string size? (T)")) -> (refnum out=w543:refnum<file>, error out=w541:errorcluster)  [unwired: 2 in, 1 out]
                        n427 = Write to Binary File(file (use dialog)=w540, data=w528, error in=w538, 5:FALSE ("prepend array or string size? (T)")) -> (refnum out=w539:refnum<file>, error out=w537:errorcluster)  [unwired: 2 in, 1 out]
                        n428 = Get File Position(4:w541, 7:w543) -> (2:w534:i64)  [unwired: 2 out]
                        n429 = Get File Position(4:w537, 7:w539) -> (2:w527:i64)  [unwired: 2 out]
                        n430 = local write "FF_Off_Ptr"(w534) -> ()
                        n431 = local write "NF_Off_Ptr"(w527) -> ()
                      }
                    }
                  }
                }
              }
              frame #4 {
                n432 = First Call?() -> (First Call?: T/F=w555:bool)
                n433 = Or(x="calculate absorption cross sections", y=w555) -> (x .or. y?=w553:bool)
                n434 = case shown="True" w553 {
                  frame False {
                  }
                  frame True {
                    # "calculate absorption cross sections from HITRAN data base"
                    n435 = local read "Off-Line Smoothed"() -> (w556:dbl[])
                    n436 = local read "Lambda On Read (nm)"() -> (w559:dbl)
                    n437 = local read "Lambda Off Set (nm)"() -> (w562:dbl)
                    n438 = local read "Temperature (C)"() -> (w560:dbl)
                    n439 = local read "Pressure (mb)"() -> (w561:dbl)
                    n440 = script code="hitran = dlmread('C:\\H2O_DIAL\\LabVIEW-2012\\Micropulse DIAL Matlab\\815nm_841nm_HITRAN_2008.csv', ',',[1 1 1676 8]);\n%hitran = dlmread('C:\\H2O_DIAL\\LabVIEW-2012\\Micropulse DIAL Matlab\\824nm_841nm_H2O_Spectral_Calc.csv', ',',[1 1 1209 7]);\n\n\n\n%Range vector in meters\nrange = ([75:75:size(Online,2)*75]);\n\nif lambda< 828\nlambda=828.195;\nelse\nlambda=lambda;\nend;\n\n%%\n\n%Voigt profile calculation\nWNmin = 1/(828+4)*1e7;  % 832.0 nm converted to wavenumber\nWNmax = 1/(828-4)*1e7;  % 824.0 nm converted to wavenumber\n\n%Find lines from WNmin to WNmax to calculate voigt profile\nline_indices = hitran(1:size(hitran,1),1)>WNmin & hitran(1:size(hitran,1),1)<WNmax;\n\nline = double(hitran(line_indices, 1:size(hitran,2)));\n\n%Calculate temperature and pressure profile\nT0 = 273+25; % surface temperature\nT0 = 273+T0_C;\nT = T0-0.0065.*range; % set to match the sounding\n\n% pressure in atmospheres\nP0  = 0.83; % surface pressure\nP0  = P0_mb/1000*0.986; %pressure in mb converted to atm\nP = P0.*(T0./T).^-5.5;   % set this value to match sounding\n\nT00 = 296;              % HITRAN reference temperature [K]\nP00 = 1;                % HITRAN reference pressure [atm]\nnu0_0 = line(:,1);      % absorption line center wavenumber from HITRAN [cm^-1]\nS0 = line(:,2);         % initial linestrength from HITRAN [cm^-1/(mol*cm^-2)]   \ngammal0 = line(:,4);    % air-broadened halfwidth at T_ref and P_ref from HITRAN [cm^-1/atm]\ngamma_s = line(:,5);    % self-broadened halfwidth at T_ref and P_ref from HITRAN [cm^-1/atm]\nE = line(:,6);          % ground state transition energy from HITRAN [cm^-1]  \nalpha = line(:,7);      % linewidth temperature dependence factor from HITRAN\ndelta = line(:,8);      % pressure shift from HiTRAN [cm^-1 atm^-1]\n\nnu_on = 1/(lambda)*1e7;\nnu_off = 1/(lambda_off)*1e7;\n\nfor i = 1:size(Online,2); % calculate the absorption cross section at each range\n  \n    nu0 = nu0_0+delta.*(P(i)./P00); % unclear if it should be Pi/P00  \n    gammal = gammal0.*(P(i)./P00).*((T00./T(i)).^alpha);    %Calculate Lorentz lineweidth at P(i) and T(i)\n\n    const.m = 18.015E-3./6.022E23; % mass of a single water molecule\n    const.k_B = 1.3806488e-23; % (J/K)\n    const.c = 299792458; % (m/s) (exact)\n \n    gammad = (nu0).*((2.0.*const.k_B.*T(i).*log(2.0))./(const.m.*const.c^2)).^(0.5);  %Calculate HWHM Doppler linewidth at T(i)\n     \n    % term 1 in the Voigt profile\n    y = (gammal./gammad).*((log(2.0)).^(0.5));\n    \n    % term 2 in the Voigt profile\n    x_on = ((nu_on-nu0)./gammad).*(log(2.0)).^(0.5);\n    x_off = ((nu_off-nu0)./gammad).*(log(2.0)).^(0.5);\n    \n    %setting up Voigt convolution\n    t = (-(size(line,1))/2:1:size(line,1)/2-1); %set up the integration spectral step size\n    t = repmat(t',1,length(x_on))';\n    x_on = repmat(x_on,1,length(t));\n    x_off = repmat(x_off,1,length(t));\n    y = repmat(y,1,length(t));\n    f_on = (exp(-t.^2.0))./(y.^2.0+(x_on-t).^2.0);  % combined Voigt term 1 and 2\n    f_off = (exp(-t.^2.0))./(y.^2.0+(x_off-t).^2.0);\n    %Voigt integration over all of the lines at the on and offline locations\n    z_on = trapz(t(1,:),f_on,2);\n    z_off =  trapz(t(1,:),f_off,2);\n    integral_on = z_on;\n    integral_off = z_off;\n    %Calculate linestrength at temperature T\n    S = S0.*((T00./T(i)).^(1.5)).*exp(1.439.*E.*((1./T00)-(1./T(i))));\n \n    %Calculate the Voigt profile\n    K_on = (y(:,1)./pi).*integral_on;\n    K_off = (y(:,1)./pi).*integral_off;\n    \n    %Calculate the Voigt profile absorption cross section [cm^2]\n    sigmav_on = S.*(1./gammad).*(((log(2.0))./pi).^(0.5)).*K_on; %.*far_wing_on;\n    sigmav_off = S.*(1./gammad).*(((log(2.0))./pi).^(0.5)).*K_off; %.*far_wing_off;\n    \n    %Sum contributions from all of the surrounding lines\n    sigma_on_total(i) = sum(sigmav_on);\n    sigma_off_total(i) = sum(sigmav_off);\n    \nend;"("lambda"=w559, "lambda_off"=w562, "P0_mb"=w561, "T0_C"=w560, "Online"=w556) -> ("sigma_on_total"=→"sigma_on_total":dbl[], "sigma_off_total"=→"sigma_off_total":dbl[])  [unwired: 1 in, 1 out]
                  }
                }
              }
              frame #5 {
                w573 = 1
                # "normalization factor\nfrom 300 to 450m"
                # "OPTICAL DEPTH PLOT"
                # "new rainbow color bar display"
                # "Data Processing Far Channel"
                # "new rainbow color bar display"
                # "Calculating the range resolved water vapor number density and plotting"
                n441 = local read "sigma_off_total"() -> (w596:dbl[])
                n442 = local read "sigma_on_total"() -> (w593:dbl[])
                n443 = local read "On-Line  Smoothed"() -> (w571:dbl[])
                n444 = local read "Off-Line Smoothed"() -> (w570:dbl[])
                n445 = local read "Off-Line Smoothed 2"() -> (w594:dbl[])
                n446 = local read "On-Line Smoothed 2"() -> (w595:dbl[])
                n447 = script code="%Time averaging in seconds.  180 Seconds =3 minutes\ntemporal_average = 180;\n\n%Spatial averaging in bins.  2 bins = 150 meters\nspatial_average = 2;\n\n%Creating r and r+deltar vectors..this can also be acsomplished using the\n%diff command\np_oni = Online(:,1:size(Online,2)-1);\n\np_onii = Online(:,2:size(Online,2));\n\np_offi = Offline(:,1:size(Offline,2)-1);\n\np_offii = Offline(:,2:size(Offline,2));\n\nInside = (p_oni.*p_offii)./(p_onii.*p_offi);\n\ndel_cross = 1./(2.*(sigma_on_total(1:size(Online,2)-1)-sigma_off_total(1:size(Offline,2)-1)).*75*100);\n\ndel_cross(isinf(del_cross)) = 0;\n\n%Calculating Number density\nN = del_cross.*log(Inside);\n\n%Spatial smoothing of the profiles\nfilter1 = ones(1,2)./2;\n\nN_1 = N;\n\nN_1_avg = filter2(filter1,N_1);\n\nfilter1 = ones(1,10)./10;\n\nN_2 = N;\n\nN_2_avg = filter2(filter1,N_2);\n\nN_new = zeros(size(N,1),size(N,2));\n \n%Using different averaging windows for different altitudes \nN_avg=[N_1_avg(:,1:40)';N_2_avg(:,41:size(N,2))']';\n\n\nw = N_avg.*1e6.*18.015./6.022e23"("Online"=w595, "Offline"=w594, "sigma_on_total"=w593, "sigma_off_total"=w596) -> ("N_avg"=w597:cdb[], "w"=w606:cdb[])  [unwired: 1 in, 1 out]
                n448 = script code="%Time averaging in seconds.  180 Seconds = 3 minutes\ntemporal_average = 180;\n\n%Spatial averaging in bins.  2 bins = 150 meters\nspatial_average = 2;\n\n%Creating r and r+deltar vectors..this can also be acsomplished using the\n%diff command\np_oni = Online(:,1:size(Online,2)-1);\n\np_onii = Online(:,2:size(Online,2));\n\np_offi = Offline(:,1:size(Offline,2)-1);\n\np_offii = Offline(:,2:size(Offline,2));\n\nInside = (p_oni.*p_offii)./(p_onii.*p_offi);\n\ndel_cross = 1./(2.*(sigma_on_total(1:size(Online,2)-1)-sigma_off_total(1:size(Offline,2)-1)).*75*100);\n\ndel_cross(isinf(del_cross)) = 0;\n\n%Calculating Number density\nN = del_cross.*log(Inside);\n\n%Spatial smoothing of the profiles\nfilter1 = ones(1,2)./2;\n\nN_1 = N;\n\nN_1_avg = filter2(filter1,N_1);\n\nfilter1 = ones(1,10)./10;\n\nN_2 = N;\n\nN_2_avg = filter2(filter1,N_2);\n\nN_new = zeros(size(N,1),size(N,2));\n \n%Using different averaging windows for different altitudes \nN_avg=[N_1_avg(:,1:40)';N_2_avg(:,41:size(N,2))']';\n\n \nw = N_avg.*1e6.*18.015./6.022e23"("Online"=w571, "Offline"=w570, "sigma_on_total"=w593, "sigma_off_total"=w596) -> ("N_avg"=w602:cdb[], "w"=w603:cdb[])  [unwired: 1 in, 1 out]
                n449 = local read "Time Resolution Per Bin(ns)"() -> (w572:u32)
                n450 = local read "bins"() -> (w598:u32)
                n451 = local read "Altitude Array (km)"() -> (w568:dbl[])
                n452 = Build Array(w603, w606) -> (w609:cdb[][])
                n453 = To Double Precision Float(number=w572) -> (double precision float=w591:dbl)
                n454 = Reshape Array(w602, w573, w598) -> (w613:cdb[][])
                n455 = Reshape Array(w597, w573, w598) -> (w600:cdb[][])
                n456 = Multiply(x=0.15, y=w591) -> (x*y=w589:dbl)
                n457 = Build Array(w602, w597) -> (w607:cdb[][])
                n458 = Divide(x=300.0, y=w589) -> (x/y=w586:dbl)
                n459 = Divide(x=450.0, y=w589) -> (x/y=w585:dbl)
                n460 = Build Array(w568, w568) -> (w592:dbl[][])
                n461 = call "Convert to Dynamic Data5"("2D Array"=w609) -> ("Dynamic Data Type"=w608:dynamicdata)  [unwired: 3 in]
                n462 = call "Convert to Dynamic Data2"("2D Array"=w607) -> ("Dynamic Data Type"=w604:dynamicdata)  [unwired: 3 in]
                n463 = Divide(x=w613, y=1e+17) -> (x/y=→"Water Vapor Number Density":cdb[][])
                n464 = Divide(x=w600, y=1e+17) -> (x/y=→"Water Vapor Number Density 2":cdb[][])
                n465 = call "Convert to Dynamic Data6"("Array"=w568) -> ("Dynamic Data Type"=w569:dynamicdata)  [unwired: 3 in]
                n466 = To Long Integer(number=w586) -> (32bit integer=w584:i32)
                n467 = To Long Integer(number=w585) -> (32bit integer=w583:i32)
                n468 = call "Convert to Dynamic Data"("2D Array"=w592) -> ("Dynamic Data Type"=w605:dynamicdata)  [unwired: 3 in]
                n469 = call "Convert to Dynamic Data8"("2D Array"=w592) -> ("Dynamic Data Type"=w610:dynamicdata)  [unwired: 3 in]
                n470 = Decrement(x=w584) -> (x-1=w581:i32)
                n471 = Decrement(x=w583) -> (x-1=w582:i32)
                n472 = call "Build XY Graph"("Y Input"=w605, "X Input"=w604) -> ("XY Graph"=→"Water Vapor Number Density  2":cluster{"Y":dbl[], "Y":dbl[]}[])  [unwired: 3 in, 6 out]
                n473 = call "Build XY Graph3"("Y Input"=w610, "X Input"=w608) -> ("XY Graph"=→"Absolute Humidity":cluster{"Y":dbl[], "Y":dbl[]}[])  [unwired: 3 in, 6 out]
                n474 = Array Subset(array=w571, index=w581, length=w582) -> (w580:dbl[])
                n475 = Array Subset(array=w570, index=w581, length=w582) -> (w579:dbl[])
                n476 = call-poly <vilib>:"Mean.vi"("X"=w580) -> ("mean"=w578:dbl)  [unwired: 1 out]
                n477 = call-poly <vilib>:"Mean.vi"("X"=w579) -> ("mean"=w577:dbl)  [unwired: 1 out]
                n478 = Divide(x=w578, y=w577) -> (x/y=w576:dbl)
                n479 = Multiply(x=w570, y=w576) -> (x*y=w575:dbl[])
                n480 = Divide(x=w571, y=w575) -> (x/y=w574:dbl[])
                n481 = Natural Logarithm(1:w574) -> (0:w565:dbl[])
                n482 = Multiply(x=-1.0, y=w565) -> (x*y=w564:dbl[])
                n483 = call "Convert to Dynamic Data9"("Array"=w564) -> ("Dynamic Data Type"=w567:dynamicdata)  [unwired: 3 in]
                n484 = call "Build OD Plot"("Y Input"=w569, "X Input"=w567) -> ("XY Graph"=→"Optical Depth":cluster{"Y":dbl[], "Y":dbl[]}[])  [unwired: 3 in, 6 out]
              }
            }
          }
        }
        "L_Count" <- w99
      }
    }
  }
  n485 = case shown="True" w3 {
    frame False {
    }
    frame True {
      # "close data files"
      # "Close Bristol WM"
      n486 = local read "Ophir PM On/Off"() -> (w617:bool)
      n487 = local read "Bristol Out"() -> (w622:i32)
      n488 = local read "NF_Off_Ref"() -> (w618:refnum<file>)
      n489 = local read "NF_On_Ref"() -> (w619:refnum<file>)
      n490 = local read "FF_Off_Ref"() -> (w620:refnum<file>)
      n491 = local read "WS_On/Off"() -> (w616:bool)
      n492 = local read "FF_On_Ref"() -> (w621:refnum<file>)
      n493 = case shown="True" w616 {
        frame False {
        }
        frame True {
          n494 = local read "WS visa"() -> (w627:refnum<visa-resource-name>)
          n495 = local read "ID_out"() -> (w624:refnum<k5>)
          n496 = call "T_RH_P.vi"("VISA in"=w627, "WS_Commands"=enum16{"OpenWS", "ReadTRHP", "CloseWS"}."CloseWS") -> ()  [unwired: 11 in, 3 out]
          n497 = call "ADAM6018_2.1.vi"("ADAM6018_Command"=enum16{"Open_Adam", "Read_Adam", "Close_Adam"}."Close_Adam", "ID_in"=w624) -> ()  [unwired: 11 in, 3 out]
        }
      }
      n498 = case shown="True" w617 {
        frame False {
        }
        frame True {
          n499 = local read "OphirPM"() -> (w623:T7)
          n500 = call "OphirClose.vi"("OphirPM"=w623) -> ()  [unwired: 18 in, 1 out]
        }
      }
      n501 = dll-call lib="C:/H2O_DIAL/LabVIEW-2012/Bristol WM V2_31b/CLDevIFace.dll" fn="CLCloseDevice"("CommPort"=w622) -> ()  [unwired: 5 in, 2 out]
      n502 = Close File(refnum=w621) -> ()  [unwired: 1 in, 2 out]
      n503 = Close File(refnum=w620) -> ()  [unwired: 1 in, 2 out]
      n504 = Close File(refnum=w619) -> ()  [unwired: 1 in, 2 out]
      n505 = Close File(refnum=w618) -> ()  [unwired: 1 in, 2 out]
    }
  }
  "FileHour" <- -1 ("FileHour")
  "DataOpen" <- FALSE
